vi "XML Results.vi"(2 "XML":string="﻿<?xml version=\"1.0\" encoding=\"UTF-8\" standalone=\"no\"?><worksheet xmlns=\"http://schemas.mathsoft.com/worksheet50\" xmlns:xsi=\"http://www.w3.org/2001/XMLSchema-instance\" xmlns:ve=\"http://schemas.openxmlformats.org/markup-compatibility/2006\" xmlns:r=\"http://schemas.openxmlformats.org/officeDocument/2006/relationships\" xmlns:ws=\"http://schemas.mathsoft.com/worksheet50\" xmlns:ml=\"http://schemas.mathsoft.com/math50\" xmlns:u=\"http://schemas.mathsoft.com/units10\" xmlns:p=\"http://schemas.mathsoft.com/provenance10\"><regions><region top=\"57.6\" width=\"368\" left=\"9.6\" height=\"30\" converted-from=\"Mathcad14\" region-id=\"0\"><text><FlowDocument FontFamily=\"Tahoma\" FontStyle=\"Normal\" FontWeight=\"Normal\" FontSize=\"14.6666666666667\" Foreground=\"#FF000000\" Background=\"#00FFFFFF\" PagePadding=\"5,0,5,0\" AllowDrop=\"True\" Typography.Variants=\"Normal\" xmlns=\"http://schemas.microsoft.com/winfx/2006/xaml/presentation\"><Paragraph TextAlignment=\"Left\"><Run FontFamily=\"Arial\" FontStyle=\"Normal\" FontWeight=\"Bold\" FontSize=\"26.6666666666667\" Typography.Variants=\"Normal\"><Run.TextDecorations><TextDecoration Location=\"Underline\" /></Run.TextDecorations>AguaClara Design Tool</Run></Paragraph></FlowDocument></text></region><region top=\"124.8\" width=\"75\" left=\"48\" height=\"17\" converted-from=\"Mathcad14\" region-id=\"1\"><math><ml:eval><ml:id xml:space=\"preserve\">Country</ml:id><ml:result /></ml:eval></math></region><region top=\"153.6\" width=\"84\" left=\"48\" height=\"17\" converted-from=\"Mathcad14\" region-id=\"2\"><math><ml:eval><ml:id xml:space=\"preserve\">Language</ml:id><ml:result /></ml:eval></math></region><region top=\"153.6\" width=\"152\" left=\"288\" height=\"37\" converted-from=\"Mathcad14\" region-id=\"3\"><math><ml:define><ml:id label=\"Variable\" xml:space=\"preserve\"><Span xmlns=\"http://schemas.microsoft.com/winfx/2006/xaml/presentation\" xmlns:pw=\"clr-namespace:Ptc.Wpf;assembly=Ptc.Core\">C<pw:Subscript>ChlorineDoseMax</pw:Subscript></Span></ml:id><ml:apply><ml:mult /><ml:real>2</ml:real><ml:apply><ml:div /><ml:id xml:space=\"preserve\">mg</ml:id><ml:id xml:space=\"preserve\">L</ml:id></ml:apply></ml:apply></ml:define></math><mc14-conversion-loss-annotations><annotation>DisplayOperator</annotation></mc14-conversion-loss-annotations></region><region top=\"201.6\" width=\"138\" left=\"288\" height=\"37\" converted-from=\"Mathcad14\" region-id=\"4\"><math><ml:define><ml:id label=\"Variable\" xml:space=\"preserve\"><Span xmlns=\"http://schemas.microsoft.com/winfx/2006/xaml/presentation\" xmlns:pw=\"clr-namespace:Ptc.Wpf;assembly=Ptc.Core\">C<pw:Subscript>ChlorineStock</pw:Subscript></Span></ml:id><ml:apply><ml:mult /><ml:real>50</ml:real><ml:apply><ml:div /><ml:id xml:space=\"preserve\">gm</ml:id><ml:id xml:space=\"preserve\">L</ml:id></ml:apply></ml:apply></ml:define></math><mc14-conversion-loss-annotations><annotation>DisplayOperator</annotation></mc14-conversion-loss-annotations></region><region top=\"240\" width=\"131\" left=\"288\" height=\"22\" converted-from=\"Mathcad14\" region-id=\"5\"><math><ml:define><ml:id label=\"Variable\" xml:space=\"preserve\"><Span xmlns=\"http://schemas.microsoft.com/winfx/2006/xaml/presentation\" xmlns:pw=\"clr-namespace:Ptc.Wpf;assembly=Ptc.Core\">Ti<pw:Subscript>ChlorineStock</pw:Subscript></Span></ml:id><ml:apply><ml:mult /><ml:real>30</ml:real><ml:id xml:space=\"preserve\">hr</ml:id></ml:apply></ml:define></math><mc14-conversion-loss-annotations><annotation>DisplayOperator</annotation></mc14-conversion-loss-annotations></region><region top=\"268.8\" width=\"242.68\" left=\"422.4\" height=\"32\" converted-from=\"Mathcad14\" region-id=\"6\"><text><FlowDocument FontFamily=\"Tahoma\" FontStyle=\"Normal\" FontWeight=\"Normal\" FontSize=\"14.6666666666667\" Foreground=\"#FF000000\" Background=\"#00FFFFFF\" PagePadding=\"5,0,5,0\" AllowDrop=\"True\" Typography.Variants=\"Normal\" xmlns=\"http://schemas.microsoft.com/winfx/2006/xaml/presentation\"><Paragraph TextAlignment=\"Left\"><Run FontFamily=\"Arial\" FontStyle=\"Normal\" FontWeight=\"Normal\" FontSize=\"13.3333333333333\" Typography.Variants=\"Normal\"><Run.TextDecorations><TextDecorationCollection /></Run.TextDecorations>Needs to be redefined as zero until we create a database for all countries.</Run></Paragraph></FlowDocument></text></region><region top=\"278.4\" width=\"70\" left=\"288\" height=\"17\" converted-from=\"Mathcad14\" region-id=\"7\"><math><ml:define><ml:id label=\"Variable\" xml:space=\"preserve\">Country</ml:id><ml:real>0</ml:real></ml:define></math></region><region top=\"297.6\" width=\"172\" left=\"9.6\" height=\"24\" converted-from=\"Mathcad14\" region-id=\"8\"><text><FlowDocument FontFamily=\"Tahoma\" FontStyle=\"Normal\" FontWeight=\"Normal\" FontSize=\"14.6666666666667\" Foreground=\"#FF000000\" Background=\"#00FFFFFF\" PagePadding=\"5,0,5,0\" AllowDrop=\"True\" Typography.Variants=\"Normal\" xmlns=\"http://schemas.microsoft.com/winfx/2006/xaml/presentation\"><Paragraph TextAlignment=\"Left\"><Run FontFamily=\"Arial\" FontStyle=\"Normal\" FontWeight=\"Normal\" FontSize=\"21.3333333333333\" Typography.Variants=\"Normal\"><Run.TextDecorations><TextDecorationCollection /></Run.TextDecorations>References</Run></Paragraph></FlowDocument></text></region><region top=\"326.4\" width=\"832\" left=\"0\" height=\"19.2\" region-id=\"9\"><text is-text-block=\"true\"><FlowDocument FontFamily=\"Mathcad UniMath\" xmlns=\"http://schemas.microsoft.com/winfx/2006/xaml/presentation\"><Paragraph xml:space=\"preserve\">---↓  ---</Paragraph></FlowDocument></text><mc14-conversion-loss-annotations><annotation>Area</annotation></mc14-conversion-loss-annotations></region><region top=\"378.24\" width=\"215.68\" left=\"28.8\" height=\"16\" converted-from=\"Mathcad14\" region-id=\"10\"><text><FlowDocument FontFamily=\"Tahoma\" FontStyle=\"Normal\" FontWeight=\"Normal\" FontSize=\"14.6666666666667\" Foreground=\"#FF000000\" Background=\"#00FFFFFF\" PagePadding=\"5,0,5,0\" AllowDrop=\"True\" Typography.Variants=\"Normal\" xmlns=\"http://schemas.microsoft.com/winfx/2006/xaml/presentation\"><Paragraph TextAlignment=\"Left\"><Run FontFamily=\"Arial\" FontStyle=\"Normal\" FontWeight=\"Normal\" FontSize=\"13.3333333333333\" Typography.Variants=\"Normal\"><Run.TextDecorations><TextDecorationCollection /></Run.TextDecorations>MathCAD dimension calculations:</Run></Paragraph></FlowDocument></text></region><region top=\"416.639984\" width=\"488\" left=\"48\" height=\"14\" converted-from=\"Mathcad14\" region-id=\"11\"><reference used-cache=\"false\" last-saved-date=\"12/31/9999 23:59:59\" href=\"./BasicClientInputs.mcdx\" /><mc14-conversion-loss-annotations><annotation>IncludeWorksheet</annotation></mc14-conversion-loss-annotations></region><region top=\"435.84\" width=\"461\" left=\"48\" height=\"14\" converted-from=\"Mathcad14\" region-id=\"12\"><reference used-cache=\"false\" last-saved-date=\"12/31/9999 23:59:59\" href=\"./ExpertInputs.mcdx\" /><mc14-conversion-loss-annotations><annotation>IncludeWorksheet</annotation></mc14-conversion-loss-annotations></region><region top=\"455.039978\" width=\"476\" left=\"48\" height=\"14\" converted-from=\"Mathcad14\" region-id=\"13\"><reference used-cache=\"false\" last-saved-date=\"12/31/9999 23:59:59\" href=\"./MathFunctions.mcdx\" /><mc14-conversion-loss-annotations><annotation>IncludeWorksheet</annotation></mc14-conversion-loss-annotations></region><region top=\"474.24\" width=\"466\" left=\"48\" height=\"14\" converted-from=\"Mathcad14\" region-id=\"14\"><reference used-cache=\"false\" last-saved-date=\"12/31/9999 23:59:59\" href=\"./PipeDatabase.mcdx\" /><mc14-conversion-loss-annotations><annotation>IncludeWorksheet</annotation></mc14-conversion-loss-annotations></region><region top=\"493.44\" width=\"480\" left=\"48\" height=\"14\" converted-from=\"Mathcad14\" region-id=\"15\"><reference used-cache=\"false\" last-saved-date=\"12/31/9999 23:59:59\" href=\"./FluidsFunctions.mcdx\" /><mc14-conversion-loss-annotations><annotation>IncludeWorksheet</annotation></mc14-conversion-loss-annotations></region><region top=\"512.64\" width=\"496\" left=\"48\" height=\"14\" converted-from=\"Mathcad14\" region-id=\"16\"><reference used-cache=\"false\" last-saved-date=\"12/31/9999 23:59:59\" href=\"./SedimentationTank.mcdx\" /><mc14-conversion-loss-annotations><annotation>IncludeWorksheet</annotation></mc14-conversion-loss-annotations></region><region top=\"531.839966\" width=\"453\" left=\"48\" height=\"14\" converted-from=\"Mathcad14\" region-id=\"17\"><reference used-cache=\"false\" last-saved-date=\"12/31/9999 23:59:59\" href=\"./Flocculator.mcdx\" /><mc14-conversion-loss-annotations><annotation>IncludeWorksheet</annotation></mc14-conversion-loss-annotations></region><region top=\"551.04\" width=\"428\" left=\"48\" height=\"14\" converted-from=\"Mathcad14\" region-id=\"18\"><reference used-cache=\"false\" last-saved-date=\"12/31/9999 23:59:59\" href=\"./LFOM.mcdx\" /><mc14-conversion-loss-annotations><annotation>IncludeWorksheet</annotation></mc14-conversion-loss-annotations></region><region top=\"570.24\" width=\"447\" left=\"48\" height=\"14\" converted-from=\"Mathcad14\" region-id=\"19\"><reference used-cache=\"false\" last-saved-date=\"12/31/9999 23:59:59\" href=\"./LinearCdc.mcdx\" /><mc14-conversion-loss-annotations><annotation>IncludeWorksheet</annotation></mc14-conversion-loss-annotations></region><region top=\"589.44\" width=\"497\" left=\"48\" height=\"14\" converted-from=\"Mathcad14\" region-id=\"20\"><reference used-cache=\"false\" last-saved-date=\"12/31/9999 23:59:59\" href=\"./ChemStorageTanks.mcdx\" /><mc14-conversion-loss-annotations><annotation>IncludeWorksheet</annotation></mc14-conversion-loss-annotations></region><region top=\"608.64\" width=\"467\" left=\"48\" height=\"14\" converted-from=\"Mathcad14\" region-id=\"21\"><reference used-cache=\"false\" last-saved-date=\"12/31/9999 23:59:59\" href=\"./EntranceTank.mcdx\" /><mc14-conversion-loss-annotations><annotation>IncludeWorksheet</annotation></mc14-conversion-loss-annotations></region><region top=\"627.839966\" width=\"520\" left=\"48\" height=\"14\" converted-from=\"Mathcad14\" region-id=\"22\"><reference used-cache=\"false\" last-saved-date=\"12/31/9999 23:59:59\" href=\"./StackedRapidSandFilter.mcdx\" /><mc14-conversion-loss-annotations><annotation>IncludeWorksheet</annotation></mc14-conversion-loss-annotations></region><region top=\"647.04\" width=\"466\" left=\"48\" height=\"14\" converted-from=\"Mathcad14\" region-id=\"23\"><reference used-cache=\"false\" last-saved-date=\"12/31/9999 23:59:59\" href=\"./DrainChannel.mcdx\" /><mc14-conversion-loss-annotations><annotation>IncludeWorksheet</annotation></mc14-conversion-loss-annotations></region><region top=\"666.24\" width=\"463\" left=\"48\" height=\"14\" converted-from=\"Mathcad14\" region-id=\"24\"><reference used-cache=\"false\" last-saved-date=\"12/31/9999 23:59:59\" href=\"./MaterialsList.mcdx\" /><mc14-conversion-loss-annotations><annotation>IncludeWorksheet</annotation></mc14-conversion-loss-annotations></region><region top=\"704.64\" width=\"187.68\" left=\"28.8\" height=\"16\" converted-from=\"Mathcad14\" region-id=\"25\"><text><FlowDocument FontFamily=\"Tahoma\" FontStyle=\"Normal\" FontWeight=\"Normal\" FontSize=\"14.6666666666667\" Foreground=\"#FF000000\" Background=\"#00FFFFFF\" PagePadding=\"5,0,5,0\" AllowDrop=\"True\" Typography.Variants=\"Normal\" xmlns=\"http://schemas.microsoft.com/winfx/2006/xaml/presentation\"><Paragraph TextAlignment=\"Left\"><Run FontFamily=\"Arial\" FontStyle=\"Normal\" FontWeight=\"Normal\" FontSize=\"13.3333333333333\" Typography.Variants=\"Normal\"><Run.TextDecorations><TextDecorationCollection /></Run.TextDecorations>AutoCAD drawing programs:</Run></Paragraph></FlowDocument></text></region><region top=\"743.04\" width=\"125\" left=\"57.6\" height=\"18\" converted-from=\"Mathcad14\" region-id=\"26\"><text><FlowDocument FontFamily=\"Tahoma\" FontStyle=\"Normal\" FontWeight=\"Normal\" FontSize=\"14.6666666666667\" Foreground=\"#FF000000\" Background=\"#00FFFFFF\" PagePadding=\"5,0,5,0\" AllowDrop=\"True\" Typography.Variants=\"Normal\" xmlns=\"http://schemas.microsoft.com/winfx/2006/xaml/presentation\"><Paragraph TextAlignment=\"Left\"><Run FontFamily=\"Arial\" FontStyle=\"Normal\" FontWeight=\"Normal\" FontSize=\"16\" Typography.Variants=\"Normal\"><Run.TextDecorations><TextDecoration Location=\"Underline\" /></Run.TextDecorations>Translators:</Run><Run FontFamily=\"Arial\" FontStyle=\"Normal\" FontWeight=\"Normal\" FontSize=\"13.3333333333333\" Typography.Variants=\"Normal\" xml:space=\"preserve\"><Run.TextDecorations><TextDecorationCollection /></Run.TextDecorations> </Run></Paragraph></FlowDocument></text></region><region top=\"771.839966\" width=\"534\" left=\"57.6\" height=\"32\" converted-from=\"Mathcad14\" region-id=\"27\"><text><FlowDocument FontFamily=\"Tahoma\" FontStyle=\"Normal\" FontWeight=\"Normal\" FontSize=\"14.6666666666667\" Foreground=\"#FF000000\" Background=\"#00FFFFFF\" PagePadding=\"5,0,5,0\" AllowDrop=\"True\" Typography.Variants=\"Normal\" xmlns=\"http://schemas.microsoft.com/winfx/2006/xaml/presentation\"><Paragraph TextAlignment=\"Left\"><Run FontFamily=\"Arial\" FontStyle=\"Normal\" FontWeight=\"Normal\" FontSize=\"13.3333333333333\" Typography.Variants=\"Normal\"><Run.TextDecorations><TextDecorationCollection /></Run.TextDecorations>These are the codes that take MathCAD outputs and create AutoCAD scripts that are used to draw the plant (formerly Basics)</Run></Paragraph></FlowDocument></text></region><region top=\"800.64\" width=\"586\" left=\"48\" height=\"14\" converted-from=\"Mathcad14\" region-id=\"28\"><reference used-cache=\"false\" last-saved-date=\"12/31/9999 23:59:59\" href=\".\\AutoCAD Scripts\\MtoATranslators.mcdx\" /><mc14-conversion-loss-annotations><annotation>IncludeWorksheet</annotation></mc14-conversion-loss-annotations></region><region top=\"848.64\" width=\"558\" left=\"57.6\" height=\"64\" converted-from=\"Mathcad14\" region-id=\"29\"><text><FlowDocument FontFamily=\"Tahoma\" FontStyle=\"Normal\" FontWeight=\"Normal\" FontSize=\"14.6666666666667\" Foreground=\"#FF000000\" Background=\"#00FFFFFF\" PagePadding=\"5,0,5,0\" AllowDrop=\"True\" Typography.Variants=\"Normal\" xmlns=\"http://schemas.microsoft.com/winfx/2006/xaml/presentation\"><Paragraph TextAlignment=\"Left\"><Run FontFamily=\"Arial\" FontStyle=\"Normal\" FontWeight=\"Normal\" FontSize=\"13.3333333333333\" Typography.Variants=\"Normal\"><Run.TextDecorations><TextDecorationCollection /></Run.TextDecorations>The wrapped MtoA translator contains the functions that the user will want to access. These functions will draw pieces with full functionality - specifying the location, dimension, and orientation of the object. Also, it contains layer control and subtraction capabilities for grouped objects.</Run></Paragraph></FlowDocument></text></region><region top=\"915.84\" width=\"636\" left=\"48\" height=\"14\" converted-from=\"Mathcad14\" region-id=\"30\"><reference used-cache=\"false\" last-saved-date=\"12/31/9999 23:59:59\" href=\".\\AutoCAD Scripts\\MtoATranslatorsWrapped.mcdx\" /><mc14-conversion-loss-annotations><annotation>IncludeWorksheet</annotation></mc14-conversion-loss-annotations></region><region top=\"992.64\" width=\"172\" left=\"19.2\" height=\"18\" converted-from=\"Mathcad14\" region-id=\"31\"><text><FlowDocument FontFamily=\"Tahoma\" FontStyle=\"Normal\" FontWeight=\"Normal\" FontSize=\"14.6666666666667\" Foreground=\"#FF000000\" Background=\"#00FFFFFF\" PagePadding=\"5,0,5,0\" AllowDrop=\"True\" Typography.Variants=\"Normal\" xmlns=\"http://schemas.microsoft.com/winfx/2006/xaml/presentation\"><Paragraph TextAlignment=\"Left\"><Run FontFamily=\"Arial\" FontStyle=\"Normal\" FontWeight=\"Normal\" FontSize=\"16\" Typography.Variants=\"Normal\"><Run.TextDecorations><TextDecoration Location=\"Underline\" /></Run.TextDecorations>Drawing functions:</Run><Run FontFamily=\"Arial\" FontStyle=\"Normal\" FontWeight=\"Normal\" FontSize=\"13.3333333333333\" Typography.Variants=\"Normal\" xml:space=\"preserve\"><Run.TextDecorations><TextDecorationCollection /></Run.TextDecorations> </Run></Paragraph></FlowDocument></text></region><region top=\"1011.84\" width=\"543\" left=\"48\" height=\"14\" converted-from=\"Mathcad14\" region-id=\"32\"><reference used-cache=\"false\" last-saved-date=\"12/31/9999 23:59:59\" href=\".\\AutoCAD Scripts\\ChannelF.mcdx\" /><mc14-conversion-loss-annotations><annotation>IncludeWorksheet</annotation></mc14-conversion-loss-annotations></region><region top=\"1031.04\" width=\"549\" left=\"48\" height=\"14\" converted-from=\"Mathcad14\" region-id=\"33\"><reference used-cache=\"false\" last-saved-date=\"12/31/9999 23:59:59\" href=\".\\AutoCAD Scripts\\PlumbingF.mcdx\" /><mc14-conversion-loss-annotations><annotation>IncludeWorksheet</annotation></mc14-conversion-loss-annotations></region><region top=\"1050.24\" width=\"526\" left=\"48\" height=\"14\" converted-from=\"Mathcad14\" region-id=\"34\"><reference used-cache=\"false\" last-saved-date=\"12/31/9999 23:59:59\" href=\".\\AutoCAD Scripts\\TankF.mcdx\" /><mc14-conversion-loss-annotations><annotation>IncludeWorksheet</annotation></mc14-conversion-loss-annotations></region><region top=\"1069.44006\" width=\"529\" left=\"48\" height=\"14\" converted-from=\"Mathcad14\" region-id=\"35\"><reference used-cache=\"false\" last-saved-date=\"12/31/9999 23:59:59\" href=\".\\AutoCAD Scripts\\StairsF.mcdx\" /><mc14-conversion-loss-annotations><annotation>IncludeWorksheet</annotation></mc14-conversion-loss-annotations></region><region top=\"1088.64\" width=\"572\" left=\"48\" height=\"14\" converted-from=\"Mathcad14\" region-id=\"36\"><reference used-cache=\"false\" last-saved-date=\"12/31/9999 23:59:59\" href=\".\\AutoCAD Scripts\\DrainChannelF.mcdx\" /><mc14-conversion-loss-annotations><annotation>IncludeWorksheet</annotation></mc14-conversion-loss-annotations></region><region top=\"1165.44006\" width=\"184\" left=\"19.2\" height=\"18\" converted-from=\"Mathcad14\" region-id=\"37\"><text><FlowDocument FontFamily=\"Tahoma\" FontStyle=\"Normal\" FontWeight=\"Normal\" FontSize=\"14.6666666666667\" Foreground=\"#FF000000\" Background=\"#00FFFFFF\" PagePadding=\"5,0,5,0\" AllowDrop=\"True\" Typography.Variants=\"Normal\" xmlns=\"http://schemas.microsoft.com/winfx/2006/xaml/presentation\"><Paragraph TextAlignment=\"Left\"><Run FontFamily=\"Arial\" FontStyle=\"Normal\" FontWeight=\"Normal\" FontSize=\"16\" Typography.Variants=\"Normal\"><Run.TextDecorations><TextDecoration Location=\"Underline\" /></Run.TextDecorations>AutoCAD Script Files:</Run><Run FontFamily=\"Arial\" FontStyle=\"Normal\" FontWeight=\"Normal\" FontSize=\"13.3333333333333\" Typography.Variants=\"Normal\" xml:space=\"preserve\"><Run.TextDecorations><TextDecorationCollection /></Run.TextDecorations> </Run></Paragraph></FlowDocument></text></region><region top=\"1184.64\" width=\"570\" left=\"48\" height=\"14\" converted-from=\"Mathcad14\" region-id=\"38\"><reference used-cache=\"false\" last-saved-date=\"12/31/9999 23:59:59\" href=\".\\AutoCAD Scripts\\FlocculatorAC.mcdx\" /><mc14-conversion-loss-annotations><annotation>IncludeWorksheet</annotation></mc14-conversion-loss-annotations></region><region top=\"1203.84009\" width=\"613\" left=\"48\" height=\"14\" converted-from=\"Mathcad14\" region-id=\"39\"><reference used-cache=\"false\" last-saved-date=\"12/31/9999 23:59:59\" href=\".\\AutoCAD Scripts\\SedimentationTankAC.mcdx\" /><mc14-conversion-loss-annotations><annotation>IncludeWorksheet</annotation></mc14-conversion-loss-annotations></region><region top=\"1223.04\" width=\"584\" left=\"48\" height=\"14\" converted-from=\"Mathcad14\" region-id=\"40\"><reference used-cache=\"false\" last-saved-date=\"12/31/9999 23:59:59\" href=\".\\AutoCAD Scripts\\EntranceTankAC.mcdx\" /><mc14-conversion-loss-annotations><annotation>IncludeWorksheet</annotation></mc14-conversion-loss-annotations></region><region top=\"1242.24\" width=\"631\" left=\"48\" height=\"14\" converted-from=\"Mathcad14\" region-id=\"41\"><reference used-cache=\"false\" last-saved-date=\"12/31/9999 23:59:59\" href=\".\\AutoCAD Scripts\\ChemStockTanksACvlk24.mcdx\" /><mc14-conversion-loss-annotations><annotation>IncludeWorksheet</annotation></mc14-conversion-loss-annotations></region><region top=\"1261.44006\" width=\"583\" left=\"48\" height=\"14\" converted-from=\"Mathcad14\" region-id=\"42\"><reference used-cache=\"false\" last-saved-date=\"12/31/9999 23:59:59\" href=\".\\AutoCAD Scripts\\DrainChannelAC.mcdx\" /><mc14-conversion-loss-annotations><annotation>IncludeWorksheet</annotation></mc14-conversion-loss-annotations></region><region top=\"1280.64\" width=\"637\" left=\"48\" height=\"14\" converted-from=\"Mathcad14\" region-id=\"43\"><reference used-cache=\"false\" last-saved-date=\"12/31/9999 23:59:59\" href=\".\\AutoCAD Scripts\\StackedRapidSandFilterAC.mcdx\" /><mc14-conversion-loss-annotations><annotation>IncludeWorksheet</annotation></mc14-conversion-loss-annotations></region><region top=\"1299.84009\" width=\"559\" left=\"48\" height=\"14\" converted-from=\"Mathcad14\" region-id=\"44\"><reference used-cache=\"false\" last-saved-date=\"12/31/9999 23:59:59\" href=\".\\AutoCAD Scripts\\CdcACvlk24.mcdx\" /><mc14-conversion-loss-annotations><annotation>IncludeWorksheet</annotation></mc14-conversion-loss-annotations></region><region top=\"1319.04\" width=\"625\" left=\"48\" height=\"14\" converted-from=\"Mathcad14\" region-id=\"45\"><reference used-cache=\"false\" last-saved-date=\"12/31/9999 23:59:59\" href=\".\\AutoCAD Scripts\\OperatorAccessACvlk24.mcdx\" /><mc14-conversion-loss-annotations><annotation>IncludeWorksheet</annotation></mc14-conversion-loss-annotations></region><region top=\"1338.24\" width=\"560\" left=\"48\" height=\"14\" converted-from=\"Mathcad14\" region-id=\"46\"><reference used-cache=\"false\" last-saved-date=\"12/31/9999 23:59:59\" href=\".\\AutoCAD Scripts\\MaterialsAC.mcdx\" /><mc14-conversion-loss-annotations><annotation>IncludeWorksheet</annotation></mc14-conversion-loss-annotations></region><region top=\"1424.64\" width=\"77.08\" left=\"19.2\" height=\"18\" converted-from=\"Mathcad14\" region-id=\"47\"><text><FlowDocument FontFamily=\"Tahoma\" FontStyle=\"Normal\" FontWeight=\"Normal\" FontSize=\"14.6666666666667\" Foreground=\"#FF000000\" Background=\"#00FFFFFF\" PagePadding=\"5,0,5,0\" AllowDrop=\"True\" Typography.Variants=\"Normal\" xmlns=\"http://schemas.microsoft.com/winfx/2006/xaml/presentation\"><Paragraph TextAlignment=\"Left\"><Run FontFamily=\"Arial\" FontStyle=\"Normal\" FontWeight=\"Normal\" FontSize=\"16\" Typography.Variants=\"Normal\"><Run.TextDecorations><TextDecoration Location=\"Underline\" /></Run.TextDecorations>Layouts:</Run></Paragraph></FlowDocument></text></region><region top=\"1472.64\" width=\"297.76\" left=\"57.6\" height=\"16\" converted-from=\"Mathcad14\" region-id=\"48\"><text><FlowDocument FontFamily=\"Tahoma\" FontStyle=\"Normal\" FontWeight=\"Normal\" FontSize=\"14.6666666666667\" Foreground=\"#FF000000\" Background=\"#00FFFFFF\" PagePadding=\"5,0,5,0\" AllowDrop=\"True\" Typography.Variants=\"Normal\" xmlns=\"http://schemas.microsoft.com/winfx/2006/xaml/presentation\"><Paragraph TextAlignment=\"Left\"><Run FontFamily=\"Arial\" FontStyle=\"Normal\" FontWeight=\"Normal\" FontSize=\"13.3333333333333\" Typography.Variants=\"Normal\"><Run.TextDecorations><TextDecorationCollection /></Run.TextDecorations>This rearranges the plant to optimize the layout</Run></Paragraph></FlowDocument></text></region><region top=\"1491.84009\" width=\"581\" left=\"57.6\" height=\"14\" converted-from=\"Mathcad14\" region-id=\"49\"><reference used-cache=\"false\" last-saved-date=\"12/31/9999 23:59:59\" href=\".\\AutoCAD Scripts\\PlantLayoutsAC.mcdx\" /><mc14-conversion-loss-annotations><annotation>IncludeWorksheet</annotation></mc14-conversion-loss-annotations></region><region top=\"1549.44006\" width=\"466\" left=\"38.4\" height=\"32\" converted-from=\"Mathcad14\" region-id=\"50\"><text><FlowDocument FontFamily=\"Tahoma\" FontStyle=\"Normal\" FontWeight=\"Normal\" FontSize=\"14.6666666666667\" Foreground=\"#FF000000\" Background=\"#00FFFFFF\" PagePadding=\"5,0,5,0\" AllowDrop=\"True\" Typography.Variants=\"Normal\" xmlns=\"http://schemas.microsoft.com/winfx/2006/xaml/presentation\"><Paragraph TextAlignment=\"Left\"><Run FontFamily=\"Arial\" FontStyle=\"Normal\" FontWeight=\"Normal\" FontSize=\"13.3333333333333\" Typography.Variants=\"Normal\"><Run.TextDecorations><TextDecorationCollection /></Run.TextDecorations>This file will execute at the very end to create multiple views of the entire plant in paperspace</Run></Paragraph></FlowDocument></text></region><region top=\"1587.84009\" width=\"554\" left=\"48\" height=\"14\" converted-from=\"Mathcad14\" region-id=\"51\"><reference used-cache=\"false\" last-saved-date=\"12/31/9999 23:59:59\" href=\".\\AutoCAD Scripts\\LayoutsAC.mcdx\" /><mc14-conversion-loss-annotations><annotation>IncludeWorksheet</annotation></mc14-conversion-loss-annotations></region><region top=\"1687.44006\" width=\"832\" left=\"0\" height=\"19.2\" region-id=\"52\"><text is-text-block=\"true\"><FlowDocument FontFamily=\"Mathcad UniMath\" xmlns=\"http://schemas.microsoft.com/winfx/2006/xaml/presentation\"><Paragraph xml:space=\"preserve\">---↑  ---</Paragraph></FlowDocument></text></region><region top=\"1726.08008\" width=\"567\" left=\"19.2\" height=\"36\" converted-from=\"Mathcad14\" region-id=\"53\"><text><FlowDocument FontFamily=\"Tahoma\" FontStyle=\"Normal\" FontWeight=\"Normal\" FontSize=\"14.6666666666667\" Foreground=\"#FF000000\" Background=\"#00FFFFFF\" PagePadding=\"5,0,5,0\" AllowDrop=\"True\" Typography.Variants=\"Normal\" xmlns=\"http://schemas.microsoft.com/winfx/2006/xaml/presentation\"><Paragraph TextAlignment=\"Left\"><Run FontFamily=\"Arial\" FontStyle=\"Italic\" FontWeight=\"Bold\" FontSize=\"16\" Typography.Variants=\"Normal\" xml:space=\"preserve\"><Run.TextDecorations><TextDecorationCollection /></Run.TextDecorations>All variables displayed must have the standard SI units. They may not have units attached by the user. </Run></Paragraph></FlowDocument></text></region><region top=\"1850.88013\" width=\"301\" left=\"9.6\" height=\"19\" converted-from=\"Mathcad14\" region-id=\"54\"><text><FlowDocument FontFamily=\"Tahoma\" FontStyle=\"Normal\" FontWeight=\"Normal\" FontSize=\"14.6666666666667\" Foreground=\"#FF000000\" Background=\"#00FFFFFF\" PagePadding=\"5,0,5,0\" AllowDrop=\"True\" Typography.Variants=\"Normal\" xmlns=\"http://schemas.microsoft.com/winfx/2006/xaml/presentation\"><Paragraph TextAlignment=\"Left\"><Run FontFamily=\"Arial\" FontStyle=\"Normal\" FontWeight=\"Bold\" FontSize=\"16\" Foreground=\"#FF008000\" Typography.Variants=\"Normal\"><Run.TextDecorations><TextDecorationCollection /></Run.TextDecorations>General</Run></Paragraph></FlowDocument></text></region><region top=\"1860.4801\" width=\"832\" left=\"0\" height=\"19.2\" region-id=\"55\"><text is-text-block=\"true\"><FlowDocument FontFamily=\"Mathcad UniMath\" xmlns=\"http://schemas.microsoft.com/winfx/2006/xaml/presentation\"><Paragraph xml:space=\"preserve\">---↓  ---</Paragraph></FlowDocument></text><mc14-conversion-loss-annotations><annotation>CollapsedArea</annotation></mc14-conversion-loss-annotations></region><region top=\"1950.72009\" width=\"67\" left=\"38.4\" height=\"22\" converted-from=\"Mathcad14\" region-id=\"56\"><math><ml:eval><ml:id xml:space=\"preserve\"><Span xmlns=\"http://schemas.microsoft.com/winfx/2006/xaml/presentation\" xmlns:pw=\"clr-namespace:Ptc.Wpf;assembly=Ptc.Core\">Q<pw:Subscript>Plant</pw:Subscript></Span></ml:id><ml:result /></ml:eval></math></region><region top=\"1950.72009\" width=\"170\" left=\"345.6\" height=\"22\" converted-from=\"Mathcad14\" region-id=\"57\"><math resultRef=\"-2\"><ml:eval><ml:id xml:space=\"preserve\"><Span xmlns=\"http://schemas.microsoft.com/winfx/2006/xaml/presentation\" xmlns:pw=\"clr-namespace:Ptc.Wpf;assembly=Ptc.Core\">Pi<pw:Subscript>VenaContractaOrifice</pw:Subscript></Span></ml:id><ml:result /></ml:eval></math></region><region top=\"1998.72009\" width=\"92\" left=\"48\" height=\"22\" converted-from=\"Mathcad14\" region-id=\"58\"><math><ml:eval><ml:id xml:space=\"preserve\"><Span xmlns=\"http://schemas.microsoft.com/winfx/2006/xaml/presentation\" xmlns:pw=\"clr-namespace:Ptc.Wpf;assembly=Ptc.Core\">T<pw:Subscript>PlantWall</pw:Subscript></Span></ml:id><ml:result /></ml:eval></math></region><region top=\"2037.12012\" width=\"90\" left=\"364.8\" height=\"22\" converted-from=\"Mathcad14\" region-id=\"59\"><math><ml:eval><ml:id xml:space=\"preserve\"><Span xmlns=\"http://schemas.microsoft.com/winfx/2006/xaml/presentation\" xmlns:pw=\"clr-namespace:Ptc.Wpf;assembly=Ptc.Core\">W<pw:Subscript>SedPlate</pw:Subscript></Span></ml:id><ml:result /></ml:eval></math></region><region top=\"2046.72009\" width=\"109\" left=\"48\" height=\"22\" converted-from=\"Mathcad14\" region-id=\"60\"><math><ml:eval><ml:id xml:space=\"preserve\"><Span xmlns=\"http://schemas.microsoft.com/winfx/2006/xaml/presentation\" xmlns:pw=\"clr-namespace:Ptc.Wpf;assembly=Ptc.Core\">T<pw:Subscript>ConcreteMin</pw:Subscript></Span></ml:id><ml:result /></ml:eval></math></region><region top=\"2085.12\" width=\"114\" left=\"364.8\" height=\"22\" converted-from=\"Mathcad14\" region-id=\"61\"><math><ml:eval><ml:id xml:space=\"preserve\"><Span xmlns=\"http://schemas.microsoft.com/winfx/2006/xaml/presentation\" xmlns:pw=\"clr-namespace:Ptc.Wpf;assembly=Ptc.Core\">L<pw:Subscript>SedPlateSheet</pw:Subscript></Span></ml:id><ml:result /></ml:eval></math></region><region top=\"2094.72021\" width=\"98\" left=\"48\" height=\"22\" converted-from=\"Mathcad14\" region-id=\"62\"><math><ml:eval><ml:id xml:space=\"preserve\"><Span xmlns=\"http://schemas.microsoft.com/winfx/2006/xaml/presentation\" xmlns:pw=\"clr-namespace:Ptc.Wpf;assembly=Ptc.Core\">C<pw:Subscript>CoagStock</pw:Subscript></Span></ml:id><ml:result /></ml:eval></math></region><region top=\"2133.12\" width=\"85\" left=\"364.8\" height=\"22\" converted-from=\"Mathcad14\" region-id=\"63\"><math><ml:eval><ml:id xml:space=\"preserve\"><Span xmlns=\"http://schemas.microsoft.com/winfx/2006/xaml/presentation\" xmlns:pw=\"clr-namespace:Ptc.Wpf;assembly=Ptc.Core\">T<pw:Subscript>SedPlate</pw:Subscript></Span></ml:id><ml:result /></ml:eval></math></region><region top=\"2161.92017\" width=\"101\" left=\"48\" height=\"22\" converted-from=\"Mathcad14\" region-id=\"64\"><math><ml:eval><ml:id xml:space=\"preserve\"><Span xmlns=\"http://schemas.microsoft.com/winfx/2006/xaml/presentation\" xmlns:pw=\"clr-namespace:Ptc.Wpf;assembly=Ptc.Core\">Ti<pw:Subscript>CoagStock</pw:Subscript></Span></ml:id><ml:result /></ml:eval></math></region><region top=\"2181.12\" width=\"86\" left=\"364.8\" height=\"22\" converted-from=\"Mathcad14\" region-id=\"65\"><math><ml:eval><ml:id xml:space=\"preserve\"><Span xmlns=\"http://schemas.microsoft.com/winfx/2006/xaml/presentation\" xmlns:pw=\"clr-namespace:Ptc.Wpf;assembly=Ptc.Core\">T<pw:Subscript>SedWeir</pw:Subscript></Span></ml:id><ml:result /></ml:eval></math></region><region top=\"2209.92017\" width=\"142\" left=\"48\" height=\"45\" converted-from=\"Mathcad14\" region-id=\"66\"><math resultRef=\"-3\"><ml:eval><ml:id xml:space=\"preserve\"><Span xmlns=\"http://schemas.microsoft.com/winfx/2006/xaml/presentation\" xmlns:pw=\"clr-namespace:Ptc.Wpf;assembly=Ptc.Core\">C<pw:Subscript>ChlorineStock</pw:Subscript></Span></ml:id><ml:result /></ml:eval></math></region><region top=\"2229.12\" width=\"85\" left=\"364.8\" height=\"22\" converted-from=\"Mathcad14\" region-id=\"67\"><math><ml:eval><ml:id xml:space=\"preserve\"><Span xmlns=\"http://schemas.microsoft.com/winfx/2006/xaml/presentation\" xmlns:pw=\"clr-namespace:Ptc.Wpf;assembly=Ptc.Core\">W<pw:Subscript>SedBay</pw:Subscript></Span></ml:id><ml:result /></ml:eval></math></region><region top=\"2277.12\" width=\"174\" left=\"48\" height=\"30\" converted-from=\"Mathcad14\" region-id=\"68\"><math resultRef=\"-4\"><ml:eval><ml:id xml:space=\"preserve\"><Span xmlns=\"http://schemas.microsoft.com/winfx/2006/xaml/presentation\" xmlns:pw=\"clr-namespace:Ptc.Wpf;assembly=Ptc.Core\">Ti<pw:Subscript>ChlorineStock</pw:Subscript></Span></ml:id><ml:result /></ml:eval></math></region><region top=\"2277.12\" width=\"140\" left=\"374.4\" height=\"22\" converted-from=\"Mathcad14\" region-id=\"69\"><math resultRef=\"-5\"><ml:eval><ml:id xml:space=\"preserve\"><Span xmlns=\"http://schemas.microsoft.com/winfx/2006/xaml/presentation\" xmlns:pw=\"clr-namespace:Ptc.Wpf;assembly=Ptc.Core\">HL<pw:Subscript>ChannelMax</pw:Subscript></Span></ml:id><ml:result /></ml:eval></math></region><region top=\"2277.12\" width=\"106\" left=\"576\" height=\"48\" converted-from=\"Mathcad14\" region-id=\"70\"><text><FlowDocument FontFamily=\"Tahoma\" FontStyle=\"Normal\" FontWeight=\"Normal\" FontSize=\"14.6666666666667\" Foreground=\"#FF000000\" Background=\"#00FFFFFF\" PagePadding=\"5,0,5,0\" AllowDrop=\"True\" Typography.Variants=\"Normal\" xmlns=\"http://schemas.microsoft.com/winfx/2006/xaml/presentation\"><Paragraph TextAlignment=\"Left\"><Run FontFamily=\"Arial\" FontStyle=\"Normal\" FontWeight=\"Normal\" FontSize=\"13.3333333333333\" Typography.Variants=\"Normal\"><Run.TextDecorations><TextDecorationCollection /></Run.TextDecorations>Eliminate FCM variable from design specs</Run></Paragraph></FlowDocument></text></region><region top=\"2325.12\" width=\"142\" left=\"48\" height=\"22\" converted-from=\"Mathcad14\" region-id=\"71\"><math resultRef=\"-6\"><ml:eval><ml:id xml:space=\"preserve\"><Span xmlns=\"http://schemas.microsoft.com/winfx/2006/xaml/presentation\" xmlns:pw=\"clr-namespace:Ptc.Wpf;assembly=Ptc.Core\">H<pw:Subscript>PlantFreeboard</pw:Subscript></Span></ml:id><ml:result /></ml:eval></math></region><region top=\"2325.12\" width=\"102\" left=\"364.8\" height=\"22\" converted-from=\"Mathcad14\" region-id=\"72\"><math><ml:eval><ml:id xml:space=\"preserve\"><Span xmlns=\"http://schemas.microsoft.com/winfx/2006/xaml/presentation\" xmlns:pw=\"clr-namespace:Ptc.Wpf;assembly=Ptc.Core\">EN<pw:Subscript>DrillSeries</pw:Subscript></Span></ml:id><ml:result /></ml:eval></math></region><region top=\"2386.32\" width=\"832\" left=\"0\" height=\"19.2\" region-id=\"73\"><text is-text-block=\"true\"><FlowDocument FontFamily=\"Mathcad UniMath\" xmlns=\"http://schemas.microsoft.com/winfx/2006/xaml/presentation\"><Paragraph xml:space=\"preserve\">---↑  ---</Paragraph></FlowDocument></text></region><region top=\"2495.76\" width=\"301\" left=\"9.6\" height=\"19\" converted-from=\"Mathcad14\" region-id=\"74\"><text><FlowDocument FontFamily=\"Tahoma\" FontStyle=\"Normal\" FontWeight=\"Normal\" FontSize=\"14.6666666666667\" Foreground=\"#FF000000\" Background=\"#00FFFFFF\" PagePadding=\"5,0,5,0\" AllowDrop=\"True\" Typography.Variants=\"Normal\" xmlns=\"http://schemas.microsoft.com/winfx/2006/xaml/presentation\"><Paragraph TextAlignment=\"Left\"><Run FontFamily=\"Arial\" FontStyle=\"Normal\" FontWeight=\"Bold\" FontSize=\"16\" Foreground=\"#FF008000\" Typography.Variants=\"Normal\"><Run.TextDecorations><TextDecorationCollection /></Run.TextDecorations>Entrance Tank</Run></Paragraph></FlowDocument></text></region><region top=\"2505.35986\" width=\"832\" left=\"0\" height=\"19.2\" region-id=\"75\"><text is-text-block=\"true\"><FlowDocument FontFamily=\"Mathcad UniMath\" xmlns=\"http://schemas.microsoft.com/winfx/2006/xaml/presentation\"><Paragraph xml:space=\"preserve\">---↓  ---</Paragraph></FlowDocument></text><mc14-conversion-loss-annotations><annotation>CollapsedArea</annotation></mc14-conversion-loss-annotations></region><region top=\"2586\" width=\"124\" left=\"48\" height=\"37\" converted-from=\"Mathcad14\" region-id=\"76\"><math resultRef=\"-7\"><ml:eval><ml:id xml:space=\"preserve\"><Span xmlns=\"http://schemas.microsoft.com/winfx/2006/xaml/presentation\" xmlns:pw=\"clr-namespace:Ptc.Wpf;assembly=Ptc.Core\">V<pw:Subscript>EtUp</pw:Subscript></Span></ml:id><ml:result /></ml:eval></math></region><region top=\"2595.6\" width=\"97\" left=\"364.8\" height=\"22\" converted-from=\"Mathcad14\" region-id=\"77\"><math><ml:eval><ml:id xml:space=\"preserve\"><Span xmlns=\"http://schemas.microsoft.com/winfx/2006/xaml/presentation\" xmlns:pw=\"clr-namespace:Ptc.Wpf;assembly=Ptc.Core\">W<pw:Subscript>EtCapture</pw:Subscript></Span></ml:id><ml:result /></ml:eval></math></region><region top=\"2624.4\" width=\"145\" left=\"547.2\" height=\"22\" converted-from=\"Mathcad14\" region-id=\"78\"><math><ml:eval><ml:id xml:space=\"preserve\"><Span xmlns=\"http://schemas.microsoft.com/winfx/2006/xaml/presentation\" xmlns:pw=\"clr-namespace:Ptc.Wpf;assembly=Ptc.Core\">H<pw:Subscript>EtOverflowChannel</pw:Subscript></Span></ml:id><ml:result /></ml:eval></math></region><region top=\"2634\" width=\"51\" left=\"48\" height=\"22\" converted-from=\"Mathcad14\" region-id=\"79\"><math><ml:eval><ml:id xml:space=\"preserve\"><Span xmlns=\"http://schemas.microsoft.com/winfx/2006/xaml/presentation\" xmlns:pw=\"clr-namespace:Ptc.Wpf;assembly=Ptc.Core\">H<pw:Subscript>Et</pw:Subscript></Span></ml:id><ml:result /></ml:eval></math></region><region top=\"2672.4\" width=\"93\" left=\"57.6\" height=\"22\" converted-from=\"Mathcad14\" region-id=\"80\"><math resultRef=\"-8\"><ml:eval><ml:id xml:space=\"preserve\"><Span xmlns=\"http://schemas.microsoft.com/winfx/2006/xaml/presentation\" xmlns:pw=\"clr-namespace:Ptc.Wpf;assembly=Ptc.Core\">H<pw:Subscript>EtTop</pw:Subscript></Span></ml:id><ml:result /></ml:eval></math></region><region top=\"2672.4\" width=\"378.76\" left=\"192\" height=\"16\" converted-from=\"Mathcad14\" region-id=\"81\"><text><FlowDocument FontFamily=\"Tahoma\" FontStyle=\"Normal\" FontWeight=\"Normal\" FontSize=\"14.6666666666667\" Foreground=\"#FF000000\" Background=\"#00FFFFFF\" PagePadding=\"5,0,5,0\" AllowDrop=\"True\" Typography.Variants=\"Normal\" xmlns=\"http://schemas.microsoft.com/winfx/2006/xaml/presentation\"><Paragraph TextAlignment=\"Left\"><Run FontFamily=\"Arial\" FontStyle=\"Normal\" FontWeight=\"Normal\" FontSize=\"13.3333333333333\" Typography.Variants=\"Normal\"><Run.TextDecorations><TextDecorationCollection /></Run.TextDecorations>height of the top part of the entrance tank above the hoppers</Run></Paragraph></FlowDocument></text></region><region top=\"2710.8\" width=\"55\" left=\"48\" height=\"22\" converted-from=\"Mathcad14\" region-id=\"82\"><math><ml:eval><ml:id xml:space=\"preserve\"><Span xmlns=\"http://schemas.microsoft.com/winfx/2006/xaml/presentation\" xmlns:pw=\"clr-namespace:Ptc.Wpf;assembly=Ptc.Core\">W<pw:Subscript>Et</pw:Subscript></Span></ml:id><ml:result /></ml:eval></math></region><region top=\"2749.2\" width=\"49\" left=\"48\" height=\"22\" converted-from=\"Mathcad14\" region-id=\"83\"><math><ml:eval><ml:id xml:space=\"preserve\"><Span xmlns=\"http://schemas.microsoft.com/winfx/2006/xaml/presentation\" xmlns:pw=\"clr-namespace:Ptc.Wpf;assembly=Ptc.Core\">L<pw:Subscript>Et</pw:Subscript></Span></ml:id><ml:result /></ml:eval></math></region><region top=\"2768.4\" width=\"122\" left=\"480\" height=\"22\" converted-from=\"Mathcad14\" region-id=\"84\"><math resultRef=\"-9\"><ml:eval><ml:id xml:space=\"preserve\"><Span xmlns=\"http://schemas.microsoft.com/winfx/2006/xaml/presentation\" xmlns:pw=\"clr-namespace:Ptc.Wpf;assembly=Ptc.Core\">ND<pw:Subscript>EtDrain</pw:Subscript></Span></ml:id><ml:result /></ml:eval></math></region><region top=\"2768.4\" width=\"94\" left=\"700.8\" height=\"22\" converted-from=\"Mathcad14\" region-id=\"85\"><math resultRef=\"-10\"><ml:eval><ml:id xml:space=\"preserve\"><Span xmlns=\"http://schemas.microsoft.com/winfx/2006/xaml/presentation\" xmlns:pw=\"clr-namespace:Ptc.Wpf;assembly=Ptc.Core\">HL<pw:Subscript>Lfom</pw:Subscript></Span></ml:id><ml:result /></ml:eval></math></region><region top=\"2778\" width=\"63\" left=\"48\" height=\"22\" converted-from=\"Mathcad14\" region-id=\"86\"><math><ml:eval><ml:id xml:space=\"preserve\"><Span xmlns=\"http://schemas.microsoft.com/winfx/2006/xaml/presentation\" xmlns:pw=\"clr-namespace:Ptc.Wpf;assembly=Ptc.Core\">ZW<pw:Subscript>Et</pw:Subscript></Span></ml:id><ml:result /></ml:eval></math></region><region top=\"2806.8\" width=\"72\" left=\"48\" height=\"22\" converted-from=\"Mathcad14\" region-id=\"87\"><math><ml:eval><ml:id xml:space=\"preserve\"><Span xmlns=\"http://schemas.microsoft.com/winfx/2006/xaml/presentation\" xmlns:pw=\"clr-namespace:Ptc.Wpf;assembly=Ptc.Core\">Z<pw:Subscript>EtTop</pw:Subscript></Span></ml:id><ml:result /></ml:eval></math></region><region top=\"2835.6\" width=\"50\" left=\"48\" height=\"22\" converted-from=\"Mathcad14\" region-id=\"88\"><math><ml:eval><ml:id xml:space=\"preserve\"><Span xmlns=\"http://schemas.microsoft.com/winfx/2006/xaml/presentation\" xmlns:pw=\"clr-namespace:Ptc.Wpf;assembly=Ptc.Core\">Z<pw:Subscript>Et</pw:Subscript></Span></ml:id><ml:result /></ml:eval></math></region><region top=\"2835.6\" width=\"154.48\" left=\"201.6\" height=\"16\" converted-from=\"Mathcad14\" region-id=\"89\"><text><FlowDocument FontFamily=\"Tahoma\" FontStyle=\"Normal\" FontWeight=\"Normal\" FontSize=\"14.6666666666667\" Foreground=\"#FF000000\" Background=\"#00FFFFFF\" PagePadding=\"5,0,5,0\" AllowDrop=\"True\" Typography.Variants=\"Normal\" xmlns=\"http://schemas.microsoft.com/winfx/2006/xaml/presentation\"><Paragraph TextAlignment=\"Left\"><Run FontFamily=\"Arial\" FontStyle=\"Normal\" FontWeight=\"Normal\" FontSize=\"13.3333333333333\" Typography.Variants=\"Normal\"><Run.TextDecorations><TextDecorationCollection /></Run.TextDecorations>elevation of top of slab.</Run></Paragraph></FlowDocument></text></region><region top=\"2864.4\" width=\"93\" left=\"480\" height=\"22\" converted-from=\"Mathcad14\" region-id=\"90\"><math><ml:eval><ml:id xml:space=\"preserve\"><Span xmlns=\"http://schemas.microsoft.com/winfx/2006/xaml/presentation\" xmlns:pw=\"clr-namespace:Ptc.Wpf;assembly=Ptc.Core\">ND<pw:Subscript>RMPipe</pw:Subscript></Span></ml:id><ml:result /></ml:eval></math></region><region top=\"2874\" width=\"91\" left=\"57.6\" height=\"22\" converted-from=\"Mathcad14\" region-id=\"91\"><math><ml:eval><ml:id xml:space=\"preserve\"><Span xmlns=\"http://schemas.microsoft.com/winfx/2006/xaml/presentation\" xmlns:pw=\"clr-namespace:Ptc.Wpf;assembly=Ptc.Core\">Z<pw:Subscript>EtHopper</pw:Subscript></Span></ml:id><ml:result /></ml:eval></math></region><region top=\"2912.4\" width=\"92\" left=\"480\" height=\"22\" converted-from=\"Mathcad14\" region-id=\"92\"><math><ml:eval><ml:id xml:space=\"preserve\"><Span xmlns=\"http://schemas.microsoft.com/winfx/2006/xaml/presentation\" xmlns:pw=\"clr-namespace:Ptc.Wpf;assembly=Ptc.Core\">H<pw:Subscript>EtHopper</pw:Subscript></Span></ml:id><ml:result /></ml:eval></math></region><region top=\"2922\" width=\"98\" left=\"57.6\" height=\"22\" converted-from=\"Mathcad14\" region-id=\"93\"><math><ml:eval><ml:id xml:space=\"preserve\"><Span xmlns=\"http://schemas.microsoft.com/winfx/2006/xaml/presentation\" xmlns:pw=\"clr-namespace:Ptc.Wpf;assembly=Ptc.Core\">N<pw:Subscript>EtHoppers</pw:Subscript></Span></ml:id><ml:result /></ml:eval></math></region><region top=\"2950.8\" width=\"128\" left=\"720\" height=\"22\" converted-from=\"Mathcad14\" region-id=\"94\"><math><ml:eval><ml:id xml:space=\"preserve\"><Span xmlns=\"http://schemas.microsoft.com/winfx/2006/xaml/presentation\" xmlns:pw=\"clr-namespace:Ptc.Wpf;assembly=Ptc.Core\">ND<pw:Subscript>EtFlowControl</pw:Subscript></Span></ml:id><ml:result /></ml:eval></math></region><region top=\"2960.4\" width=\"90\" left=\"480\" height=\"22\" converted-from=\"Mathcad14\" region-id=\"95\"><math><ml:eval><ml:id xml:space=\"preserve\"><Span xmlns=\"http://schemas.microsoft.com/winfx/2006/xaml/presentation\" xmlns:pw=\"clr-namespace:Ptc.Wpf;assembly=Ptc.Core\">L<pw:Subscript>EtHopper</pw:Subscript></Span></ml:id><ml:result /></ml:eval></math></region><region top=\"2979.6\" width=\"91\" left=\"57.6\" height=\"22\" converted-from=\"Mathcad14\" region-id=\"96\"><math><ml:eval><ml:id xml:space=\"preserve\"><Span xmlns=\"http://schemas.microsoft.com/winfx/2006/xaml/presentation\" xmlns:pw=\"clr-namespace:Ptc.Wpf;assembly=Ptc.Core\">AN<pw:Subscript>EtSlope</pw:Subscript></Span></ml:id><ml:result /></ml:eval></math></region><region top=\"3027.6\" width=\"72\" left=\"57.6\" height=\"22\" converted-from=\"Mathcad14\" region-id=\"97\"><math><ml:eval><ml:id xml:space=\"preserve\"><Span xmlns=\"http://schemas.microsoft.com/winfx/2006/xaml/presentation\" xmlns:pw=\"clr-namespace:Ptc.Wpf;assembly=Ptc.Core\">W<pw:Subscript>EtDC</pw:Subscript></Span></ml:id><ml:result /></ml:eval></math></region><region top=\"3027.6\" width=\"291.28\" left=\"192\" height=\"16\" converted-from=\"Mathcad14\" region-id=\"98\"><text><FlowDocument FontFamily=\"Tahoma\" FontStyle=\"Normal\" FontWeight=\"Normal\" FontSize=\"14.6666666666667\" Foreground=\"#FF000000\" Background=\"#00FFFFFF\" PagePadding=\"5,0,5,0\" AllowDrop=\"True\" Typography.Variants=\"Normal\" xmlns=\"http://schemas.microsoft.com/winfx/2006/xaml/presentation\"><Paragraph TextAlignment=\"Left\"><Run FontFamily=\"Arial\" FontStyle=\"Normal\" FontWeight=\"Normal\" FontSize=\"13.3333333333333\" Typography.Variants=\"Normal\"><Run.TextDecorations><TextDecorationCollection /></Run.TextDecorations>drain channel under entrance tank dimensions</Run></Paragraph></FlowDocument></text></region><region top=\"3056.4\" width=\"66\" left=\"57.6\" height=\"22\" converted-from=\"Mathcad14\" region-id=\"99\"><math><ml:eval><ml:id xml:space=\"preserve\"><Span xmlns=\"http://schemas.microsoft.com/winfx/2006/xaml/presentation\" xmlns:pw=\"clr-namespace:Ptc.Wpf;assembly=Ptc.Core\">L<pw:Subscript>EtDC</pw:Subscript></Span></ml:id><ml:result /></ml:eval></math></region><region top=\"3094.8\" width=\"327\" left=\"307.2\" height=\"32\" converted-from=\"Mathcad14\" region-id=\"100\"><text><FlowDocument FontFamily=\"Tahoma\" FontStyle=\"Normal\" FontWeight=\"Normal\" FontSize=\"14.6666666666667\" Foreground=\"#FF000000\" Background=\"#00FFFFFF\" PagePadding=\"5,0,5,0\" AllowDrop=\"True\" Typography.Variants=\"Normal\" xmlns=\"http://schemas.microsoft.com/winfx/2006/xaml/presentation\"><Paragraph TextAlignment=\"Left\"><Run FontFamily=\"Arial\" FontStyle=\"Normal\" FontWeight=\"Normal\" FontSize=\"13.3333333333333\" Typography.Variants=\"Normal\"><Run.TextDecorations><TextDecorationCollection /></Run.TextDecorations>Give heights of the channel at the beginning and end and change the design specs to explain that it's sloped.</Run></Paragraph></FlowDocument></text></region><region top=\"3104.4\" width=\"68\" left=\"57.6\" height=\"22\" converted-from=\"Mathcad14\" region-id=\"101\"><math><ml:eval><ml:id xml:space=\"preserve\"><Span xmlns=\"http://schemas.microsoft.com/winfx/2006/xaml/presentation\" xmlns:pw=\"clr-namespace:Ptc.Wpf;assembly=Ptc.Core\">H<pw:Subscript>EtDC</pw:Subscript></Span></ml:id><ml:result /></ml:eval></math></region><region top=\"3152.4\" width=\"129.4\" left=\"9.6\" height=\"16\" converted-from=\"Mathcad14\" region-id=\"102\"><text><FlowDocument FontFamily=\"Tahoma\" FontStyle=\"Normal\" FontWeight=\"Normal\" FontSize=\"14.6666666666667\" Foreground=\"#FF000000\" Background=\"#00FFFFFF\" PagePadding=\"5,0,5,0\" AllowDrop=\"True\" Typography.Variants=\"Normal\" xmlns=\"http://schemas.microsoft.com/winfx/2006/xaml/presentation\"><Paragraph TextAlignment=\"Left\"><Run FontFamily=\"Arial\" FontStyle=\"Normal\" FontWeight=\"Normal\" FontSize=\"13.3333333333333\" Typography.Variants=\"Normal\"><Run.TextDecorations><TextDecorationCollection /></Run.TextDecorations>Flow measurement</Run></Paragraph></FlowDocument></text></region><region top=\"3200.4\" width=\"108\" left=\"38.4\" height=\"22\" converted-from=\"Mathcad14\" region-id=\"103\"><math><ml:eval><ml:id xml:space=\"preserve\"><Span xmlns=\"http://schemas.microsoft.com/winfx/2006/xaml/presentation\" xmlns:pw=\"clr-namespace:Ptc.Wpf;assembly=Ptc.Core\">D<pw:Subscript>LfomOrifices</pw:Subscript></Span></ml:id><ml:result /></ml:eval></math></region><region top=\"3248.4\" width=\"121\" left=\"38.4\" height=\"22\" converted-from=\"Mathcad14\" region-id=\"104\"><math resultRef=\"-11\"><ml:eval><ml:id xml:space=\"preserve\"><Span xmlns=\"http://schemas.microsoft.com/winfx/2006/xaml/presentation\" xmlns:pw=\"clr-namespace:Ptc.Wpf;assembly=Ptc.Core\">S<pw:Subscript>LfomRows</pw:Subscript></Span></ml:id><ml:result /></ml:eval></math></region><region top=\"3421.2\" width=\"102\" left=\"336\" height=\"22\" converted-from=\"Mathcad14\" region-id=\"105\"><math><ml:eval><ml:id xml:space=\"preserve\"><Span xmlns=\"http://schemas.microsoft.com/winfx/2006/xaml/presentation\" xmlns:pw=\"clr-namespace:Ptc.Wpf;assembly=Ptc.Core\">H<pw:Subscript>LfomOrifice</pw:Subscript></Span></ml:id><ml:result /></ml:eval><resultFormat><table /></resultFormat></math></region><region top=\"3421.2\" width=\"95\" left=\"604.8\" height=\"22\" converted-from=\"Mathcad14\" region-id=\"106\"><math><ml:eval><ml:id xml:space=\"preserve\"><Span xmlns=\"http://schemas.microsoft.com/winfx/2006/xaml/presentation\" xmlns:pw=\"clr-namespace:Ptc.Wpf;assembly=Ptc.Core\">Q<pw:Subscript>LfomScale</pw:Subscript></Span></ml:id><ml:result /></ml:eval><resultFormat><table /></resultFormat></math></region><region top=\"3430.8\" width=\"109\" left=\"48\" height=\"22\" converted-from=\"Mathcad14\" region-id=\"107\"><math><ml:eval><ml:id xml:space=\"preserve\"><Span xmlns=\"http://schemas.microsoft.com/winfx/2006/xaml/presentation\" xmlns:pw=\"clr-namespace:Ptc.Wpf;assembly=Ptc.Core\">N<pw:Subscript>LfomOrifices</pw:Subscript></Span></ml:id><ml:result /></ml:eval><resultFormat><table /></resultFormat></math></region><region top=\"3594\" width=\"77\" left=\"28.8\" height=\"22\" converted-from=\"Mathcad14\" region-id=\"108\"><math><ml:eval><ml:id xml:space=\"preserve\"><Span xmlns=\"http://schemas.microsoft.com/winfx/2006/xaml/presentation\" xmlns:pw=\"clr-namespace:Ptc.Wpf;assembly=Ptc.Core\">ND<pw:Subscript>Lfom</pw:Subscript></Span></ml:id><ml:result /></ml:eval></math></region><region top=\"3622.8\" width=\"94\" left=\"403.2\" height=\"22\" converted-from=\"Mathcad14\" region-id=\"109\"><math resultRef=\"-12\"><ml:eval><ml:id xml:space=\"preserve\"><Span xmlns=\"http://schemas.microsoft.com/winfx/2006/xaml/presentation\" xmlns:pw=\"clr-namespace:Ptc.Wpf;assembly=Ptc.Core\">HL<pw:Subscript>Lfom</pw:Subscript></Span></ml:id><ml:result /></ml:eval></math></region><region top=\"3651.6\" width=\"75.92\" left=\"28.8\" height=\"16\" converted-from=\"Mathcad14\" region-id=\"110\"><text><FlowDocument FontFamily=\"Tahoma\" FontStyle=\"Normal\" FontWeight=\"Normal\" FontSize=\"14.6666666666667\" Foreground=\"#FF000000\" Background=\"#00FFFFFF\" PagePadding=\"5,0,5,0\" AllowDrop=\"True\" Typography.Variants=\"Normal\" xmlns=\"http://schemas.microsoft.com/winfx/2006/xaml/presentation\"><Paragraph TextAlignment=\"Left\"><Run FontFamily=\"Arial\" FontStyle=\"Normal\" FontWeight=\"Normal\" FontSize=\"13.3333333333333\" Typography.Variants=\"Normal\"><Run.TextDecorations><TextDecorationCollection /></Run.TextDecorations>Rapid Mix</Run></Paragraph></FlowDocument></text></region><region top=\"3709.2\" width=\"68\" left=\"38.4\" height=\"22\" converted-from=\"Mathcad14\" region-id=\"111\"><math><ml:eval><ml:id xml:space=\"preserve\"><Span xmlns=\"http://schemas.microsoft.com/winfx/2006/xaml/presentation\" xmlns:pw=\"clr-namespace:Ptc.Wpf;assembly=Ptc.Core\">ED<pw:Subscript>Tee</pw:Subscript></Span></ml:id><ml:result /></ml:eval></math></region><region top=\"3795.6\" width=\"162.4\" left=\"201.6\" height=\"16\" converted-from=\"Mathcad14\" region-id=\"112\"><text><FlowDocument FontFamily=\"Tahoma\" FontStyle=\"Normal\" FontWeight=\"Normal\" FontSize=\"14.6666666666667\" Foreground=\"#FF000000\" Background=\"#00FFFFFF\" PagePadding=\"5,0,5,0\" AllowDrop=\"True\" Typography.Variants=\"Normal\" xmlns=\"http://schemas.microsoft.com/winfx/2006/xaml/presentation\"><Paragraph TextAlignment=\"Left\"><Run FontFamily=\"Arial\" FontStyle=\"Normal\" FontWeight=\"Normal\" FontSize=\"13.3333333333333\" Typography.Variants=\"Normal\" xml:space=\"preserve\"><Run.TextDecorations><TextDecorationCollection /></Run.TextDecorations>elevation of the center of </Run></Paragraph></FlowDocument></text></region><region top=\"3805.2\" width=\"107\" left=\"9.6\" height=\"22\" converted-from=\"Mathcad14\" region-id=\"113\"><math><ml:eval><ml:id xml:space=\"preserve\"><Span xmlns=\"http://schemas.microsoft.com/winfx/2006/xaml/presentation\" xmlns:pw=\"clr-namespace:Ptc.Wpf;assembly=Ptc.Core\">Z<pw:Subscript>LfomOrifices</pw:Subscript></Span></ml:id><ml:result /></ml:eval></math></region><region top=\"3834\" width=\"69\" left=\"9.6\" height=\"22\" converted-from=\"Mathcad14\" region-id=\"114\"><math><ml:eval><ml:id xml:space=\"preserve\"><Span xmlns=\"http://schemas.microsoft.com/winfx/2006/xaml/presentation\" xmlns:pw=\"clr-namespace:Ptc.Wpf;assembly=Ptc.Core\">Z<pw:Subscript>EtExit</pw:Subscript></Span></ml:id><ml:result /></ml:eval></math></region><region top=\"3834\" width=\"527.52\" left=\"201.6\" height=\"32\" converted-from=\"Mathcad14\" region-id=\"115\"><text><FlowDocument FontFamily=\"Tahoma\" FontStyle=\"Normal\" FontWeight=\"Normal\" FontSize=\"14.6666666666667\" Foreground=\"#FF000000\" Background=\"#00FFFFFF\" PagePadding=\"5,0,5,0\" AllowDrop=\"True\" Typography.Variants=\"Normal\" xmlns=\"http://schemas.microsoft.com/winfx/2006/xaml/presentation\"><Paragraph TextAlignment=\"Left\"><Run FontFamily=\"Arial\" FontStyle=\"Normal\" FontWeight=\"Normal\" FontSize=\"13.3333333333333\" Typography.Variants=\"Normal\"><Run.TextDecorations><TextDecorationCollection /></Run.TextDecorations>elevation of center of pipe exiting the entrance tank and heading toward the flocculator</Run></Paragraph></FlowDocument></text></region><region top=\"3914.4\" width=\"832\" left=\"0\" height=\"19.2\" region-id=\"116\"><text is-text-block=\"true\"><FlowDocument FontFamily=\"Mathcad UniMath\" xmlns=\"http://schemas.microsoft.com/winfx/2006/xaml/presentation\"><Paragraph xml:space=\"preserve\">---↑  ---</Paragraph></FlowDocument></text></region><region top=\"4043.03979\" width=\"832\" left=\"0\" height=\"19.2\" region-id=\"117\"><text is-text-block=\"true\"><FlowDocument FontFamily=\"Mathcad UniMath\" xmlns=\"http://schemas.microsoft.com/winfx/2006/xaml/presentation\"><Paragraph xml:space=\"preserve\">---↓  ---</Paragraph></FlowDocument></text><mc14-conversion-loss-annotations><annotation>CollapsedArea</annotation></mc14-conversion-loss-annotations></region><region top=\"4114.07959\" width=\"72\" left=\"28.8\" height=\"22\" converted-from=\"Mathcad14\" region-id=\"118\"><math resultRef=\"-13\"><ml:eval><ml:id xml:space=\"preserve\"><Span xmlns=\"http://schemas.microsoft.com/winfx/2006/xaml/presentation\" xmlns:pw=\"clr-namespace:Ptc.Wpf;assembly=Ptc.Core\">W<pw:Subscript>DC</pw:Subscript></Span></ml:id><ml:result /></ml:eval></math></region><region top=\"4133.28\" width=\"398\" left=\"201.6\" height=\"48\" converted-from=\"Mathcad14\" region-id=\"119\"><text><FlowDocument FontFamily=\"Tahoma\" FontStyle=\"Normal\" FontWeight=\"Normal\" FontSize=\"14.6666666666667\" Foreground=\"#FF000000\" Background=\"#00FFFFFF\" PagePadding=\"5,0,5,0\" AllowDrop=\"True\" Typography.Variants=\"Normal\" xmlns=\"http://schemas.microsoft.com/winfx/2006/xaml/presentation\"><Paragraph TextAlignment=\"Left\"><Run FontFamily=\"Arial\" FontStyle=\"Normal\" FontWeight=\"Normal\" FontSize=\"13.3333333333333\" Typography.Variants=\"Normal\"><Run.TextDecorations><TextDecorationCollection /></Run.TextDecorations>Maybe give the vertical distances below the bottom of the sed tank of the beginning and end of the channel? Calculate them, display, and add to the design specs.</Run></Paragraph></FlowDocument></text></region><region top=\"4152.47949\" width=\"57\" left=\"28.8\" height=\"22\" converted-from=\"Mathcad14\" region-id=\"120\"><math><ml:eval><ml:id xml:space=\"preserve\"><Span xmlns=\"http://schemas.microsoft.com/winfx/2006/xaml/presentation\" xmlns:pw=\"clr-namespace:Ptc.Wpf;assembly=Ptc.Core\">H<pw:Subscript>DC</pw:Subscript></Span></ml:id><ml:result /></ml:eval></math></region><region top=\"4190.88\" width=\"55\" left=\"28.8\" height=\"22\" converted-from=\"Mathcad14\" region-id=\"121\"><math><ml:eval><ml:id xml:space=\"preserve\"><Span xmlns=\"http://schemas.microsoft.com/winfx/2006/xaml/presentation\" xmlns:pw=\"clr-namespace:Ptc.Wpf;assembly=Ptc.Core\">L<pw:Subscript>DC</pw:Subscript></Span></ml:id><ml:result /></ml:eval></math></region><region top=\"4252.07959\" width=\"832\" left=\"0\" height=\"19.2\" region-id=\"122\"><text is-text-block=\"true\"><FlowDocument FontFamily=\"Mathcad UniMath\" xmlns=\"http://schemas.microsoft.com/winfx/2006/xaml/presentation\"><Paragraph xml:space=\"preserve\">---↑  ---</Paragraph></FlowDocument></text></region><region top=\"4275.12\" width=\"310\" left=\"9.6\" height=\"19\" converted-from=\"Mathcad14\" region-id=\"123\"><text><FlowDocument FontFamily=\"Tahoma\" FontStyle=\"Normal\" FontWeight=\"Normal\" FontSize=\"14.6666666666667\" Foreground=\"#FF000000\" Background=\"#00FFFFFF\" PagePadding=\"5,0,5,0\" AllowDrop=\"True\" Typography.Variants=\"Normal\" xmlns=\"http://schemas.microsoft.com/winfx/2006/xaml/presentation\"><Paragraph TextAlignment=\"Left\"><Run FontFamily=\"Arial\" FontStyle=\"Normal\" FontWeight=\"Bold\" FontSize=\"16\" Foreground=\"#FF008000\" Typography.Variants=\"Normal\"><Run.TextDecorations><TextDecorationCollection /></Run.TextDecorations>Plant Drain Channel</Run></Paragraph></FlowDocument></text></region><region top=\"4371.12\" width=\"832\" left=\"0\" height=\"19.2\" region-id=\"124\"><text is-text-block=\"true\"><FlowDocument FontFamily=\"Mathcad UniMath\" xmlns=\"http://schemas.microsoft.com/winfx/2006/xaml/presentation\"><Paragraph xml:space=\"preserve\">---↓  ---</Paragraph></FlowDocument></text><mc14-conversion-loss-annotations><annotation>CollapsedArea</annotation></mc14-conversion-loss-annotations></region><region top=\"4432.55957\" width=\"95\" left=\"28.8\" height=\"22\" converted-from=\"Mathcad14\" region-id=\"125\"><math><ml:eval><ml:id xml:space=\"preserve\"><Span xmlns=\"http://schemas.microsoft.com/winfx/2006/xaml/presentation\" xmlns:pw=\"clr-namespace:Ptc.Wpf;assembly=Ptc.Core\">Z<pw:Subscript>CoagTank</pw:Subscript></Span></ml:id><ml:result /></ml:eval></math></region><region top=\"4480.55957\" width=\"127\" left=\"28.8\" height=\"22\" converted-from=\"Mathcad14\" region-id=\"126\"><math><ml:eval><ml:id xml:space=\"preserve\"><Span xmlns=\"http://schemas.microsoft.com/winfx/2006/xaml/presentation\" xmlns:pw=\"clr-namespace:Ptc.Wpf;assembly=Ptc.Core\">Z<pw:Subscript>CoagTankOutlet</pw:Subscript></Span></ml:id><ml:result /></ml:eval></math></region><region top=\"4528.55957\" width=\"141\" left=\"28.8\" height=\"22\" converted-from=\"Mathcad14\" region-id=\"127\"><math resultRef=\"-14\"><ml:eval><ml:id xml:space=\"preserve\"><Span xmlns=\"http://schemas.microsoft.com/winfx/2006/xaml/presentation\" xmlns:pw=\"clr-namespace:Ptc.Wpf;assembly=Ptc.Core\">L<pw:Subscript>CdcFloatArm</pw:Subscript></Span></ml:id><ml:result /></ml:eval></math></region><region top=\"4547.76\" width=\"84\" left=\"316.8\" height=\"22\" converted-from=\"Mathcad14\" region-id=\"128\"><math><ml:eval><ml:id xml:space=\"preserve\"><Span xmlns=\"http://schemas.microsoft.com/winfx/2006/xaml/presentation\" xmlns:pw=\"clr-namespace:Ptc.Wpf;assembly=Ptc.Core\">Q<pw:Subscript>CdcMax</pw:Subscript></Span></ml:id><ml:result /></ml:eval></math></region><region top=\"4576.55957\" width=\"142\" left=\"28.8\" height=\"22\" converted-from=\"Mathcad14\" region-id=\"129\"><math resultRef=\"-15\"><ml:eval><ml:id xml:space=\"preserve\"><Span xmlns=\"http://schemas.microsoft.com/winfx/2006/xaml/presentation\" xmlns:pw=\"clr-namespace:Ptc.Wpf;assembly=Ptc.Core\">L<pw:Subscript>CdcScaleArm</pw:Subscript></Span></ml:id><ml:result /></ml:eval></math></region><region top=\"4595.76\" width=\"154\" left=\"614.4\" height=\"45\" converted-from=\"Mathcad14\" region-id=\"130\"><math resultRef=\"-16\"><ml:eval><ml:id xml:space=\"preserve\"><Span xmlns=\"http://schemas.microsoft.com/winfx/2006/xaml/presentation\" xmlns:pw=\"clr-namespace:Ptc.Wpf;assembly=Ptc.Core\">C<pw:Subscript>CoagDoseMax</pw:Subscript></Span></ml:id><ml:result /></ml:eval></math></region><region top=\"4624.55957\" width=\"122\" left=\"28.8\" height=\"22\" converted-from=\"Mathcad14\" region-id=\"131\"><math resultRef=\"-17\"><ml:eval><ml:id xml:space=\"preserve\"><Span xmlns=\"http://schemas.microsoft.com/winfx/2006/xaml/presentation\" xmlns:pw=\"clr-namespace:Ptc.Wpf;assembly=Ptc.Core\">B<pw:Subscript>StockOutlet</pw:Subscript></Span></ml:id><ml:result /></ml:eval></math></region><region top=\"4701.36\" width=\"115\" left=\"316.8\" height=\"22\" converted-from=\"Mathcad14\" region-id=\"132\"><math><ml:eval><ml:id xml:space=\"preserve\"><Span xmlns=\"http://schemas.microsoft.com/winfx/2006/xaml/presentation\" xmlns:pw=\"clr-namespace:Ptc.Wpf;assembly=Ptc.Core\">L<pw:Subscript>CoagCdcTube</pw:Subscript></Span></ml:id><ml:result /></ml:eval></math></region><region top=\"4720.55957\" width=\"164\" left=\"28.8\" height=\"30\" converted-from=\"Mathcad14\" region-id=\"133\"><math resultRef=\"-18\"><ml:eval><ml:id xml:space=\"preserve\"><Span xmlns=\"http://schemas.microsoft.com/winfx/2006/xaml/presentation\" xmlns:pw=\"clr-namespace:Ptc.Wpf;assembly=Ptc.Core\">D<pw:Subscript>CdcTube</pw:Subscript></Span></ml:id><ml:result /></ml:eval></math></region><region top=\"4758.96\" width=\"124\" left=\"28.8\" height=\"22\" converted-from=\"Mathcad14\" region-id=\"134\"><math><ml:eval><ml:id xml:space=\"preserve\"><Span xmlns=\"http://schemas.microsoft.com/winfx/2006/xaml/presentation\" xmlns:pw=\"clr-namespace:Ptc.Wpf;assembly=Ptc.Core\">N<pw:Subscript>CoagCdcTubes</pw:Subscript></Span></ml:id><ml:result /></ml:eval></math></region><region top=\"4797.36\" width=\"88\" left=\"374.4\" height=\"22\" converted-from=\"Mathcad14\" region-id=\"135\"><math resultRef=\"-19\"><ml:eval><ml:id xml:space=\"preserve\"><Span xmlns=\"http://schemas.microsoft.com/winfx/2006/xaml/presentation\" xmlns:pw=\"clr-namespace:Ptc.Wpf;assembly=Ptc.Core\">HL<pw:Subscript>Cdc</pw:Subscript></Span></ml:id><ml:result /></ml:eval></math></region><region top=\"4806.96\" width=\"141\" left=\"28.8\" height=\"22\" converted-from=\"Mathcad14\" region-id=\"136\"><math resultRef=\"-20\"><ml:eval><ml:id xml:space=\"preserve\"><Span xmlns=\"http://schemas.microsoft.com/winfx/2006/xaml/presentation\" xmlns:pw=\"clr-namespace:Ptc.Wpf;assembly=Ptc.Core\">L<pw:Subscript>CdcFloatArm</pw:Subscript></Span></ml:id><ml:result /></ml:eval></math></region><region top=\"4845.36\" width=\"142\" left=\"28.8\" height=\"22\" converted-from=\"Mathcad14\" region-id=\"137\"><math resultRef=\"-21\"><ml:eval><ml:id xml:space=\"preserve\"><Span xmlns=\"http://schemas.microsoft.com/winfx/2006/xaml/presentation\" xmlns:pw=\"clr-namespace:Ptc.Wpf;assembly=Ptc.Core\">L<pw:Subscript>CdcScaleArm</pw:Subscript></Span></ml:id><ml:result /></ml:eval></math></region><region top=\"4973.76\" width=\"832\" left=\"0\" height=\"19.2\" region-id=\"138\"><text is-text-block=\"true\"><FlowDocument FontFamily=\"Mathcad UniMath\" xmlns=\"http://schemas.microsoft.com/winfx/2006/xaml/presentation\"><Paragraph xml:space=\"preserve\">---↑  ---</Paragraph></FlowDocument></text></region><region top=\"4996.8\" width=\"310\" left=\"9.6\" height=\"19\" converted-from=\"Mathcad14\" region-id=\"139\"><text><FlowDocument FontFamily=\"Tahoma\" FontStyle=\"Normal\" FontWeight=\"Normal\" FontSize=\"14.6666666666667\" Foreground=\"#FF000000\" Background=\"#00FFFFFF\" PagePadding=\"5,0,5,0\" AllowDrop=\"True\" Typography.Variants=\"Normal\" xmlns=\"http://schemas.microsoft.com/winfx/2006/xaml/presentation\"><Paragraph Margin=\"0,0,0,0\" TextAlignment=\"Left\"><Run FontFamily=\"Arial\" FontStyle=\"Normal\" FontWeight=\"Bold\" FontSize=\"16\" Foreground=\"#FF008000\" Typography.Variants=\"Normal\"><Run.TextDecorations><TextDecorationCollection /></Run.TextDecorations>Coag Dose Controller</Run></Paragraph></FlowDocument></text></region><region top=\"5092.8\" width=\"103.36\" left=\"9.6\" height=\"19\" converted-from=\"Mathcad14\" region-id=\"140\"><text><FlowDocument FontFamily=\"Tahoma\" FontStyle=\"Normal\" FontWeight=\"Normal\" FontSize=\"14.6666666666667\" Foreground=\"#FF000000\" Background=\"#00FFFFFF\" PagePadding=\"5,0,5,0\" AllowDrop=\"True\" Typography.Variants=\"Normal\" xmlns=\"http://schemas.microsoft.com/winfx/2006/xaml/presentation\"><Paragraph TextAlignment=\"Left\"><Run FontFamily=\"Arial\" FontStyle=\"Normal\" FontWeight=\"Bold\" FontSize=\"16\" Foreground=\"#FF008000\" Typography.Variants=\"Normal\"><Run.TextDecorations><TextDecorationCollection /></Run.TextDecorations>Flocculator</Run></Paragraph></FlowDocument></text></region><region top=\"5102.4\" width=\"832\" left=\"0\" height=\"19.2\" region-id=\"141\"><text is-text-block=\"true\"><FlowDocument FontFamily=\"Mathcad UniMath\" xmlns=\"http://schemas.microsoft.com/winfx/2006/xaml/presentation\"><Paragraph xml:space=\"preserve\">---↓  ---</Paragraph></FlowDocument></text><mc14-conversion-loss-annotations><annotation>CollapsedArea</annotation></mc14-conversion-loss-annotations></region><region top=\"5163.84\" width=\"240.52\" left=\"681.6\" height=\"16\" converted-from=\"Mathcad14\" region-id=\"142\"><text><FlowDocument FontFamily=\"Tahoma\" FontStyle=\"Normal\" FontWeight=\"Normal\" FontSize=\"14.6666666666667\" Foreground=\"#FF000000\" Background=\"#00FFFFFF\" PagePadding=\"5,0,5,0\" AllowDrop=\"True\" Typography.Variants=\"Normal\" xmlns=\"http://schemas.microsoft.com/winfx/2006/xaml/presentation\"><Paragraph TextAlignment=\"Left\"><Run FontFamily=\"Arial\" FontStyle=\"Normal\" FontWeight=\"Normal\" FontSize=\"13.3333333333333\" Typography.Variants=\"Normal\"><Run.TextDecorations><TextDecorationCollection /></Run.TextDecorations>Look at Flocculator Positioning arrays</Run></Paragraph></FlowDocument></text></region><region top=\"5173.44\" width=\"63\" left=\"19.2\" height=\"22\" converted-from=\"Mathcad14\" region-id=\"143\"><math><ml:eval><ml:id xml:space=\"preserve\"><Span xmlns=\"http://schemas.microsoft.com/winfx/2006/xaml/presentation\" xmlns:pw=\"clr-namespace:Ptc.Wpf;assembly=Ptc.Core\">H<pw:Subscript>Floc</pw:Subscript></Span></ml:id><ml:result /></ml:eval></math></region><region top=\"5173.44\" width=\"90\" left=\"230.4\" height=\"22\" converted-from=\"Mathcad14\" region-id=\"144\"><math><ml:eval><ml:id xml:space=\"preserve\"><Span xmlns=\"http://schemas.microsoft.com/winfx/2006/xaml/presentation\" xmlns:pw=\"clr-namespace:Ptc.Wpf;assembly=Ptc.Core\">Z<pw:Subscript>FlocTank</pw:Subscript></Span></ml:id><ml:result /></ml:eval></math></region><region top=\"5202.23975\" width=\"100\" left=\"432\" height=\"22\" converted-from=\"Mathcad14\" region-id=\"145\"><math><ml:eval><ml:id xml:space=\"preserve\"><Span xmlns=\"http://schemas.microsoft.com/winfx/2006/xaml/presentation\" xmlns:pw=\"clr-namespace:Ptc.Wpf;assembly=Ptc.Core\">N<pw:Subscript>FlocValves</pw:Subscript></Span></ml:id><ml:result /></ml:eval></math></region><region top=\"5221.44\" width=\"112\" left=\"19.2\" height=\"22\" converted-from=\"Mathcad14\" region-id=\"146\"><math><ml:eval><ml:id xml:space=\"preserve\"><Span xmlns=\"http://schemas.microsoft.com/winfx/2006/xaml/presentation\" xmlns:pw=\"clr-namespace:Ptc.Wpf;assembly=Ptc.Core\">W<pw:Subscript>FlocChannel</pw:Subscript></Span></ml:id><ml:result /></ml:eval></math></region><region top=\"5221.44\" width=\"290.2\" left=\"748.8\" height=\"16\" converted-from=\"Mathcad14\" region-id=\"147\"><text><FlowDocument FontFamily=\"Tahoma\" FontStyle=\"Normal\" FontWeight=\"Normal\" FontSize=\"14.6666666666667\" Foreground=\"#FF000000\" Background=\"#00FFFFFF\" PagePadding=\"5,0,5,0\" AllowDrop=\"True\" Typography.Variants=\"Normal\" xmlns=\"http://schemas.microsoft.com/winfx/2006/xaml/presentation\"><Paragraph TextAlignment=\"Left\"><Run FontFamily=\"Arial\" FontStyle=\"Normal\" FontWeight=\"Normal\" FontSize=\"13.3333333333333\" Typography.Variants=\"Normal\"><Run.TextDecorations><TextDecorationCollection /></Run.TextDecorations>Fill last channel with bafffles from last channel</Run></Paragraph></FlowDocument></text></region><region top=\"5231.04\" width=\"65\" left=\"240\" height=\"22\" converted-from=\"Mathcad14\" region-id=\"148\"><math><ml:eval><ml:id xml:space=\"preserve\"><Span xmlns=\"http://schemas.microsoft.com/winfx/2006/xaml/presentation\" xmlns:pw=\"clr-namespace:Ptc.Wpf;assembly=Ptc.Core\">Ti<pw:Subscript>Floc</pw:Subscript></Span></ml:id><ml:result /></ml:eval></math></region><region top=\"5240.63965\" width=\"93\" left=\"441.6\" height=\"22\" converted-from=\"Mathcad14\" region-id=\"149\"><math><ml:eval><ml:id xml:space=\"preserve\"><Span xmlns=\"http://schemas.microsoft.com/winfx/2006/xaml/presentation\" xmlns:pw=\"clr-namespace:Ptc.Wpf;assembly=Ptc.Core\">H<pw:Subscript>FlocSlope</pw:Subscript></Span></ml:id><ml:result /></ml:eval></math></region><region top=\"5240.63965\" width=\"391.96\" left=\"748.8\" height=\"16\" converted-from=\"Mathcad14\" region-id=\"150\"><text><FlowDocument FontFamily=\"Tahoma\" FontStyle=\"Normal\" FontWeight=\"Normal\" FontSize=\"14.6666666666667\" Foreground=\"#FF000000\" Background=\"#00FFFFFF\" PagePadding=\"5,0,5,0\" AllowDrop=\"True\" Typography.Variants=\"Normal\" xmlns=\"http://schemas.microsoft.com/winfx/2006/xaml/presentation\"><Paragraph TextAlignment=\"Left\"><Run FontFamily=\"Arial\" FontStyle=\"Normal\" FontWeight=\"Normal\" FontSize=\"13.3333333333333\" Typography.Variants=\"Normal\"><Run.TextDecorations><TextDecorationCollection /></Run.TextDecorations>Fix port width to be based on energy dissipation in that channel</Run></Paragraph></FlowDocument></text></region><region top=\"5259.84\" width=\"395.14\" left=\"748.8\" height=\"16\" converted-from=\"Mathcad14\" region-id=\"151\"><text><FlowDocument FontFamily=\"Tahoma\" FontStyle=\"Normal\" FontWeight=\"Normal\" FontSize=\"14.6666666666667\" Foreground=\"#FF000000\" Background=\"#00FFFFFF\" PagePadding=\"5,0,5,0\" AllowDrop=\"True\" Typography.Variants=\"Normal\" xmlns=\"http://schemas.microsoft.com/winfx/2006/xaml/presentation\"><Paragraph TextAlignment=\"Left\"><Run FontFamily=\"Arial\" FontStyle=\"Normal\" FontWeight=\"Normal\" FontSize=\"13.3333333333333\" Typography.Variants=\"Normal\"><Run.TextDecorations><TextDecorationCollection /></Run.TextDecorations>Adjust spacing after the number of baffles per channel is known.</Run></Paragraph></FlowDocument></text></region><region top=\"5269.44\" width=\"107\" left=\"19.2\" height=\"53\" converted-from=\"Mathcad14\" region-id=\"152\"><math resultRef=\"-22\"><ml:eval><ml:id xml:space=\"preserve\"><Span xmlns=\"http://schemas.microsoft.com/winfx/2006/xaml/presentation\" xmlns:pw=\"clr-namespace:Ptc.Wpf;assembly=Ptc.Core\">ED<pw:Subscript>Floc</pw:Subscript></Span></ml:id><ml:result /></ml:eval></math></region><region top=\"5279.04\" width=\"62\" left=\"240\" height=\"22\" converted-from=\"Mathcad14\" region-id=\"153\"><math><ml:eval><ml:id xml:space=\"preserve\"><Span xmlns=\"http://schemas.microsoft.com/winfx/2006/xaml/presentation\" xmlns:pw=\"clr-namespace:Ptc.Wpf;assembly=Ptc.Core\">V<pw:Subscript>Floc</pw:Subscript></Span></ml:id><ml:result /></ml:eval></math></region><region top=\"5279.04\" width=\"442.88\" left=\"748.8\" height=\"16\" converted-from=\"Mathcad14\" region-id=\"154\"><text><FlowDocument FontFamily=\"Tahoma\" FontStyle=\"Normal\" FontWeight=\"Normal\" FontSize=\"14.6666666666667\" Foreground=\"#FF000000\" Background=\"#00FFFFFF\" PagePadding=\"5,0,5,0\" AllowDrop=\"True\" Typography.Variants=\"Normal\" xmlns=\"http://schemas.microsoft.com/winfx/2006/xaml/presentation\"><Paragraph TextAlignment=\"Left\"><Run FontFamily=\"Arial\" FontStyle=\"Normal\" FontWeight=\"Normal\" FontSize=\"13.3333333333333\" Typography.Variants=\"Normal\" xml:space=\"preserve\"><Run.TextDecorations><TextDecorationCollection /></Run.TextDecorations>Check the residence time of the flocculator should be at least 20minutes </Run></Paragraph></FlowDocument></text></region><region top=\"5317.44\" width=\"98\" left=\"19.2\" height=\"22\" converted-from=\"Mathcad14\" region-id=\"155\"><math><ml:eval><ml:id xml:space=\"preserve\"><Span xmlns=\"http://schemas.microsoft.com/winfx/2006/xaml/presentation\" xmlns:pw=\"clr-namespace:Ptc.Wpf;assembly=Ptc.Core\">HW<pw:Subscript>FlocEnd</pw:Subscript></Span></ml:id><ml:result /></ml:eval></math></region><region top=\"5336.63965\" width=\"103\" left=\"259.2\" height=\"22\" converted-from=\"Mathcad14\" region-id=\"156\"><math><ml:eval><ml:id xml:space=\"preserve\"><Span xmlns=\"http://schemas.microsoft.com/winfx/2006/xaml/presentation\" xmlns:pw=\"clr-namespace:Ptc.Wpf;assembly=Ptc.Core\">ND<pw:Subscript>FlocValve</pw:Subscript></Span></ml:id><ml:result /></ml:eval></math></region><region top=\"5355.84\" width=\"113\" left=\"28.8\" height=\"30\" converted-from=\"Mathcad14\" region-id=\"157\"><math resultRef=\"-23\"><ml:eval><ml:id xml:space=\"preserve\"><Span xmlns=\"http://schemas.microsoft.com/winfx/2006/xaml/presentation\" xmlns:pw=\"clr-namespace:Ptc.Wpf;assembly=Ptc.Core\">CP<pw:Subscript>Floc</pw:Subscript></Span></ml:id><ml:result /></ml:eval></math></region><region top=\"5384.63965\" width=\"144\" left=\"259.2\" height=\"30\" converted-from=\"Mathcad14\" region-id=\"158\"><math resultRef=\"-24\"><ml:eval><ml:id xml:space=\"preserve\"><Span xmlns=\"http://schemas.microsoft.com/winfx/2006/xaml/presentation\" xmlns:pw=\"clr-namespace:Ptc.Wpf;assembly=Ptc.Core\">Ti<pw:Subscript>FlocDrain</pw:Subscript></Span></ml:id><ml:result /></ml:eval></math></region><region top=\"5403.84\" width=\"98\" left=\"28.8\" height=\"22\" converted-from=\"Mathcad14\" region-id=\"159\"><math><ml:eval><ml:id xml:space=\"preserve\"><Span xmlns=\"http://schemas.microsoft.com/winfx/2006/xaml/presentation\" xmlns:pw=\"clr-namespace:Ptc.Wpf;assembly=Ptc.Core\">CP<pw:Subscript>FlocTotal</pw:Subscript></Span></ml:id><ml:result /></ml:eval></math></region><region top=\"5461.44\" width=\"114\" left=\"19.2\" height=\"22\" converted-from=\"Mathcad14\" region-id=\"160\"><math><ml:eval><ml:id xml:space=\"preserve\"><Span xmlns=\"http://schemas.microsoft.com/winfx/2006/xaml/presentation\" xmlns:pw=\"clr-namespace:Ptc.Wpf;assembly=Ptc.Core\">N<pw:Subscript>FlocChannels</pw:Subscript></Span></ml:id><ml:result /></ml:eval></math></region><region top=\"5461.44\" width=\"62\" left=\"268.8\" height=\"22\" converted-from=\"Mathcad14\" region-id=\"161\"><math><ml:eval><ml:id xml:space=\"preserve\"><Span xmlns=\"http://schemas.microsoft.com/winfx/2006/xaml/presentation\" xmlns:pw=\"clr-namespace:Ptc.Wpf;assembly=Ptc.Core\">G<pw:Subscript>Floc</pw:Subscript></Span></ml:id><ml:result /></ml:eval></math></region><region top=\"5499.84\" width=\"89\" left=\"19.2\" height=\"22\" converted-from=\"Mathcad14\" region-id=\"162\"><math><ml:eval><ml:id xml:space=\"preserve\"><Span xmlns=\"http://schemas.microsoft.com/winfx/2006/xaml/presentation\" xmlns:pw=\"clr-namespace:Ptc.Wpf;assembly=Ptc.Core\">L<pw:Subscript>FlocTank</pw:Subscript></Span></ml:id><ml:result /></ml:eval></math></region><region top=\"5547.84\" width=\"70\" left=\"19.2\" height=\"22\" converted-from=\"Mathcad14\" region-id=\"163\"><math><ml:eval><ml:id xml:space=\"preserve\"><Span xmlns=\"http://schemas.microsoft.com/winfx/2006/xaml/presentation\" xmlns:pw=\"clr-namespace:Ptc.Wpf;assembly=Ptc.Core\">HL<pw:Subscript>Floc</pw:Subscript></Span></ml:id><ml:result /></ml:eval></math></region><region top=\"5547.84\" width=\"139\" left=\"268.8\" height=\"22\" converted-from=\"Mathcad14\" region-id=\"164\"><math><ml:eval><ml:id xml:space=\"preserve\"><Span xmlns=\"http://schemas.microsoft.com/winfx/2006/xaml/presentation\" xmlns:pw=\"clr-namespace:Ptc.Wpf;assembly=Ptc.Core\">ED<pw:Subscript>FlocChannelFirst</pw:Subscript></Span></ml:id><ml:result /></ml:eval></math></region><region top=\"5605.44\" width=\"101\" left=\"19.2\" height=\"22\" converted-from=\"Mathcad14\" region-id=\"165\"><math><ml:eval><ml:id xml:space=\"preserve\"><Span xmlns=\"http://schemas.microsoft.com/winfx/2006/xaml/presentation\" xmlns:pw=\"clr-namespace:Ptc.Wpf;assembly=Ptc.Core\">HW<pw:Subscript>FlocStart</pw:Subscript></Span></ml:id><ml:result /></ml:eval></math></region><region top=\"5720.63965\" width=\"92\" left=\"28.8\" height=\"22\" converted-from=\"Mathcad14\" region-id=\"166\"><math><ml:eval><ml:id xml:space=\"preserve\"><Span xmlns=\"http://schemas.microsoft.com/winfx/2006/xaml/presentation\" xmlns:pw=\"clr-namespace:Ptc.Wpf;assembly=Ptc.Core\">S<pw:Subscript>FlocBaffle</pw:Subscript></Span></ml:id><ml:result /></ml:eval></math></region><region top=\"5720.63965\" width=\"93\" left=\"240\" height=\"22\" converted-from=\"Mathcad14\" region-id=\"167\"><math><ml:eval><ml:id xml:space=\"preserve\"><Span xmlns=\"http://schemas.microsoft.com/winfx/2006/xaml/presentation\" xmlns:pw=\"clr-namespace:Ptc.Wpf;assembly=Ptc.Core\">B<pw:Subscript>FlocBaffle</pw:Subscript></Span></ml:id><ml:result /></ml:eval></math></region><region top=\"5720.63965\" width=\"145\" left=\"470.4\" height=\"22\" converted-from=\"Mathcad14\" region-id=\"168\"><math><ml:eval><ml:id xml:space=\"preserve\"><Span xmlns=\"http://schemas.microsoft.com/winfx/2006/xaml/presentation\" xmlns:pw=\"clr-namespace:Ptc.Wpf;assembly=Ptc.Core\">N<pw:Subscript>FlocChannelBaffles</pw:Subscript></Span></ml:id><ml:result /></ml:eval></math></region><region top=\"5720.63965\" width=\"89\" left=\"720\" height=\"22\" converted-from=\"Mathcad14\" region-id=\"169\"><math><ml:eval><ml:id xml:space=\"preserve\"><Span xmlns=\"http://schemas.microsoft.com/winfx/2006/xaml/presentation\" xmlns:pw=\"clr-namespace:Ptc.Wpf;assembly=Ptc.Core\">W<pw:Subscript>FlocPort</pw:Subscript></Span></ml:id><ml:result /></ml:eval></math></region><region top=\"5797.44\" width=\"116\" left=\"28.8\" height=\"22\" converted-from=\"Mathcad14\" region-id=\"170\"><math><ml:eval><ml:id xml:space=\"preserve\"><Span xmlns=\"http://schemas.microsoft.com/winfx/2006/xaml/presentation\" xmlns:pw=\"clr-namespace:Ptc.Wpf;assembly=Ptc.Core\">S<pw:Subscript>FlocBaffleFirst</pw:Subscript></Span></ml:id><ml:result /></ml:eval></math></region><region top=\"5912.63965\" width=\"120\" left=\"28.8\" height=\"22\" converted-from=\"Mathcad14\" region-id=\"171\"><math><ml:eval><ml:id xml:space=\"preserve\"><Span xmlns=\"http://schemas.microsoft.com/winfx/2006/xaml/presentation\" xmlns:pw=\"clr-namespace:Ptc.Wpf;assembly=Ptc.Core\">HL<pw:Subscript>FlocChannels</pw:Subscript></Span></ml:id><ml:result /></ml:eval></math></region><region top=\"5912.63965\" width=\"126\" left=\"268.8\" height=\"22\" converted-from=\"Mathcad14\" region-id=\"172\"><math><ml:eval><ml:id xml:space=\"preserve\"><Span xmlns=\"http://schemas.microsoft.com/winfx/2006/xaml/presentation\" xmlns:pw=\"clr-namespace:Ptc.Wpf;assembly=Ptc.Core\">L<pw:Subscript>FlocBaffleLower</pw:Subscript></Span></ml:id><ml:result /></ml:eval></math></region><region top=\"5912.63965\" width=\"126\" left=\"508.8\" height=\"22\" converted-from=\"Mathcad14\" region-id=\"173\"><math><ml:eval><ml:id xml:space=\"preserve\"><Span xmlns=\"http://schemas.microsoft.com/winfx/2006/xaml/presentation\" xmlns:pw=\"clr-namespace:Ptc.Wpf;assembly=Ptc.Core\">L<pw:Subscript>FlocBaffleUpper</pw:Subscript></Span></ml:id><ml:result /></ml:eval></math></region><region top=\"5912.63965\" width=\"85\" left=\"748.8\" height=\"22\" converted-from=\"Mathcad14\" region-id=\"174\"><math><ml:eval><ml:id xml:space=\"preserve\"><Span xmlns=\"http://schemas.microsoft.com/winfx/2006/xaml/presentation\" xmlns:pw=\"clr-namespace:Ptc.Wpf;assembly=Ptc.Core\">H<pw:Subscript>FlocPort</pw:Subscript></Span></ml:id><ml:result /></ml:eval></math></region><region top=\"6027.84\" width=\"65\" left=\"28.8\" height=\"22\" converted-from=\"Mathcad14\" region-id=\"175\"><math><ml:eval><ml:id xml:space=\"preserve\"><Span xmlns=\"http://schemas.microsoft.com/winfx/2006/xaml/presentation\" xmlns:pw=\"clr-namespace:Ptc.Wpf;assembly=Ptc.Core\">Ti<pw:Subscript>Floc</pw:Subscript></Span></ml:id><ml:result /></ml:eval></math></region><region top=\"6027.84\" width=\"206.4\" left=\"172.8\" height=\"16\" converted-from=\"Mathcad14\" region-id=\"176\"><text><FlowDocument FontFamily=\"Tahoma\" FontStyle=\"Normal\" FontWeight=\"Normal\" FontSize=\"14.6666666666667\" Foreground=\"#FF000000\" Background=\"#00FFFFFF\" PagePadding=\"5,0,5,0\" AllowDrop=\"True\" Typography.Variants=\"Normal\" xmlns=\"http://schemas.microsoft.com/winfx/2006/xaml/presentation\"><Paragraph TextAlignment=\"Left\"><Run FontFamily=\"Arial\" FontStyle=\"Normal\" FontWeight=\"Normal\" FontSize=\"13.3333333333333\" Typography.Variants=\"Normal\"><Run.TextDecorations><TextDecorationCollection /></Run.TextDecorations>residence time of the flocculator</Run></Paragraph></FlowDocument></text></region><region top=\"6056.63965\" width=\"101\" left=\"28.8\" height=\"22\" converted-from=\"Mathcad14\" region-id=\"177\"><math><ml:eval><ml:id xml:space=\"preserve\"><Span xmlns=\"http://schemas.microsoft.com/winfx/2006/xaml/presentation\" xmlns:pw=\"clr-namespace:Ptc.Wpf;assembly=Ptc.Core\">N<pw:Subscript>FlocBaffles</pw:Subscript></Span></ml:id><ml:result /></ml:eval></math></region><region top=\"6056.63965\" width=\"109\" left=\"470.4\" height=\"22\" converted-from=\"Mathcad14\" region-id=\"178\"><math><ml:eval><ml:id xml:space=\"preserve\"><Span xmlns=\"http://schemas.microsoft.com/winfx/2006/xaml/presentation\" xmlns:pw=\"clr-namespace:Ptc.Wpf;assembly=Ptc.Core\">ND<pw:Subscript>FlocValve</pw:Subscript></Span></ml:id><ml:unitOverride><ml:id label=\"Unit\" xml:space=\"preserve\">in</ml:id></ml:unitOverride><ml:result /></ml:eval></math></region><region top=\"6104.63965\" width=\"102\" left=\"28.8\" height=\"22\" converted-from=\"Mathcad14\" region-id=\"179\"><math><ml:eval><ml:id xml:space=\"preserve\"><Span xmlns=\"http://schemas.microsoft.com/winfx/2006/xaml/presentation\" xmlns:pw=\"clr-namespace:Ptc.Wpf;assembly=Ptc.Core\">EN<pw:Subscript>FlocBaffle</pw:Subscript></Span></ml:id><ml:result /></ml:eval></math></region><region top=\"6165.84\" width=\"832\" left=\"0\" height=\"19.2\" region-id=\"180\"><text is-text-block=\"true\"><FlowDocument FontFamily=\"Mathcad UniMath\" xmlns=\"http://schemas.microsoft.com/winfx/2006/xaml/presentation\"><Paragraph xml:space=\"preserve\">---↑  ---</Paragraph></FlowDocument></text></region><region top=\"6265.68\" width=\"301\" left=\"19.2\" height=\"19\" converted-from=\"Mathcad14\" region-id=\"181\"><text><FlowDocument FontFamily=\"Tahoma\" FontStyle=\"Normal\" FontWeight=\"Normal\" FontSize=\"14.6666666666667\" Foreground=\"#FF000000\" Background=\"#00FFFFFF\" PagePadding=\"5,0,5,0\" AllowDrop=\"True\" Typography.Variants=\"Normal\" xmlns=\"http://schemas.microsoft.com/winfx/2006/xaml/presentation\"><Paragraph TextAlignment=\"Left\"><Run FontFamily=\"Arial\" FontStyle=\"Normal\" FontWeight=\"Bold\" FontSize=\"16\" Foreground=\"#FF008000\" Typography.Variants=\"Normal\"><Run.TextDecorations><TextDecorationCollection /></Run.TextDecorations>Sed Tanks</Run></Paragraph></FlowDocument></text></region><region top=\"6275.28027\" width=\"832\" left=\"0\" height=\"19.2\" region-id=\"182\"><text is-text-block=\"true\"><FlowDocument FontFamily=\"Mathcad UniMath\" xmlns=\"http://schemas.microsoft.com/winfx/2006/xaml/presentation\"><Paragraph xml:space=\"preserve\">---↓  ---</Paragraph></FlowDocument></text><mc14-conversion-loss-annotations><annotation>CollapsedArea</annotation></mc14-conversion-loss-annotations></region><region top=\"6346.32\" width=\"94\" left=\"38.4\" height=\"22\" converted-from=\"Mathcad14\" region-id=\"183\"><math><ml:eval><ml:id xml:space=\"preserve\"><Span xmlns=\"http://schemas.microsoft.com/winfx/2006/xaml/presentation\" xmlns:pw=\"clr-namespace:Ptc.Wpf;assembly=Ptc.Core\">N<pw:Subscript>SedTanks</pw:Subscript></Span></ml:id><ml:result /></ml:eval></math></region><region top=\"6394.32\" width=\"59\" left=\"38.4\" height=\"22\" converted-from=\"Mathcad14\" region-id=\"184\"><math><ml:eval><ml:id xml:space=\"preserve\"><Span xmlns=\"http://schemas.microsoft.com/winfx/2006/xaml/presentation\" xmlns:pw=\"clr-namespace:Ptc.Wpf;assembly=Ptc.Core\">L<pw:Subscript>Sed</pw:Subscript></Span></ml:id><ml:result /></ml:eval></math></region><region top=\"6432.71973\" width=\"88\" left=\"38.4\" height=\"22\" converted-from=\"Mathcad14\" region-id=\"185\"><math><ml:eval><ml:id xml:space=\"preserve\"><Span xmlns=\"http://schemas.microsoft.com/winfx/2006/xaml/presentation\" xmlns:pw=\"clr-namespace:Ptc.Wpf;assembly=Ptc.Core\">N<pw:Subscript>SedBays</pw:Subscript></Span></ml:id><ml:result /></ml:eval></math></region><region top=\"6442.32\" width=\"319.36\" left=\"182.4\" height=\"16\" converted-from=\"Mathcad14\" region-id=\"186\"><text><FlowDocument FontFamily=\"Tahoma\" FontStyle=\"Normal\" FontWeight=\"Normal\" FontSize=\"14.6666666666667\" Foreground=\"#FF000000\" Background=\"#00FFFFFF\" PagePadding=\"5,0,5,0\" AllowDrop=\"True\" Typography.Variants=\"Normal\" xmlns=\"http://schemas.microsoft.com/winfx/2006/xaml/presentation\"><Paragraph TextAlignment=\"Left\"><Run FontFamily=\"Arial\" FontStyle=\"Normal\" FontWeight=\"Normal\" FontSize=\"13.3333333333333\" Typography.Variants=\"Normal\"><Run.TextDecorations><TextDecorationCollection /></Run.TextDecorations>Number of bays of inlet manifolds in each sed tank</Run></Paragraph></FlowDocument></text></region><region top=\"6499.92\" width=\"81\" left=\"38.4\" height=\"22\" converted-from=\"Mathcad14\" region-id=\"187\"><math><ml:eval><ml:id xml:space=\"preserve\"><Span xmlns=\"http://schemas.microsoft.com/winfx/2006/xaml/presentation\" xmlns:pw=\"clr-namespace:Ptc.Wpf;assembly=Ptc.Core\">Q<pw:Subscript>SedBay</pw:Subscript></Span></ml:id><ml:result /></ml:eval></math></region><region top=\"6547.92\" width=\"156\" left=\"38.4\" height=\"37\" converted-from=\"Mathcad14\" region-id=\"188\"><math resultRef=\"-25\"><ml:eval><ml:id xml:space=\"preserve\"><Span xmlns=\"http://schemas.microsoft.com/winfx/2006/xaml/presentation\" xmlns:pw=\"clr-namespace:Ptc.Wpf;assembly=Ptc.Core\">V<pw:Subscript>SedUpBod</pw:Subscript></Span></ml:id><ml:result /></ml:eval></math></region><region top=\"6557.52051\" width=\"124.84\" left=\"268.8\" height=\"16\" converted-from=\"Mathcad14\" region-id=\"189\"><text><FlowDocument FontFamily=\"Tahoma\" FontStyle=\"Normal\" FontWeight=\"Normal\" FontSize=\"14.6666666666667\" Foreground=\"#FF000000\" Background=\"#00FFFFFF\" PagePadding=\"5,0,5,0\" AllowDrop=\"True\" Typography.Variants=\"Normal\" xmlns=\"http://schemas.microsoft.com/winfx/2006/xaml/presentation\"><Paragraph TextAlignment=\"Left\"><Run FontFamily=\"Arial\" FontStyle=\"Normal\" FontWeight=\"Normal\" FontSize=\"13.3333333333333\" Typography.Variants=\"Normal\"><Run.TextDecorations><TextDecorationCollection /></Run.TextDecorations>design constraints</Run></Paragraph></FlowDocument></text></region><region top=\"6605.52051\" width=\"157\" left=\"38.4\" height=\"37\" converted-from=\"Mathcad14\" region-id=\"190\"><math resultRef=\"-26\"><ml:eval><ml:id xml:space=\"preserve\"><Span xmlns=\"http://schemas.microsoft.com/winfx/2006/xaml/presentation\" xmlns:pw=\"clr-namespace:Ptc.Wpf;assembly=Ptc.Core\">V<pw:Subscript>SedCBod</pw:Subscript></Span></ml:id><ml:result /></ml:eval></math></region><region top=\"6663.12\" width=\"75\" left=\"38.4\" height=\"22\" converted-from=\"Mathcad14\" region-id=\"191\"><math><ml:eval><ml:id xml:space=\"preserve\"><Span xmlns=\"http://schemas.microsoft.com/winfx/2006/xaml/presentation\" xmlns:pw=\"clr-namespace:Ptc.Wpf;assembly=Ptc.Core\">V<pw:Subscript>SedUp</pw:Subscript></Span></ml:id><ml:result /></ml:eval></math></region><region top=\"6663.12\" width=\"194.3\" left=\"230.4\" height=\"16\" converted-from=\"Mathcad14\" region-id=\"192\"><text><FlowDocument FontFamily=\"Tahoma\" FontStyle=\"Normal\" FontWeight=\"Normal\" FontSize=\"14.6666666666667\" Foreground=\"#FF000000\" Background=\"#00FFFFFF\" PagePadding=\"5,0,5,0\" AllowDrop=\"True\" Typography.Variants=\"Normal\" xmlns=\"http://schemas.microsoft.com/winfx/2006/xaml/presentation\"><Paragraph TextAlignment=\"Left\"><Run FontFamily=\"Arial\" FontStyle=\"Normal\" FontWeight=\"Normal\" FontSize=\"13.3333333333333\" Typography.Variants=\"Normal\"><Run.TextDecorations><TextDecorationCollection /></Run.TextDecorations>Actual values from this design</Run></Paragraph></FlowDocument></text></region><region top=\"6720.72\" width=\"67\" left=\"38.4\" height=\"22\" converted-from=\"Mathcad14\" region-id=\"193\"><math><ml:eval><ml:id xml:space=\"preserve\"><Span xmlns=\"http://schemas.microsoft.com/winfx/2006/xaml/presentation\" xmlns:pw=\"clr-namespace:Ptc.Wpf;assembly=Ptc.Core\">V<pw:Subscript>SedC</pw:Subscript></Span></ml:id><ml:result /></ml:eval></math></region><region top=\"6778.32031\" width=\"123\" left=\"38.4\" height=\"22\" converted-from=\"Mathcad14\" region-id=\"194\"><math><ml:eval><ml:id xml:space=\"preserve\"><Span xmlns=\"http://schemas.microsoft.com/winfx/2006/xaml/presentation\" xmlns:pw=\"clr-namespace:Ptc.Wpf;assembly=Ptc.Core\">W<pw:Subscript>SedSideSlopes</pw:Subscript></Span></ml:id><ml:result /></ml:eval></math></region><region top=\"6826.32031\" width=\"121\" left=\"38.4\" height=\"22\" converted-from=\"Mathcad14\" region-id=\"195\"><math resultRef=\"-27\"><ml:eval><ml:id xml:space=\"preserve\"><Span xmlns=\"http://schemas.microsoft.com/winfx/2006/xaml/presentation\" xmlns:pw=\"clr-namespace:Ptc.Wpf;assembly=Ptc.Core\">AN<pw:Subscript>SedSlope</pw:Subscript></Span></ml:id><ml:result /></ml:eval></math></region><region top=\"6883.92041\" width=\"63\" left=\"38.4\" height=\"22\" converted-from=\"Mathcad14\" region-id=\"196\"><math><ml:eval><ml:id xml:space=\"preserve\"><Span xmlns=\"http://schemas.microsoft.com/winfx/2006/xaml/presentation\" xmlns:pw=\"clr-namespace:Ptc.Wpf;assembly=Ptc.Core\">Ti<pw:Subscript>Sed</pw:Subscript></Span></ml:id><ml:result /></ml:eval></math></region><region top=\"6941.52051\" width=\"275.44\" left=\"19.2\" height=\"19\" converted-from=\"Mathcad14\" region-id=\"197\"><text><FlowDocument FontFamily=\"Tahoma\" FontStyle=\"Normal\" FontWeight=\"Normal\" FontSize=\"14.6666666666667\" Foreground=\"#FF000000\" Background=\"#00FFFFFF\" PagePadding=\"5,0,5,0\" AllowDrop=\"True\" Typography.Variants=\"Normal\" xmlns=\"http://schemas.microsoft.com/winfx/2006/xaml/presentation\"><Paragraph TextAlignment=\"Left\"><Run FontFamily=\"Arial\" FontStyle=\"Normal\" FontWeight=\"Bold\" FontSize=\"16\" Foreground=\"#FF008000\" Typography.Variants=\"Normal\"><Run.TextDecorations><TextDecorationCollection /></Run.TextDecorations>Sedimentation Tank Sludge Drain:</Run></Paragraph></FlowDocument></text></region><region top=\"6960.72\" width=\"139\" left=\"28.8\" height=\"22\" converted-from=\"Mathcad14\" region-id=\"198\"><math><ml:eval><ml:id xml:space=\"preserve\"><Span xmlns=\"http://schemas.microsoft.com/winfx/2006/xaml/presentation\" xmlns:pw=\"clr-namespace:Ptc.Wpf;assembly=Ptc.Core\">N<pw:Subscript>SedSludgeOrifices</pw:Subscript></Span></ml:id><ml:result /></ml:eval></math></region><region top=\"6970.32031\" width=\"59.44\" left=\"230.4\" height=\"16\" converted-from=\"Mathcad14\" region-id=\"199\"><text><FlowDocument FontFamily=\"Tahoma\" FontStyle=\"Normal\" FontWeight=\"Normal\" FontSize=\"14.6666666666667\" Foreground=\"#FF000000\" Background=\"#00FFFFFF\" PagePadding=\"5,0,5,0\" AllowDrop=\"True\" Typography.Variants=\"Normal\" xmlns=\"http://schemas.microsoft.com/winfx/2006/xaml/presentation\"><Paragraph TextAlignment=\"Left\"><Run FontFamily=\"Arial\" FontStyle=\"Normal\" FontWeight=\"Normal\" FontSize=\"13.3333333333333\" Typography.Variants=\"Normal\"><Run.TextDecorations><TextDecorationCollection /></Run.TextDecorations>per cell</Run></Paragraph></FlowDocument></text></region><region top=\"6970.32031\" width=\"158\" left=\"643.2\" height=\"30\" converted-from=\"Mathcad14\" region-id=\"200\"><math resultRef=\"-28\"><ml:eval><ml:id xml:space=\"preserve\"><Span xmlns=\"http://schemas.microsoft.com/winfx/2006/xaml/presentation\" xmlns:pw=\"clr-namespace:Ptc.Wpf;assembly=Ptc.Core\">Ti<pw:Subscript>SludgeDrain</pw:Subscript></Span></ml:id><ml:result /></ml:eval></math></region><region top=\"6970.32031\" width=\"109.56\" left=\"864\" height=\"16\" converted-from=\"Mathcad14\" region-id=\"201\"><text><FlowDocument FontFamily=\"Tahoma\" FontStyle=\"Normal\" FontWeight=\"Normal\" FontSize=\"14.6666666666667\" Foreground=\"#FF000000\" Background=\"#00FFFFFF\" PagePadding=\"5,0,5,0\" AllowDrop=\"True\" Typography.Variants=\"Normal\" xmlns=\"http://schemas.microsoft.com/winfx/2006/xaml/presentation\"><Paragraph TextAlignment=\"Left\"><Run FontFamily=\"Arial\" FontStyle=\"Normal\" FontWeight=\"Normal\" FontSize=\"13.3333333333333\" Typography.Variants=\"Normal\"><Run.TextDecorations><TextDecorationCollection /></Run.TextDecorations>Tank Drain time</Run></Paragraph></FlowDocument></text></region><region top=\"6999.12\" width=\"101\" left=\"28.8\" height=\"22\" converted-from=\"Mathcad14\" region-id=\"202\"><math><ml:eval><ml:id xml:space=\"preserve\"><Span xmlns=\"http://schemas.microsoft.com/winfx/2006/xaml/presentation\" xmlns:pw=\"clr-namespace:Ptc.Wpf;assembly=Ptc.Core\">W<pw:Subscript>SedSludge</pw:Subscript></Span></ml:id><ml:result /></ml:eval></math></region><region top=\"6999.12\" width=\"181.1\" left=\"230.4\" height=\"16\" converted-from=\"Mathcad14\" region-id=\"203\"><text><FlowDocument FontFamily=\"Tahoma\" FontStyle=\"Normal\" FontWeight=\"Normal\" FontSize=\"14.6666666666667\" Foreground=\"#FF000000\" Background=\"#00FFFFFF\" PagePadding=\"5,0,5,0\" AllowDrop=\"True\" Typography.Variants=\"Normal\" xmlns=\"http://schemas.microsoft.com/winfx/2006/xaml/presentation\"><Paragraph TextAlignment=\"Left\"><Run FontFamily=\"Arial\" FontStyle=\"Normal\" FontWeight=\"Normal\" FontSize=\"13.3333333333333\" Typography.Variants=\"Normal\"><Run.TextDecorations><TextDecorationCollection /></Run.TextDecorations>Width of the sludge channel</Run></Paragraph></FlowDocument></text></region><region top=\"7018.32031\" width=\"184.32\" left=\"230.4\" height=\"16\" converted-from=\"Mathcad14\" region-id=\"204\"><text><FlowDocument FontFamily=\"Tahoma\" FontStyle=\"Normal\" FontWeight=\"Normal\" FontSize=\"14.6666666666667\" Foreground=\"#FF000000\" Background=\"#00FFFFFF\" PagePadding=\"5,0,5,0\" AllowDrop=\"True\" Typography.Variants=\"Normal\" xmlns=\"http://schemas.microsoft.com/winfx/2006/xaml/presentation\"><Paragraph TextAlignment=\"Left\"><Run FontFamily=\"Arial\" FontStyle=\"Normal\" FontWeight=\"Normal\" FontSize=\"13.3333333333333\" Typography.Variants=\"Normal\"><Run.TextDecorations><TextDecorationCollection /></Run.TextDecorations>Depth of the sludge channel</Run></Paragraph></FlowDocument></text></region><region top=\"7027.92041\" width=\"97\" left=\"28.8\" height=\"22\" converted-from=\"Mathcad14\" region-id=\"205\"><math><ml:eval><ml:id xml:space=\"preserve\"><Span xmlns=\"http://schemas.microsoft.com/winfx/2006/xaml/presentation\" xmlns:pw=\"clr-namespace:Ptc.Wpf;assembly=Ptc.Core\">H<pw:Subscript>SedSludge</pw:Subscript></Span></ml:id><ml:result /></ml:eval></math></region><region top=\"7027.92041\" width=\"298.78\" left=\"864\" height=\"16\" converted-from=\"Mathcad14\" region-id=\"206\"><text><FlowDocument FontFamily=\"Tahoma\" FontStyle=\"Normal\" FontWeight=\"Normal\" FontSize=\"14.6666666666667\" Foreground=\"#FF000000\" Background=\"#00FFFFFF\" PagePadding=\"5,0,5,0\" AllowDrop=\"True\" Typography.Variants=\"Normal\" xmlns=\"http://schemas.microsoft.com/winfx/2006/xaml/presentation\"><Paragraph TextAlignment=\"Left\"><Run FontFamily=\"Arial\" FontStyle=\"Normal\" FontWeight=\"Normal\" FontSize=\"13.3333333333333\" Typography.Variants=\"Normal\"><Run.TextDecorations><TextDecorationCollection /></Run.TextDecorations>Distance center to center between drain orifices</Run></Paragraph></FlowDocument></text></region><region top=\"7037.52051\" width=\"137\" left=\"643.2\" height=\"22\" converted-from=\"Mathcad14\" region-id=\"207\"><math><ml:eval><ml:id xml:space=\"preserve\"><Span xmlns=\"http://schemas.microsoft.com/winfx/2006/xaml/presentation\" xmlns:pw=\"clr-namespace:Ptc.Wpf;assembly=Ptc.Core\">B<pw:Subscript>SedSludgeOrifices</pw:Subscript></Span></ml:id><ml:result /></ml:eval></math></region><region top=\"7085.52051\" width=\"126\" left=\"643.2\" height=\"22\" converted-from=\"Mathcad14\" region-id=\"208\"><math><ml:eval><ml:id xml:space=\"preserve\"><Span xmlns=\"http://schemas.microsoft.com/winfx/2006/xaml/presentation\" xmlns:pw=\"clr-namespace:Ptc.Wpf;assembly=Ptc.Core\">W<pw:Subscript>SedDrainCover</pw:Subscript></Span></ml:id><ml:result /></ml:eval></math></region><region top=\"7104.72\" width=\"132\" left=\"28.8\" height=\"22\" converted-from=\"Mathcad14\" region-id=\"209\"><math><ml:eval><ml:id xml:space=\"preserve\"><Span xmlns=\"http://schemas.microsoft.com/winfx/2006/xaml/presentation\" xmlns:pw=\"clr-namespace:Ptc.Wpf;assembly=Ptc.Core\">D<pw:Subscript>SedSludgeOrifice</pw:Subscript></Span></ml:id><ml:result /></ml:eval></math></region><region top=\"7114.32031\" width=\"167.02\" left=\"288\" height=\"16\" converted-from=\"Mathcad14\" region-id=\"210\"><text><FlowDocument FontFamily=\"Tahoma\" FontStyle=\"Normal\" FontWeight=\"Normal\" FontSize=\"14.6666666666667\" Foreground=\"#FF000000\" Background=\"#00FFFFFF\" PagePadding=\"5,0,5,0\" AllowDrop=\"True\" Typography.Variants=\"Normal\" xmlns=\"http://schemas.microsoft.com/winfx/2006/xaml/presentation\"><Paragraph TextAlignment=\"Left\"><Run FontFamily=\"Arial\" FontStyle=\"Normal\" FontWeight=\"Normal\" FontSize=\"13.3333333333333\" Typography.Variants=\"Normal\"><Run.TextDecorations><TextDecorationCollection /></Run.TextDecorations>Diameter of drain orifices</Run></Paragraph></FlowDocument></text></region><region top=\"7152.72\" width=\"139\" left=\"28.8\" height=\"22\" converted-from=\"Mathcad14\" region-id=\"211\"><math><ml:eval><ml:id xml:space=\"preserve\"><Span xmlns=\"http://schemas.microsoft.com/winfx/2006/xaml/presentation\" xmlns:pw=\"clr-namespace:Ptc.Wpf;assembly=Ptc.Core\">N<pw:Subscript>SedSludgeOrifices</pw:Subscript></Span></ml:id><ml:result /></ml:eval></math></region><region top=\"7191.12\" width=\"130\" left=\"28.8\" height=\"22\" converted-from=\"Mathcad14\" region-id=\"212\"><math><ml:eval><ml:id xml:space=\"preserve\"><Span xmlns=\"http://schemas.microsoft.com/winfx/2006/xaml/presentation\" xmlns:pw=\"clr-namespace:Ptc.Wpf;assembly=Ptc.Core\">ND<pw:Subscript>SedSludgePipe</pw:Subscript></Span></ml:id><ml:result /></ml:eval></math></region><region top=\"7258.32031\" width=\"398\" left=\"9.6\" height=\"19\" converted-from=\"Mathcad14\" region-id=\"213\"><text><FlowDocument FontFamily=\"Tahoma\" FontStyle=\"Normal\" FontWeight=\"Normal\" FontSize=\"14.6666666666667\" Foreground=\"#FF000000\" Background=\"#00FFFFFF\" PagePadding=\"5,0,5,0\" AllowDrop=\"True\" Typography.Variants=\"Normal\" xmlns=\"http://schemas.microsoft.com/winfx/2006/xaml/presentation\"><Paragraph TextAlignment=\"Left\"><Run FontFamily=\"Arial\" FontStyle=\"Normal\" FontWeight=\"Bold\" FontSize=\"16\" Foreground=\"#FF008000\" Typography.Variants=\"Normal\"><Run.TextDecorations><TextDecorationCollection /></Run.TextDecorations>Sedimentation Tank Dimensions:</Run></Paragraph></FlowDocument></text></region><region top=\"7287.12\" width=\"96\" left=\"28.8\" height=\"22\" converted-from=\"Mathcad14\" region-id=\"214\"><math><ml:eval><ml:id xml:space=\"preserve\"><Span xmlns=\"http://schemas.microsoft.com/winfx/2006/xaml/presentation\" xmlns:pw=\"clr-namespace:Ptc.Wpf;assembly=Ptc.Core\">Z<pw:Subscript>SedSludge</pw:Subscript></Span></ml:id><ml:result /></ml:eval></math></region><region top=\"7287.12\" width=\"273.5\" left=\"230.4\" height=\"16\" converted-from=\"Mathcad14\" region-id=\"215\"><text><FlowDocument FontFamily=\"Tahoma\" FontStyle=\"Normal\" FontWeight=\"Normal\" FontSize=\"14.6666666666667\" Foreground=\"#FF000000\" Background=\"#00FFFFFF\" PagePadding=\"5,0,5,0\" AllowDrop=\"True\" Typography.Variants=\"Normal\" xmlns=\"http://schemas.microsoft.com/winfx/2006/xaml/presentation\"><Paragraph TextAlignment=\"Left\"><Run FontFamily=\"Arial\" FontStyle=\"Normal\" FontWeight=\"Normal\" FontSize=\"13.3333333333333\" Typography.Variants=\"Normal\"><Run.TextDecorations><TextDecorationCollection /></Run.TextDecorations>Height from 0 of the top of the sludge drain</Run></Paragraph></FlowDocument></text></region><region top=\"7344.72\" width=\"118\" left=\"28.8\" height=\"22\" converted-from=\"Mathcad14\" region-id=\"216\"><math><ml:eval><ml:id xml:space=\"preserve\"><Span xmlns=\"http://schemas.microsoft.com/winfx/2006/xaml/presentation\" xmlns:pw=\"clr-namespace:Ptc.Wpf;assembly=Ptc.Core\">Z<pw:Subscript>SedSideSlopes</pw:Subscript></Span></ml:id><ml:result /></ml:eval></math></region><region top=\"7392.72\" width=\"140.64\" left=\"230.4\" height=\"16\" converted-from=\"Mathcad14\" region-id=\"217\"><text><FlowDocument FontFamily=\"Tahoma\" FontStyle=\"Normal\" FontWeight=\"Normal\" FontSize=\"14.6666666666667\" Foreground=\"#FF000000\" Background=\"#00FFFFFF\" PagePadding=\"5,0,5,0\" AllowDrop=\"True\" Typography.Variants=\"Normal\" xmlns=\"http://schemas.microsoft.com/winfx/2006/xaml/presentation\"><Paragraph TextAlignment=\"Left\"><Run FontFamily=\"Arial\" FontStyle=\"Normal\" FontWeight=\"Normal\" FontSize=\"13.3333333333333\" Typography.Variants=\"Normal\"><Run.TextDecorations><TextDecorationCollection /></Run.TextDecorations>Total tank wall height</Run></Paragraph></FlowDocument></text></region><region top=\"7402.32031\" width=\"65\" left=\"28.8\" height=\"22\" converted-from=\"Mathcad14\" region-id=\"218\"><math><ml:eval><ml:id xml:space=\"preserve\"><Span xmlns=\"http://schemas.microsoft.com/winfx/2006/xaml/presentation\" xmlns:pw=\"clr-namespace:Ptc.Wpf;assembly=Ptc.Core\">W<pw:Subscript>Sed</pw:Subscript></Span></ml:id><ml:result /></ml:eval></math></region><region top=\"7431.12\" width=\"59\" left=\"28.8\" height=\"22\" converted-from=\"Mathcad14\" region-id=\"219\"><math><ml:eval><ml:id xml:space=\"preserve\"><Span xmlns=\"http://schemas.microsoft.com/winfx/2006/xaml/presentation\" xmlns:pw=\"clr-namespace:Ptc.Wpf;assembly=Ptc.Core\">L<pw:Subscript>Sed</pw:Subscript></Span></ml:id><ml:result /></ml:eval></math></region><region top=\"7431.12\" width=\"113.44\" left=\"230.4\" height=\"16\" converted-from=\"Mathcad14\" region-id=\"220\"><text><FlowDocument FontFamily=\"Tahoma\" FontStyle=\"Normal\" FontWeight=\"Normal\" FontSize=\"14.6666666666667\" Foreground=\"#FF000000\" Background=\"#00FFFFFF\" PagePadding=\"5,0,5,0\" AllowDrop=\"True\" Typography.Variants=\"Normal\" xmlns=\"http://schemas.microsoft.com/winfx/2006/xaml/presentation\"><Paragraph TextAlignment=\"Left\"><Run FontFamily=\"Arial\" FontStyle=\"Normal\" FontWeight=\"Normal\" FontSize=\"13.3333333333333\" Typography.Variants=\"Normal\"><Run.TextDecorations><TextDecorationCollection /></Run.TextDecorations>Total tank length</Run></Paragraph></FlowDocument></text></region><region top=\"7469.52051\" width=\"61\" left=\"28.8\" height=\"22\" converted-from=\"Mathcad14\" region-id=\"221\"><math><ml:eval><ml:id xml:space=\"preserve\"><Span xmlns=\"http://schemas.microsoft.com/winfx/2006/xaml/presentation\" xmlns:pw=\"clr-namespace:Ptc.Wpf;assembly=Ptc.Core\">H<pw:Subscript>Sed</pw:Subscript></Span></ml:id><ml:result /></ml:eval></math></region><region top=\"7527.12\" width=\"280\" left=\"19.2\" height=\"19\" converted-from=\"Mathcad14\" region-id=\"222\"><text><FlowDocument FontFamily=\"Tahoma\" FontStyle=\"Normal\" FontWeight=\"Normal\" FontSize=\"14.6666666666667\" Foreground=\"#FF000000\" Background=\"#00FFFFFF\" PagePadding=\"5,0,5,0\" AllowDrop=\"True\" Typography.Variants=\"Normal\" xmlns=\"http://schemas.microsoft.com/winfx/2006/xaml/presentation\"><Paragraph TextAlignment=\"Left\"><Run FontFamily=\"Arial\" FontStyle=\"Normal\" FontWeight=\"Bold\" FontSize=\"16\" Foreground=\"#FF008000\" Typography.Variants=\"Normal\"><Run.TextDecorations><TextDecorationCollection /></Run.TextDecorations>Sedimentation Tank Inlet Channel:</Run></Paragraph></FlowDocument></text></region><region top=\"7565.52051\" width=\"146\" left=\"288\" height=\"22\" converted-from=\"Mathcad14\" region-id=\"223\"><math><ml:eval><ml:id xml:space=\"preserve\"><Span xmlns=\"http://schemas.microsoft.com/winfx/2006/xaml/presentation\" xmlns:pw=\"clr-namespace:Ptc.Wpf;assembly=Ptc.Core\">EN<pw:Subscript>InletChannelGeom</pw:Subscript></Span></ml:id><ml:result /></ml:eval></math></region><region top=\"7575.12\" width=\"142\" left=\"28.8\" height=\"22\" converted-from=\"Mathcad14\" region-id=\"224\"><math><ml:eval><ml:id xml:space=\"preserve\"><Span xmlns=\"http://schemas.microsoft.com/winfx/2006/xaml/presentation\" xmlns:pw=\"clr-namespace:Ptc.Wpf;assembly=Ptc.Core\">HW<pw:Subscript>SedInletChannel</pw:Subscript></Span></ml:id><ml:result /></ml:eval></math></region><region top=\"7613.52051\" width=\"133\" left=\"28.8\" height=\"22\" converted-from=\"Mathcad14\" region-id=\"225\"><math><ml:eval><ml:id xml:space=\"preserve\"><Span xmlns=\"http://schemas.microsoft.com/winfx/2006/xaml/presentation\" xmlns:pw=\"clr-namespace:Ptc.Wpf;assembly=Ptc.Core\">W<pw:Subscript>SedInletChannel</pw:Subscript></Span></ml:id><ml:result /></ml:eval></math></region><region top=\"7651.92041\" width=\"103\" left=\"28.8\" height=\"22\" converted-from=\"Mathcad14\" region-id=\"226\"><math><ml:eval><ml:id xml:space=\"preserve\"><Span xmlns=\"http://schemas.microsoft.com/winfx/2006/xaml/presentation\" xmlns:pw=\"clr-namespace:Ptc.Wpf;assembly=Ptc.Core\">L<pw:Subscript>SedChannel</pw:Subscript></Span></ml:id><ml:result /></ml:eval></math></region><region top=\"7699.92041\" width=\"129\" left=\"28.8\" height=\"22\" converted-from=\"Mathcad14\" region-id=\"227\"><math><ml:eval><ml:id xml:space=\"preserve\"><Span xmlns=\"http://schemas.microsoft.com/winfx/2006/xaml/presentation\" xmlns:pw=\"clr-namespace:Ptc.Wpf;assembly=Ptc.Core\">H<pw:Subscript>SedInletChannel</pw:Subscript></Span></ml:id><ml:result /></ml:eval></math></region><region top=\"7699.92041\" width=\"117\" left=\"345.6\" height=\"22\" converted-from=\"Mathcad14\" region-id=\"228\"><math><ml:eval><ml:id xml:space=\"preserve\"><Span xmlns=\"http://schemas.microsoft.com/winfx/2006/xaml/presentation\" xmlns:pw=\"clr-namespace:Ptc.Wpf;assembly=Ptc.Core\">HL<pw:Subscript>SedWeirInlet</pw:Subscript></Span></ml:id><ml:result /></ml:eval></math></region><region top=\"7747.92041\" width=\"176\" left=\"28.8\" height=\"22\" converted-from=\"Mathcad14\" region-id=\"229\"><math><ml:eval><ml:id xml:space=\"preserve\"><Span xmlns=\"http://schemas.microsoft.com/winfx/2006/xaml/presentation\" xmlns:pw=\"clr-namespace:Ptc.Wpf;assembly=Ptc.Core\">W<pw:Subscript>SedInletChannelPreWeir</pw:Subscript></Span></ml:id><ml:result /></ml:eval></math></region><region top=\"7786.32031\" width=\"110\" left=\"28.8\" height=\"22\" converted-from=\"Mathcad14\" region-id=\"230\"><math><ml:eval><ml:id xml:space=\"preserve\"><Span xmlns=\"http://schemas.microsoft.com/winfx/2006/xaml/presentation\" xmlns:pw=\"clr-namespace:Ptc.Wpf;assembly=Ptc.Core\">H<pw:Subscript>SedWeirInlet</pw:Subscript></Span></ml:id><ml:result /></ml:eval></math></region><region top=\"7824.72\" width=\"114\" left=\"28.8\" height=\"22\" converted-from=\"Mathcad14\" region-id=\"231\"><math><ml:eval><ml:id xml:space=\"preserve\"><Span xmlns=\"http://schemas.microsoft.com/winfx/2006/xaml/presentation\" xmlns:pw=\"clr-namespace:Ptc.Wpf;assembly=Ptc.Core\">W<pw:Subscript>SedWeirInlet</pw:Subscript></Span></ml:id><ml:result /></ml:eval></math></region><region top=\"7891.92041\" width=\"304.56\" left=\"19.2\" height=\"19\" converted-from=\"Mathcad14\" region-id=\"232\"><text><FlowDocument FontFamily=\"Tahoma\" FontStyle=\"Normal\" FontWeight=\"Normal\" FontSize=\"14.6666666666667\" Foreground=\"#FF000000\" Background=\"#00FFFFFF\" PagePadding=\"5,0,5,0\" AllowDrop=\"True\" Typography.Variants=\"Normal\" xmlns=\"http://schemas.microsoft.com/winfx/2006/xaml/presentation\"><Paragraph TextAlignment=\"Left\"><Run FontFamily=\"Arial\" FontStyle=\"Normal\" FontWeight=\"Bold\" FontSize=\"16\" Foreground=\"#FF008000\" Typography.Variants=\"Normal\"><Run.TextDecorations><TextDecorationCollection /></Run.TextDecorations>Sedimentation Tank Effluent Launder:</Run></Paragraph></FlowDocument></text></region><region top=\"7939.92041\" width=\"146\" left=\"28.8\" height=\"22\" converted-from=\"Mathcad14\" region-id=\"233\"><math><ml:eval><ml:id xml:space=\"preserve\"><Span xmlns=\"http://schemas.microsoft.com/winfx/2006/xaml/presentation\" xmlns:pw=\"clr-namespace:Ptc.Wpf;assembly=Ptc.Core\">N<pw:Subscript>SedLaunderOrifices</pw:Subscript></Span></ml:id><ml:result /></ml:eval></math></region><region top=\"7949.52051\" width=\"196.64\" left=\"259.2\" height=\"16\" converted-from=\"Mathcad14\" region-id=\"234\"><text><FlowDocument FontFamily=\"Tahoma\" FontStyle=\"Normal\" FontWeight=\"Normal\" FontSize=\"14.6666666666667\" Foreground=\"#FF000000\" Background=\"#00FFFFFF\" PagePadding=\"5,0,5,0\" AllowDrop=\"True\" Typography.Variants=\"Normal\" xmlns=\"http://schemas.microsoft.com/winfx/2006/xaml/presentation\"><Paragraph TextAlignment=\"Left\"><Run FontFamily=\"Arial\" FontStyle=\"Normal\" FontWeight=\"Normal\" FontSize=\"13.3333333333333\" Typography.Variants=\"Normal\"><Run.TextDecorations><TextDecorationCollection /></Run.TextDecorations>Number of orifices per launder</Run></Paragraph></FlowDocument></text></region><region top=\"7987.92041\" width=\"170\" left=\"28.8\" height=\"22\" converted-from=\"Mathcad14\" region-id=\"235\"><math><ml:eval><ml:id xml:space=\"preserve\"><Span xmlns=\"http://schemas.microsoft.com/winfx/2006/xaml/presentation\" xmlns:pw=\"clr-namespace:Ptc.Wpf;assembly=Ptc.Core\">N<pw:Subscript>SedLaunderOrificesRow</pw:Subscript></Span></ml:id><ml:result /></ml:eval></math></region><region top=\"7987.92041\" width=\"175\" left=\"259.2\" height=\"16\" converted-from=\"Mathcad14\" region-id=\"236\"><text><FlowDocument FontFamily=\"Tahoma\" FontStyle=\"Normal\" FontWeight=\"Normal\" FontSize=\"14.6666666666667\" Foreground=\"#FF000000\" Background=\"#00FFFFFF\" PagePadding=\"5,0,5,0\" AllowDrop=\"True\" Typography.Variants=\"Normal\" xmlns=\"http://schemas.microsoft.com/winfx/2006/xaml/presentation\"><Paragraph TextAlignment=\"Left\"><Run FontFamily=\"Arial\" FontStyle=\"Normal\" FontWeight=\"Normal\" FontSize=\"13.3333333333333\" Typography.Variants=\"Normal\"><Run.TextDecorations><TextDecorationCollection /></Run.TextDecorations>Number of orifices per row</Run></Paragraph></FlowDocument></text></region><region top=\"8016.72\" width=\"104\" left=\"489.6\" height=\"22\" converted-from=\"Mathcad14\" region-id=\"237\"><math><ml:eval><ml:id xml:space=\"preserve\"><Span xmlns=\"http://schemas.microsoft.com/winfx/2006/xaml/presentation\" xmlns:pw=\"clr-namespace:Ptc.Wpf;assembly=Ptc.Core\">Z<pw:Subscript>SedLaunder</pw:Subscript></Span></ml:id><ml:result /></ml:eval></math></region><region top=\"8045.52051\" width=\"145\" left=\"28.8\" height=\"22\" converted-from=\"Mathcad14\" region-id=\"238\"><math><ml:eval><ml:id xml:space=\"preserve\"><Span xmlns=\"http://schemas.microsoft.com/winfx/2006/xaml/presentation\" xmlns:pw=\"clr-namespace:Ptc.Wpf;assembly=Ptc.Core\">Q<pw:Subscript>SedLaunderOrifices</pw:Subscript></Span></ml:id><ml:result /></ml:eval></math></region><region top=\"8083.92041\" width=\"164\" left=\"28.8\" height=\"22\" converted-from=\"Mathcad14\" region-id=\"239\"><math resultRef=\"-29\"><ml:eval><ml:id xml:space=\"preserve\"><Span xmlns=\"http://schemas.microsoft.com/winfx/2006/xaml/presentation\" xmlns:pw=\"clr-namespace:Ptc.Wpf;assembly=Ptc.Core\">B<pw:Subscript>SedLaunderOrifices</pw:Subscript></Span></ml:id><ml:result /></ml:eval></math></region><region top=\"8083.92041\" width=\"210.8\" left=\"259.2\" height=\"16\" converted-from=\"Mathcad14\" region-id=\"240\"><text><FlowDocument FontFamily=\"Tahoma\" FontStyle=\"Normal\" FontWeight=\"Normal\" FontSize=\"14.6666666666667\" Foreground=\"#FF000000\" Background=\"#00FFFFFF\" PagePadding=\"5,0,5,0\" AllowDrop=\"True\" Typography.Variants=\"Normal\" xmlns=\"http://schemas.microsoft.com/winfx/2006/xaml/presentation\"><Paragraph TextAlignment=\"Left\"><Run FontFamily=\"Arial\" FontStyle=\"Normal\" FontWeight=\"Normal\" FontSize=\"13.3333333333333\" Typography.Variants=\"Normal\"><Run.TextDecorations><TextDecorationCollection /></Run.TextDecorations>Center to center launder spacing</Run></Paragraph></FlowDocument></text></region><region top=\"8141.52051\" width=\"186.6\" left=\"38.4\" height=\"16\" converted-from=\"Mathcad14\" region-id=\"241\"><text><FlowDocument FontFamily=\"Tahoma\" FontStyle=\"Normal\" FontWeight=\"Normal\" FontSize=\"14.6666666666667\" Foreground=\"#FF000000\" Background=\"#00FFFFFF\" PagePadding=\"5,0,5,0\" AllowDrop=\"True\" Typography.Variants=\"Normal\" xmlns=\"http://schemas.microsoft.com/winfx/2006/xaml/presentation\"><Paragraph TextAlignment=\"Left\"><Run FontFamily=\"Arial\" FontStyle=\"Normal\" FontWeight=\"Bold\" FontSize=\"13.3333333333333\" Typography.Variants=\"Normal\"><Run.TextDecorations><TextDecorationCollection /></Run.TextDecorations>More Launder Dimensions</Run></Paragraph></FlowDocument></text></region><region top=\"8170.32031\" width=\"115\" left=\"38.4\" height=\"22\" converted-from=\"Mathcad14\" region-id=\"242\"><math><ml:eval><ml:id xml:space=\"preserve\"><Span xmlns=\"http://schemas.microsoft.com/winfx/2006/xaml/presentation\" xmlns:pw=\"clr-namespace:Ptc.Wpf;assembly=Ptc.Core\">ND<pw:Subscript>SedLaunder</pw:Subscript></Span></ml:id><ml:result /></ml:eval></math></region><region top=\"8208.721\" width=\"139\" left=\"38.4\" height=\"22\" converted-from=\"Mathcad14\" region-id=\"243\"><math><ml:eval><ml:id xml:space=\"preserve\"><Span xmlns=\"http://schemas.microsoft.com/winfx/2006/xaml/presentation\" xmlns:pw=\"clr-namespace:Ptc.Wpf;assembly=Ptc.Core\">D<pw:Subscript>SedLaunderOrifice</pw:Subscript></Span></ml:id><ml:result /></ml:eval></math></region><region top=\"8247.12\" width=\"103\" left=\"38.4\" height=\"22\" converted-from=\"Mathcad14\" region-id=\"244\"><math><ml:eval><ml:id xml:space=\"preserve\"><Span xmlns=\"http://schemas.microsoft.com/winfx/2006/xaml/presentation\" xmlns:pw=\"clr-namespace:Ptc.Wpf;assembly=Ptc.Core\">L<pw:Subscript>SedLaunder</pw:Subscript></Span></ml:id><ml:result /></ml:eval></math></region><region top=\"8285.52051\" width=\"146\" left=\"38.4\" height=\"22\" converted-from=\"Mathcad14\" region-id=\"245\"><math><ml:eval><ml:id xml:space=\"preserve\"><Span xmlns=\"http://schemas.microsoft.com/winfx/2006/xaml/presentation\" xmlns:pw=\"clr-namespace:Ptc.Wpf;assembly=Ptc.Core\">HL<pw:Subscript>SedLaunderOrifice</pw:Subscript></Span></ml:id><ml:result /></ml:eval></math></region><region top=\"8343.12\" width=\"293\" left=\"28.8\" height=\"19\" converted-from=\"Mathcad14\" region-id=\"246\"><text><FlowDocument FontFamily=\"Tahoma\" FontStyle=\"Normal\" FontWeight=\"Normal\" FontSize=\"14.6666666666667\" Foreground=\"#FF000000\" Background=\"#00FFFFFF\" PagePadding=\"5,0,5,0\" AllowDrop=\"True\" Typography.Variants=\"Normal\" xmlns=\"http://schemas.microsoft.com/winfx/2006/xaml/presentation\"><Paragraph TextAlignment=\"Left\"><Run FontFamily=\"Arial\" FontStyle=\"Normal\" FontWeight=\"Bold\" FontSize=\"16\" Foreground=\"#FF008000\" Typography.Variants=\"Normal\"><Run.TextDecorations><TextDecorationCollection /></Run.TextDecorations>Sedimentation Tank Inlet Manifold:</Run></Paragraph></FlowDocument></text></region><region top=\"8400.721\" width=\"120\" left=\"38.4\" height=\"22\" converted-from=\"Mathcad14\" region-id=\"247\"><math><ml:eval><ml:id xml:space=\"preserve\"><Span xmlns=\"http://schemas.microsoft.com/winfx/2006/xaml/presentation\" xmlns:pw=\"clr-namespace:Ptc.Wpf;assembly=Ptc.Core\">ND<pw:Subscript>SedManifold</pw:Subscript></Span></ml:id><ml:result /></ml:eval></math></region><region top=\"8400.721\" width=\"151\" left=\"345.6\" height=\"22\" converted-from=\"Mathcad14\" region-id=\"248\"><math><ml:eval><ml:id xml:space=\"preserve\"><Span xmlns=\"http://schemas.microsoft.com/winfx/2006/xaml/presentation\" xmlns:pw=\"clr-namespace:Ptc.Wpf;assembly=Ptc.Core\">L<pw:Subscript>SedManifoldDiffuser</pw:Subscript></Span></ml:id><ml:result /></ml:eval></math></region><region top=\"8448.721\" width=\"131\" left=\"38.4\" height=\"22\" converted-from=\"Mathcad14\" region-id=\"249\"><math><ml:eval><ml:id xml:space=\"preserve\"><Span xmlns=\"http://schemas.microsoft.com/winfx/2006/xaml/presentation\" xmlns:pw=\"clr-namespace:Ptc.Wpf;assembly=Ptc.Core\">Z<pw:Subscript>SedManifoldPipe</pw:Subscript></Span></ml:id><ml:result /></ml:eval></math></region><region top=\"8448.721\" width=\"146\" left=\"345.6\" height=\"22\" converted-from=\"Mathcad14\" region-id=\"250\"><math resultRef=\"-30\"><ml:eval><ml:id xml:space=\"preserve\"><Span xmlns=\"http://schemas.microsoft.com/winfx/2006/xaml/presentation\" xmlns:pw=\"clr-namespace:Ptc.Wpf;assembly=Ptc.Core\">ND<pw:Subscript>SedDiffuser</pw:Subscript></Span></ml:id><ml:result /></ml:eval></math></region><region top=\"8487.12\" width=\"131\" left=\"38.4\" height=\"22\" converted-from=\"Mathcad14\" region-id=\"251\"><math><ml:eval><ml:id xml:space=\"preserve\"><Span xmlns=\"http://schemas.microsoft.com/winfx/2006/xaml/presentation\" xmlns:pw=\"clr-namespace:Ptc.Wpf;assembly=Ptc.Core\">D<pw:Subscript>SedManifoldPort</pw:Subscript></Span></ml:id><ml:result /></ml:eval></math></region><region top=\"8496.721\" width=\"156\" left=\"345.6\" height=\"22\" converted-from=\"Mathcad14\" region-id=\"252\"><math resultRef=\"-31\"><ml:eval><ml:id xml:space=\"preserve\"><Span xmlns=\"http://schemas.microsoft.com/winfx/2006/xaml/presentation\" xmlns:pw=\"clr-namespace:Ptc.Wpf;assembly=Ptc.Core\">B<pw:Subscript>SedManifoldPort</pw:Subscript></Span></ml:id><ml:result /></ml:eval></math></region><region top=\"8535.12\" width=\"138\" left=\"38.4\" height=\"22\" converted-from=\"Mathcad14\" region-id=\"253\"><math><ml:eval><ml:id xml:space=\"preserve\"><Span xmlns=\"http://schemas.microsoft.com/winfx/2006/xaml/presentation\" xmlns:pw=\"clr-namespace:Ptc.Wpf;assembly=Ptc.Core\">N<pw:Subscript>SedManifoldPorts</pw:Subscript></Span></ml:id><ml:result /></ml:eval></math></region><region top=\"8544.721\" width=\"130\" left=\"345.6\" height=\"22\" converted-from=\"Mathcad14\" region-id=\"254\"><math><ml:eval><ml:id xml:space=\"preserve\"><Span xmlns=\"http://schemas.microsoft.com/winfx/2006/xaml/presentation\" xmlns:pw=\"clr-namespace:Ptc.Wpf;assembly=Ptc.Core\">L<pw:Subscript>SedManifoldPipe</pw:Subscript></Span></ml:id><ml:result /></ml:eval></math></region><region top=\"8621.52051\" width=\"128\" left=\"38.4\" height=\"53\" converted-from=\"Mathcad14\" region-id=\"255\"><math resultRef=\"-32\"><ml:eval><ml:id xml:space=\"preserve\"><Span xmlns=\"http://schemas.microsoft.com/winfx/2006/xaml/presentation\" xmlns:pw=\"clr-namespace:Ptc.Wpf;assembly=Ptc.Core\">ED<pw:Subscript>SedInlet</pw:Subscript></Span></ml:id><ml:result /></ml:eval></math></region><region top=\"8707.92\" width=\"131\" left=\"38.4\" height=\"22\" converted-from=\"Mathcad14\" region-id=\"256\"><math><ml:eval><ml:id xml:space=\"preserve\"><Span xmlns=\"http://schemas.microsoft.com/winfx/2006/xaml/presentation\" xmlns:pw=\"clr-namespace:Ptc.Wpf;assembly=Ptc.Core\">Q<pw:Subscript>SedManifoldPort</pw:Subscript></Span></ml:id><ml:result /></ml:eval></math></region><region top=\"8784.721\" width=\"119.36\" left=\"19.2\" height=\"19\" converted-from=\"Mathcad14\" region-id=\"257\"><text><FlowDocument FontFamily=\"Tahoma\" FontStyle=\"Normal\" FontWeight=\"Normal\" FontSize=\"14.6666666666667\" Foreground=\"#FF000000\" Background=\"#00FFFFFF\" PagePadding=\"5,0,5,0\" AllowDrop=\"True\" Typography.Variants=\"Normal\" xmlns=\"http://schemas.microsoft.com/winfx/2006/xaml/presentation\"><Paragraph TextAlignment=\"Left\"><Run FontFamily=\"Arial\" FontStyle=\"Normal\" FontWeight=\"Bold\" FontSize=\"16\" Foreground=\"#FF008000\" Typography.Variants=\"Normal\"><Run.TextDecorations><TextDecorationCollection /></Run.TextDecorations>Exit Channel:</Run></Paragraph></FlowDocument></text></region><region top=\"8813.52051\" width=\"128\" left=\"38.4\" height=\"22\" converted-from=\"Mathcad14\" region-id=\"258\"><math><ml:eval><ml:id xml:space=\"preserve\"><Span xmlns=\"http://schemas.microsoft.com/winfx/2006/xaml/presentation\" xmlns:pw=\"clr-namespace:Ptc.Wpf;assembly=Ptc.Core\">W<pw:Subscript>SedExitChannel</pw:Subscript></Span></ml:id><ml:result /></ml:eval></math></region><region top=\"8842.32\" width=\"124\" left=\"38.4\" height=\"22\" converted-from=\"Mathcad14\" region-id=\"259\"><math><ml:eval><ml:id xml:space=\"preserve\"><Span xmlns=\"http://schemas.microsoft.com/winfx/2006/xaml/presentation\" xmlns:pw=\"clr-namespace:Ptc.Wpf;assembly=Ptc.Core\">H<pw:Subscript>SedExitChannel</pw:Subscript></Span></ml:id><ml:result /></ml:eval></math></region><region top=\"8880.72\" width=\"137\" left=\"38.4\" height=\"22\" converted-from=\"Mathcad14\" region-id=\"260\"><math><ml:eval><ml:id xml:space=\"preserve\"><Span xmlns=\"http://schemas.microsoft.com/winfx/2006/xaml/presentation\" xmlns:pw=\"clr-namespace:Ptc.Wpf;assembly=Ptc.Core\">HW<pw:Subscript>SedExitChannel</pw:Subscript></Span></ml:id><ml:result /></ml:eval></math></region><region top=\"8890.319\" width=\"308.92\" left=\"259.2\" height=\"32\" converted-from=\"Mathcad14\" region-id=\"261\"><text><FlowDocument FontFamily=\"Tahoma\" FontStyle=\"Normal\" FontWeight=\"Normal\" FontSize=\"14.6666666666667\" Foreground=\"#FF000000\" Background=\"#00FFFFFF\" PagePadding=\"5,0,5,0\" AllowDrop=\"True\" Typography.Variants=\"Normal\" xmlns=\"http://schemas.microsoft.com/winfx/2006/xaml/presentation\"><Paragraph TextAlignment=\"Left\"><Run FontFamily=\"Arial\" FontStyle=\"Normal\" FontWeight=\"Normal\" FontSize=\"13.3333333333333\" Typography.Variants=\"Normal\"><Run.TextDecorations><TextDecorationCollection /></Run.TextDecorations>water height in exit channel from base of channel</Run></Paragraph></FlowDocument></text></region><region top=\"8928.72\" width=\"105\" left=\"38.4\" height=\"22\" converted-from=\"Mathcad14\" region-id=\"262\"><math><ml:eval><ml:id xml:space=\"preserve\"><Span xmlns=\"http://schemas.microsoft.com/winfx/2006/xaml/presentation\" xmlns:pw=\"clr-namespace:Ptc.Wpf;assembly=Ptc.Core\">H<pw:Subscript>SedWeirExit</pw:Subscript></Span></ml:id><ml:result /></ml:eval></math></region><region top=\"8986.319\" width=\"107\" left=\"19.2\" height=\"19\" converted-from=\"Mathcad14\" region-id=\"263\"><text><FlowDocument FontFamily=\"Tahoma\" FontStyle=\"Normal\" FontWeight=\"Normal\" FontSize=\"14.6666666666667\" Foreground=\"#FF000000\" Background=\"#00FFFFFF\" PagePadding=\"5,0,5,0\" AllowDrop=\"True\" Typography.Variants=\"Normal\" xmlns=\"http://schemas.microsoft.com/winfx/2006/xaml/presentation\"><Paragraph TextAlignment=\"Left\"><Run FontFamily=\"Arial\" FontStyle=\"Normal\" FontWeight=\"Bold\" FontSize=\"16\" Foreground=\"#FF008000\" Typography.Variants=\"Normal\"><Run.TextDecorations><TextDecorationCollection /></Run.TextDecorations>Lamella:</Run></Paragraph></FlowDocument></text></region><region top=\"9015.119\" width=\"84\" left=\"38.4\" height=\"22\" converted-from=\"Mathcad14\" region-id=\"264\"><math><ml:eval><ml:id xml:space=\"preserve\"><Span xmlns=\"http://schemas.microsoft.com/winfx/2006/xaml/presentation\" xmlns:pw=\"clr-namespace:Ptc.Wpf;assembly=Ptc.Core\">L<pw:Subscript>SedPlate</pw:Subscript></Span></ml:id><ml:result /></ml:eval></math></region><region top=\"9034.319\" width=\"264.28\" left=\"211.2\" height=\"16\" converted-from=\"Mathcad14\" region-id=\"265\"><text><FlowDocument FontFamily=\"Tahoma\" FontStyle=\"Normal\" FontWeight=\"Normal\" FontSize=\"14.6666666666667\" Foreground=\"#FF000000\" Background=\"#00FFFFFF\" PagePadding=\"5,0,5,0\" AllowDrop=\"True\" Typography.Variants=\"Normal\" xmlns=\"http://schemas.microsoft.com/winfx/2006/xaml/presentation\"><Paragraph TextAlignment=\"Left\"><Run FontFamily=\"Arial\" FontStyle=\"Normal\" FontWeight=\"Normal\" FontSize=\"13.3333333333333\" Typography.Variants=\"Normal\"><Run.TextDecorations><TextDecorationCollection /></Run.TextDecorations>center to center distance between lamella</Run></Paragraph></FlowDocument></text></region><region top=\"9043.92\" width=\"85\" left=\"38.4\" height=\"22\" converted-from=\"Mathcad14\" region-id=\"266\"><math><ml:eval><ml:id xml:space=\"preserve\"><Span xmlns=\"http://schemas.microsoft.com/winfx/2006/xaml/presentation\" xmlns:pw=\"clr-namespace:Ptc.Wpf;assembly=Ptc.Core\">B<pw:Subscript>SedPlate</pw:Subscript></Span></ml:id><ml:result /></ml:eval></math></region><region top=\"9063.119\" width=\"163.04\" left=\"211.2\" height=\"16\" converted-from=\"Mathcad14\" region-id=\"267\"><text><FlowDocument FontFamily=\"Tahoma\" FontStyle=\"Normal\" FontWeight=\"Normal\" FontSize=\"14.6666666666667\" Foreground=\"#FF000000\" Background=\"#00FFFFFF\" PagePadding=\"5,0,5,0\" AllowDrop=\"True\" Typography.Variants=\"Normal\" xmlns=\"http://schemas.microsoft.com/winfx/2006/xaml/presentation\"><Paragraph TextAlignment=\"Left\"><Run FontFamily=\"Arial\" FontStyle=\"Normal\" FontWeight=\"Normal\" FontSize=\"13.3333333333333\" Typography.Variants=\"Normal\"><Run.TextDecorations><TextDecorationCollection /></Run.TextDecorations>spacing between lamella</Run></Paragraph></FlowDocument></text></region><region top=\"9072.72\" width=\"116\" left=\"38.4\" height=\"22\" converted-from=\"Mathcad14\" region-id=\"268\"><math resultRef=\"-33\"><ml:eval><ml:id xml:space=\"preserve\"><Span xmlns=\"http://schemas.microsoft.com/winfx/2006/xaml/presentation\" xmlns:pw=\"clr-namespace:Ptc.Wpf;assembly=Ptc.Core\">S<pw:Subscript>SedPlate</pw:Subscript></Span></ml:id><ml:result /></ml:eval></math></region><region top=\"9111.119\" width=\"93\" left=\"38.4\" height=\"22\" converted-from=\"Mathcad14\" region-id=\"269\"><math><ml:eval><ml:id xml:space=\"preserve\"><Span xmlns=\"http://schemas.microsoft.com/winfx/2006/xaml/presentation\" xmlns:pw=\"clr-namespace:Ptc.Wpf;assembly=Ptc.Core\">N<pw:Subscript>SedPlates</pw:Subscript></Span></ml:id><ml:result /></ml:eval></math></region><region top=\"9111.119\" width=\"320.94\" left=\"211.2\" height=\"16\" converted-from=\"Mathcad14\" region-id=\"270\"><text><FlowDocument FontFamily=\"Tahoma\" FontStyle=\"Normal\" FontWeight=\"Normal\" FontSize=\"14.6666666666667\" Foreground=\"#FF000000\" Background=\"#00FFFFFF\" PagePadding=\"5,0,5,0\" AllowDrop=\"True\" Typography.Variants=\"Normal\" xmlns=\"http://schemas.microsoft.com/winfx/2006/xaml/presentation\"><Paragraph TextAlignment=\"Left\"><Run FontFamily=\"Arial\" FontStyle=\"Normal\" FontWeight=\"Normal\" FontSize=\"13.3333333333333\" Typography.Variants=\"Normal\"><Run.TextDecorations><TextDecorationCollection /></Run.TextDecorations>Number of Sed Plates per Sedimentation Tank Bay.</Run></Paragraph></FlowDocument></text></region><region top=\"9149.52\" width=\"109\" left=\"48\" height=\"22\" converted-from=\"Mathcad14\" region-id=\"271\"><math><ml:eval><ml:id xml:space=\"preserve\"><Span xmlns=\"http://schemas.microsoft.com/winfx/2006/xaml/presentation\" xmlns:pw=\"clr-namespace:Ptc.Wpf;assembly=Ptc.Core\">N<pw:Subscript>SedModules</pw:Subscript></Span></ml:id><ml:result /></ml:eval></math></region><region top=\"9149.52\" width=\"182.08\" left=\"230.4\" height=\"16\" converted-from=\"Mathcad14\" region-id=\"272\"><text><FlowDocument FontFamily=\"Tahoma\" FontStyle=\"Normal\" FontWeight=\"Normal\" FontSize=\"14.6666666666667\" Foreground=\"#FF000000\" Background=\"#00FFFFFF\" PagePadding=\"5,0,5,0\" AllowDrop=\"True\" Typography.Variants=\"Normal\" xmlns=\"http://schemas.microsoft.com/winfx/2006/xaml/presentation\"><Paragraph TextAlignment=\"Left\"><Run FontFamily=\"Arial\" FontStyle=\"Normal\" FontWeight=\"Normal\" FontSize=\"13.3333333333333\" Typography.Variants=\"Normal\"><Run.TextDecorations><TextDecorationCollection /></Run.TextDecorations>Number of modules per bay</Run></Paragraph></FlowDocument></text></region><region top=\"9197.52\" width=\"135\" left=\"48\" height=\"22\" converted-from=\"Mathcad14\" region-id=\"273\"><math><ml:eval><ml:id xml:space=\"preserve\"><Span xmlns=\"http://schemas.microsoft.com/winfx/2006/xaml/presentation\" xmlns:pw=\"clr-namespace:Ptc.Wpf;assembly=Ptc.Core\">N<pw:Subscript>SedModulePlates</pw:Subscript></Span></ml:id><ml:result /></ml:eval></math></region><region top=\"9197.52\" width=\"189.92\" left=\"230.4\" height=\"16\" converted-from=\"Mathcad14\" region-id=\"274\"><text><FlowDocument FontFamily=\"Tahoma\" FontStyle=\"Normal\" FontWeight=\"Normal\" FontSize=\"14.6666666666667\" Foreground=\"#FF000000\" Background=\"#00FFFFFF\" PagePadding=\"5,0,5,0\" AllowDrop=\"True\" Typography.Variants=\"Normal\" xmlns=\"http://schemas.microsoft.com/winfx/2006/xaml/presentation\"><Paragraph TextAlignment=\"Left\"><Run FontFamily=\"Arial\" FontStyle=\"Normal\" FontWeight=\"Normal\" FontSize=\"13.3333333333333\" Typography.Variants=\"Normal\"><Run.TextDecorations><TextDecorationCollection /></Run.TextDecorations>Number of plates per module</Run></Paragraph></FlowDocument></text></region><region top=\"9255.119\" width=\"117\" left=\"48\" height=\"22\" converted-from=\"Mathcad14\" region-id=\"275\"><math resultRef=\"-34\"><ml:eval><ml:id xml:space=\"preserve\"><Span xmlns=\"http://schemas.microsoft.com/winfx/2006/xaml/presentation\" xmlns:pw=\"clr-namespace:Ptc.Wpf;assembly=Ptc.Core\">AN<pw:Subscript>SedPlate</pw:Subscript></Span></ml:id><ml:result /></ml:eval></math></region><region top=\"9293.52\" width=\"94\" left=\"230.4\" height=\"22\" converted-from=\"Mathcad14\" region-id=\"276\"><math><ml:eval><ml:id xml:space=\"preserve\"><Span xmlns=\"http://schemas.microsoft.com/winfx/2006/xaml/presentation\" xmlns:pw=\"clr-namespace:Ptc.Wpf;assembly=Ptc.Core\">L<pw:Subscript>SedActive</pw:Subscript></Span></ml:id><ml:result /></ml:eval></math></region><region top=\"9341.52\" width=\"104\" left=\"230.4\" height=\"22\" converted-from=\"Mathcad14\" region-id=\"277\"><math><ml:eval><ml:id xml:space=\"preserve\"><Span xmlns=\"http://schemas.microsoft.com/winfx/2006/xaml/presentation\" xmlns:pw=\"clr-namespace:Ptc.Wpf;assembly=Ptc.Core\">Z<pw:Subscript>SedLaunder</pw:Subscript></Span></ml:id><ml:result /></ml:eval></math></region><region top=\"9399.119\" width=\"74\" left=\"38.4\" height=\"22\" converted-from=\"Mathcad14\" region-id=\"278\"><math><ml:eval><ml:id xml:space=\"preserve\"><Span xmlns=\"http://schemas.microsoft.com/winfx/2006/xaml/presentation\" xmlns:pw=\"clr-namespace:Ptc.Wpf;assembly=Ptc.Core\">HW<pw:Subscript>Sed</pw:Subscript></Span></ml:id><ml:result /></ml:eval></math></region><region top=\"9437.52\" width=\"61\" left=\"38.4\" height=\"22\" converted-from=\"Mathcad14\" region-id=\"279\"><math><ml:eval><ml:id xml:space=\"preserve\"><Span xmlns=\"http://schemas.microsoft.com/winfx/2006/xaml/presentation\" xmlns:pw=\"clr-namespace:Ptc.Wpf;assembly=Ptc.Core\">H<pw:Subscript>Sed</pw:Subscript></Span></ml:id><ml:result /></ml:eval></math></region><region top=\"9527.52051\" width=\"832\" left=\"0\" height=\"19.2\" region-id=\"280\"><text is-text-block=\"true\"><FlowDocument FontFamily=\"Mathcad UniMath\" xmlns=\"http://schemas.microsoft.com/winfx/2006/xaml/presentation\"><Paragraph xml:space=\"preserve\">---↑  ---</Paragraph></FlowDocument></text></region><region top=\"9656.16\" width=\"129\" left=\"9.6\" height=\"19\" converted-from=\"Mathcad14\" region-id=\"281\"><text><FlowDocument FontFamily=\"Tahoma\" FontStyle=\"Normal\" FontWeight=\"Normal\" FontSize=\"14.6666666666667\" Foreground=\"#FF000000\" Background=\"#00FFFFFF\" PagePadding=\"5,0,5,0\" AllowDrop=\"True\" Typography.Variants=\"Normal\" xmlns=\"http://schemas.microsoft.com/winfx/2006/xaml/presentation\"><Paragraph Margin=\"0,0,0,0\" TextAlignment=\"Left\"><Run FontFamily=\"Arial\" FontStyle=\"Normal\" FontWeight=\"Bold\" FontSize=\"16\" Foreground=\"#FF008000\" Typography.Variants=\"Normal\"><Run.TextDecorations><TextDecorationCollection /></Run.TextDecorations>SRSF</Run></Paragraph></FlowDocument></text></region><region top=\"9675.36\" width=\"832\" left=\"0\" height=\"19.2\" region-id=\"282\"><text is-text-block=\"true\"><FlowDocument FontFamily=\"Mathcad UniMath\" xmlns=\"http://schemas.microsoft.com/winfx/2006/xaml/presentation\"><Paragraph xml:space=\"preserve\">---↓  ---</Paragraph></FlowDocument></text><mc14-conversion-loss-annotations><annotation>CollapsedArea</annotation></mc14-conversion-loss-annotations></region><region top=\"9804\" width=\"50\" left=\"48\" height=\"22\" converted-from=\"Mathcad14\" region-id=\"283\"><math><ml:eval><ml:id xml:space=\"preserve\"><Span xmlns=\"http://schemas.microsoft.com/winfx/2006/xaml/presentation\" xmlns:pw=\"clr-namespace:Ptc.Wpf;assembly=Ptc.Core\">H<pw:Subscript>Fi</pw:Subscript></Span></ml:id><ml:result /></ml:eval></math></region><region top=\"9832.8\" width=\"48\" left=\"48\" height=\"22\" converted-from=\"Mathcad14\" region-id=\"284\"><math><ml:eval><ml:id xml:space=\"preserve\"><Span xmlns=\"http://schemas.microsoft.com/winfx/2006/xaml/presentation\" xmlns:pw=\"clr-namespace:Ptc.Wpf;assembly=Ptc.Core\">L<pw:Subscript>Fi</pw:Subscript></Span></ml:id><ml:result /></ml:eval></math></region><region top=\"9861.6\" width=\"54\" left=\"48\" height=\"22\" converted-from=\"Mathcad14\" region-id=\"285\"><math><ml:eval><ml:id xml:space=\"preserve\"><Span xmlns=\"http://schemas.microsoft.com/winfx/2006/xaml/presentation\" xmlns:pw=\"clr-namespace:Ptc.Wpf;assembly=Ptc.Core\">W<pw:Subscript>Fi</pw:Subscript></Span></ml:id><ml:result /></ml:eval></math></region><region top=\"9890.4\" width=\"157\" left=\"48\" height=\"22\" converted-from=\"Mathcad14\" region-id=\"286\"><math resultRef=\"-35\"><ml:eval><ml:id xml:space=\"preserve\"><Span xmlns=\"http://schemas.microsoft.com/winfx/2006/xaml/presentation\" xmlns:pw=\"clr-namespace:Ptc.Wpf;assembly=Ptc.Core\">B<pw:Subscript>FiManifoldBranch</pw:Subscript></Span></ml:id><ml:result /></ml:eval></math></region><region top=\"9948\" width=\"93\" left=\"48\" height=\"22\" converted-from=\"Mathcad14\" region-id=\"287\"><math><ml:eval><ml:id xml:space=\"preserve\"><Span xmlns=\"http://schemas.microsoft.com/winfx/2006/xaml/presentation\" xmlns:pw=\"clr-namespace:Ptc.Wpf;assembly=Ptc.Core\">ND<pw:Subscript>FiTrunk</pw:Subscript></Span></ml:id><ml:result /></ml:eval></math></region><region top=\"9986.4\" width=\"156\" left=\"48\" height=\"22\" converted-from=\"Mathcad14\" region-id=\"288\"><math resultRef=\"-36\"><ml:eval><ml:id xml:space=\"preserve\"><Span xmlns=\"http://schemas.microsoft.com/winfx/2006/xaml/presentation\" xmlns:pw=\"clr-namespace:Ptc.Wpf;assembly=Ptc.Core\">ND<pw:Subscript>FiManBranch</pw:Subscript></Span></ml:id><ml:result /></ml:eval></math></region><region top=\"10053.6\" width=\"110\" left=\"48\" height=\"22\" converted-from=\"Mathcad14\" region-id=\"289\"><math><ml:eval><ml:id xml:space=\"preserve\"><Span xmlns=\"http://schemas.microsoft.com/winfx/2006/xaml/presentation\" xmlns:pw=\"clr-namespace:Ptc.Wpf;assembly=Ptc.Core\">ND<pw:Subscript>FiBwTrunk</pw:Subscript></Span></ml:id><ml:result /></ml:eval></math></region><region top=\"10082.4\" width=\"141\" left=\"48\" height=\"22\" converted-from=\"Mathcad14\" region-id=\"290\"><math><ml:eval><ml:id xml:space=\"preserve\"><Span xmlns=\"http://schemas.microsoft.com/winfx/2006/xaml/presentation\" xmlns:pw=\"clr-namespace:Ptc.Wpf;assembly=Ptc.Core\">ND<pw:Subscript>FiBwManBranch</pw:Subscript></Span></ml:id><ml:result /></ml:eval></math></region><region top=\"10120.8\" width=\"114\" left=\"48\" height=\"22\" converted-from=\"Mathcad14\" region-id=\"291\"><math><ml:eval><ml:id xml:space=\"preserve\"><Span xmlns=\"http://schemas.microsoft.com/winfx/2006/xaml/presentation\" xmlns:pw=\"clr-namespace:Ptc.Wpf;assembly=Ptc.Core\">ND<pw:Subscript>FiExitWaste</pw:Subscript></Span></ml:id><ml:result /></ml:eval></math></region><region top=\"10159.2\" width=\"132\" left=\"48\" height=\"22\" converted-from=\"Mathcad14\" region-id=\"292\"><math><ml:eval><ml:id xml:space=\"preserve\"><Span xmlns=\"http://schemas.microsoft.com/winfx/2006/xaml/presentation\" xmlns:pw=\"clr-namespace:Ptc.Wpf;assembly=Ptc.Core\">ND<pw:Subscript>FiBwWeirDrain</pw:Subscript></Span></ml:id><ml:result /></ml:eval></math></region><region top=\"10188\" width=\"388.12\" left=\"278.4\" height=\"32\" converted-from=\"Mathcad14\" region-id=\"293\"><text><FlowDocument FontFamily=\"Tahoma\" FontStyle=\"Normal\" FontWeight=\"Normal\" FontSize=\"14.6666666666667\" Foreground=\"#FF000000\" Background=\"#00FFFFFF\" PagePadding=\"5,0,5,0\" AllowDrop=\"True\" Typography.Variants=\"Normal\" xmlns=\"http://schemas.microsoft.com/winfx/2006/xaml/presentation\"><Paragraph TextAlignment=\"Left\"><Run FontFamily=\"Arial\" FontStyle=\"Normal\" FontWeight=\"Normal\" FontSize=\"13.3333333333333\" Typography.Variants=\"Normal\"><Run.TextDecorations><TextDecorationCollection /></Run.TextDecorations>For the box that holds keeps the end of the siphon submerged</Run></Paragraph></FlowDocument></text></region><region top=\"10197.6\" width=\"106\" left=\"48\" height=\"22\" converted-from=\"Mathcad14\" region-id=\"294\"><math><ml:eval><ml:id xml:space=\"preserve\"><Span xmlns=\"http://schemas.microsoft.com/winfx/2006/xaml/presentation\" xmlns:pw=\"clr-namespace:Ptc.Wpf;assembly=Ptc.Core\">ND<pw:Subscript>FiBwDrain</pw:Subscript></Span></ml:id><ml:result /></ml:eval></math></region><region top=\"10236\" width=\"152\" left=\"48\" height=\"22\" converted-from=\"Mathcad14\" region-id=\"295\"><math resultRef=\"-37\"><ml:eval><ml:id xml:space=\"preserve\"><Span xmlns=\"http://schemas.microsoft.com/winfx/2006/xaml/presentation\" xmlns:pw=\"clr-namespace:Ptc.Wpf;assembly=Ptc.Core\">ND<pw:Subscript>FiSandOutlet</pw:Subscript></Span></ml:id><ml:result /></ml:eval></math></region><region top=\"10264.8\" width=\"338.96\" left=\"259.2\" height=\"16\" converted-from=\"Mathcad14\" region-id=\"296\"><text><FlowDocument FontFamily=\"Tahoma\" FontStyle=\"Normal\" FontWeight=\"Normal\" FontSize=\"14.6666666666667\" Foreground=\"#FF000000\" Background=\"#00FFFFFF\" PagePadding=\"5,0,5,0\" AllowDrop=\"True\" Typography.Variants=\"Normal\" xmlns=\"http://schemas.microsoft.com/winfx/2006/xaml/presentation\"><Paragraph TextAlignment=\"Left\"><Run FontFamily=\"Arial\" FontStyle=\"Normal\" FontWeight=\"Normal\" FontSize=\"13.3333333333333\" Typography.Variants=\"Normal\"><Run.TextDecorations><TextDecorationCollection /></Run.TextDecorations>This is the time required to empty the filter of the sand.</Run></Paragraph></FlowDocument></text></region><region top=\"10274.4\" width=\"80\" left=\"48\" height=\"22\" converted-from=\"Mathcad14\" region-id=\"297\"><math><ml:eval><ml:id xml:space=\"preserve\"><Span xmlns=\"http://schemas.microsoft.com/winfx/2006/xaml/presentation\" xmlns:pw=\"clr-namespace:Ptc.Wpf;assembly=Ptc.Core\">Ti<pw:Subscript>FiSand</pw:Subscript></Span></ml:id><ml:result /></ml:eval></math></region><region top=\"10322.4\" width=\"145\" left=\"48\" height=\"22\" converted-from=\"Mathcad14\" region-id=\"298\"><math><ml:eval><ml:id xml:space=\"preserve\"><Span xmlns=\"http://schemas.microsoft.com/winfx/2006/xaml/presentation\" xmlns:pw=\"clr-namespace:Ptc.Wpf;assembly=Ptc.Core\">ND<pw:Subscript>FiSiphonAirValve</pw:Subscript></Span></ml:id><ml:result /></ml:eval></math></region><region top=\"10370.4\" width=\"98\" left=\"48\" height=\"22\" converted-from=\"Mathcad14\" region-id=\"299\"><math><ml:eval><ml:id xml:space=\"preserve\"><Span xmlns=\"http://schemas.microsoft.com/winfx/2006/xaml/presentation\" xmlns:pw=\"clr-namespace:Ptc.Wpf;assembly=Ptc.Core\">ND<pw:Subscript>FiSiphon</pw:Subscript></Span></ml:id><ml:result /></ml:eval></math></region><region top=\"10418.4\" width=\"111\" left=\"48\" height=\"22\" converted-from=\"Mathcad14\" region-id=\"300\"><math><ml:eval><ml:id xml:space=\"preserve\"><Span xmlns=\"http://schemas.microsoft.com/winfx/2006/xaml/presentation\" xmlns:pw=\"clr-namespace:Ptc.Wpf;assembly=Ptc.Core\">Q<pw:Subscript>FiSiphonMax</pw:Subscript></Span></ml:id><ml:result /></ml:eval></math></region><region top=\"10476\" width=\"153\" left=\"48\" height=\"22\" converted-from=\"Mathcad14\" region-id=\"301\"><math><ml:eval><ml:id xml:space=\"preserve\"><Span xmlns=\"http://schemas.microsoft.com/winfx/2006/xaml/presentation\" xmlns:pw=\"clr-namespace:Ptc.Wpf;assembly=Ptc.Core\">B<pw:Subscript>FiSiphonManOrifices</pw:Subscript></Span></ml:id><ml:result /></ml:eval></math></region><region top=\"10514.4\" width=\"155\" left=\"48\" height=\"22\" converted-from=\"Mathcad14\" region-id=\"302\"><math><ml:eval><ml:id xml:space=\"preserve\"><Span xmlns=\"http://schemas.microsoft.com/winfx/2006/xaml/presentation\" xmlns:pw=\"clr-namespace:Ptc.Wpf;assembly=Ptc.Core\">N<pw:Subscript>FiSiphonManOrifices</pw:Subscript></Span></ml:id><ml:result /></ml:eval></math></region><region top=\"10552.8\" width=\"154\" left=\"48\" height=\"22\" converted-from=\"Mathcad14\" region-id=\"303\"><math><ml:eval><ml:id xml:space=\"preserve\"><Span xmlns=\"http://schemas.microsoft.com/winfx/2006/xaml/presentation\" xmlns:pw=\"clr-namespace:Ptc.Wpf;assembly=Ptc.Core\">D<pw:Subscript>FiSiphonManOrifices</pw:Subscript></Span></ml:id><ml:result /></ml:eval></math></region><region top=\"10591.2\" width=\"117\" left=\"48\" height=\"22\" converted-from=\"Mathcad14\" region-id=\"304\"><math><ml:eval><ml:id xml:space=\"preserve\"><Span xmlns=\"http://schemas.microsoft.com/winfx/2006/xaml/presentation\" xmlns:pw=\"clr-namespace:Ptc.Wpf;assembly=Ptc.Core\">Ti<pw:Subscript>FiBwInitiation</pw:Subscript></Span></ml:id><ml:result /></ml:eval></math></region><region top=\"10639.2\" width=\"78\" left=\"48\" height=\"22\" converted-from=\"Mathcad14\" region-id=\"305\"><math><ml:eval><ml:id xml:space=\"preserve\"><Span xmlns=\"http://schemas.microsoft.com/winfx/2006/xaml/presentation\" xmlns:pw=\"clr-namespace:Ptc.Wpf;assembly=Ptc.Core\">H<pw:Subscript>FiSand</pw:Subscript></Span></ml:id><ml:result /></ml:eval></math></region><region top=\"10677.6\" width=\"82\" left=\"48\" height=\"22\" converted-from=\"Mathcad14\" region-id=\"306\"><math resultRef=\"-38\"><ml:eval><ml:id xml:space=\"preserve\"><Span xmlns=\"http://schemas.microsoft.com/winfx/2006/xaml/presentation\" xmlns:pw=\"clr-namespace:Ptc.Wpf;assembly=Ptc.Core\">N<pw:Subscript>FiLayer</pw:Subscript></Span></ml:id><ml:result /></ml:eval></math></region><region top=\"10706.4\" width=\"81\" left=\"48\" height=\"22\" converted-from=\"Mathcad14\" region-id=\"307\"><math><ml:eval><ml:id xml:space=\"preserve\"><Span xmlns=\"http://schemas.microsoft.com/winfx/2006/xaml/presentation\" xmlns:pw=\"clr-namespace:Ptc.Wpf;assembly=Ptc.Core\">H<pw:Subscript>FiLayer</pw:Subscript></Span></ml:id><ml:result /></ml:eval></math></region><region top=\"10716\" width=\"159\" left=\"355.2\" height=\"37\" converted-from=\"Mathcad14\" region-id=\"308\"><math resultRef=\"-39\"><ml:eval><ml:id xml:space=\"preserve\"><Span xmlns=\"http://schemas.microsoft.com/winfx/2006/xaml/presentation\" xmlns:pw=\"clr-namespace:Ptc.Wpf;assembly=Ptc.Core\">V<pw:Subscript>FiLayer</pw:Subscript></Span></ml:id><ml:result /></ml:eval></math></region><region top=\"10754.4\" width=\"104\" left=\"48\" height=\"22\" converted-from=\"Mathcad14\" region-id=\"309\"><math><ml:eval><ml:id xml:space=\"preserve\"><Span xmlns=\"http://schemas.microsoft.com/winfx/2006/xaml/presentation\" xmlns:pw=\"clr-namespace:Ptc.Wpf;assembly=Ptc.Core\">HL<pw:Subscript>FiTerminal</pw:Subscript></Span></ml:id><ml:result /></ml:eval></math></region><region top=\"10764\" width=\"102\" left=\"355.2\" height=\"37\" converted-from=\"Mathcad14\" region-id=\"310\"><math resultRef=\"-40\"><ml:eval><ml:id xml:space=\"preserve\"><Span xmlns=\"http://schemas.microsoft.com/winfx/2006/xaml/presentation\" xmlns:pw=\"clr-namespace:Ptc.Wpf;assembly=Ptc.Core\">V<pw:Subscript>FiBw</pw:Subscript></Span></ml:id><ml:result /></ml:eval></math></region><region top=\"10792.8\" width=\"122\" left=\"48\" height=\"22\" converted-from=\"Mathcad14\" region-id=\"311\"><math><ml:eval><ml:id xml:space=\"preserve\"><Span xmlns=\"http://schemas.microsoft.com/winfx/2006/xaml/presentation\" xmlns:pw=\"clr-namespace:Ptc.Wpf;assembly=Ptc.Core\">HL<pw:Subscript>FiBwInitiation</pw:Subscript></Span></ml:id><ml:result /></ml:eval></math></region><region top=\"10831.2\" width=\"88\" left=\"48\" height=\"22\" converted-from=\"Mathcad14\" region-id=\"312\"><math><ml:eval><ml:id xml:space=\"preserve\"><Span xmlns=\"http://schemas.microsoft.com/winfx/2006/xaml/presentation\" xmlns:pw=\"clr-namespace:Ptc.Wpf;assembly=Ptc.Core\">HL<pw:Subscript>FiBwSS</pw:Subscript></Span></ml:id><ml:result /></ml:eval></math></region><region top=\"10831.2\" width=\"78\" left=\"364.8\" height=\"22\" converted-from=\"Mathcad14\" region-id=\"313\"><math><ml:eval><ml:id xml:space=\"preserve\"><Span xmlns=\"http://schemas.microsoft.com/winfx/2006/xaml/presentation\" xmlns:pw=\"clr-namespace:Ptc.Wpf;assembly=Ptc.Core\">D<pw:Subscript>FiSand</pw:Subscript></Span></ml:id><ml:result /></ml:eval></math></region><region top=\"10869.6\" width=\"51\" left=\"48\" height=\"22\" converted-from=\"Mathcad14\" region-id=\"314\"><math><ml:eval><ml:id xml:space=\"preserve\"><Span xmlns=\"http://schemas.microsoft.com/winfx/2006/xaml/presentation\" xmlns:pw=\"clr-namespace:Ptc.Wpf;assembly=Ptc.Core\">N<pw:Subscript>Fi</pw:Subscript></Span></ml:id><ml:result /></ml:eval></math></region><region top=\"10965.6\" width=\"50\" left=\"48\" height=\"22\" converted-from=\"Mathcad14\" region-id=\"315\"><math><ml:eval><ml:id xml:space=\"preserve\"><Span xmlns=\"http://schemas.microsoft.com/winfx/2006/xaml/presentation\" xmlns:pw=\"clr-namespace:Ptc.Wpf;assembly=Ptc.Core\">Q<pw:Subscript>Fi</pw:Subscript></Span></ml:id><ml:result /></ml:eval></math></region><region top=\"11023.2\" width=\"146\" left=\"48\" height=\"30\" converted-from=\"Mathcad14\" region-id=\"316\"><math resultRef=\"-41\"><ml:eval><ml:id xml:space=\"preserve\"><Span xmlns=\"http://schemas.microsoft.com/winfx/2006/xaml/presentation\" xmlns:pw=\"clr-namespace:Ptc.Wpf;assembly=Ptc.Core\">W<pw:Subscript>Slots</pw:Subscript></Span></ml:id><ml:result /></ml:eval></math></region><region top=\"11061.6\" width=\"187\" left=\"48\" height=\"30\" converted-from=\"Mathcad14\" region-id=\"317\"><math resultRef=\"-42\"><ml:eval><ml:id xml:space=\"preserve\"><Span xmlns=\"http://schemas.microsoft.com/winfx/2006/xaml/presentation\" xmlns:pw=\"clr-namespace:Ptc.Wpf;assembly=Ptc.Core\">B<pw:Subscript>FiBwManSlot</pw:Subscript></Span></ml:id><ml:result /></ml:eval></math></region><region top=\"11090.4\" width=\"111\" left=\"48\" height=\"22\" converted-from=\"Mathcad14\" region-id=\"318\"><math><ml:eval><ml:id xml:space=\"preserve\"><Span xmlns=\"http://schemas.microsoft.com/winfx/2006/xaml/presentation\" xmlns:pw=\"clr-namespace:Ptc.Wpf;assembly=Ptc.Core\">L<pw:Subscript>FiBwManSlot</pw:Subscript></Span></ml:id><ml:result /></ml:eval></math></region><region top=\"11138.4\" width=\"170\" left=\"48\" height=\"30\" converted-from=\"Mathcad14\" region-id=\"319\"><math resultRef=\"-43\"><ml:eval><ml:id xml:space=\"preserve\"><Span xmlns=\"http://schemas.microsoft.com/winfx/2006/xaml/presentation\" xmlns:pw=\"clr-namespace:Ptc.Wpf;assembly=Ptc.Core\">B<pw:Subscript>FiManSlot</pw:Subscript></Span></ml:id><ml:result /></ml:eval></math></region><region top=\"11176.8\" width=\"94\" left=\"48\" height=\"22\" converted-from=\"Mathcad14\" region-id=\"320\"><math><ml:eval><ml:id xml:space=\"preserve\"><Span xmlns=\"http://schemas.microsoft.com/winfx/2006/xaml/presentation\" xmlns:pw=\"clr-namespace:Ptc.Wpf;assembly=Ptc.Core\">L<pw:Subscript>FiManSlot</pw:Subscript></Span></ml:id><ml:result /></ml:eval></math></region><region top=\"11215.2\" width=\"102\" left=\"48\" height=\"22\" converted-from=\"Mathcad14\" region-id=\"321\"><math resultRef=\"-44\"><ml:eval><ml:id xml:space=\"preserve\"><Span xmlns=\"http://schemas.microsoft.com/winfx/2006/xaml/presentation\" xmlns:pw=\"clr-namespace:Ptc.Wpf;assembly=Ptc.Core\">N<pw:Subscript>FiSlotRows</pw:Subscript></Span></ml:id><ml:result /></ml:eval></math></region><region top=\"11282.4\" width=\"88\" left=\"48\" height=\"22\" converted-from=\"Mathcad14\" region-id=\"322\"><math><ml:eval><ml:id xml:space=\"preserve\"><Span xmlns=\"http://schemas.microsoft.com/winfx/2006/xaml/presentation\" xmlns:pw=\"clr-namespace:Ptc.Wpf;assembly=Ptc.Core\">Z<pw:Subscript>FiBottom</pw:Subscript></Span></ml:id><ml:result /></ml:eval></math></region><region top=\"11330.4\" width=\"71\" left=\"48\" height=\"22\" converted-from=\"Mathcad14\" region-id=\"323\"><math><ml:eval><ml:id xml:space=\"preserve\"><Span xmlns=\"http://schemas.microsoft.com/winfx/2006/xaml/presentation\" xmlns:pw=\"clr-namespace:Ptc.Wpf;assembly=Ptc.Core\">Z<pw:Subscript>FiTop</pw:Subscript></Span></ml:id><ml:result /></ml:eval></math></region><region top=\"11368.8\" width=\"50.36\" left=\"48\" height=\"16\" converted-from=\"Mathcad14\" region-id=\"324\"><text><FlowDocument FontFamily=\"Tahoma\" FontStyle=\"Normal\" FontWeight=\"Normal\" FontSize=\"14.6666666666667\" Foreground=\"#FF000000\" Background=\"#00FFFFFF\" PagePadding=\"5,0,5,0\" AllowDrop=\"True\" Typography.Variants=\"Normal\" xmlns=\"http://schemas.microsoft.com/winfx/2006/xaml/presentation\"><Paragraph TextAlignment=\"Left\"><Run FontFamily=\"Arial\" FontStyle=\"Normal\" FontWeight=\"Normal\" FontSize=\"13.3333333333333\" Typography.Variants=\"Normal\" xml:space=\"preserve\"><Run.TextDecorations><TextDecorationCollection /></Run.TextDecorations>Weirs </Run></Paragraph></FlowDocument></text></region><region top=\"11388\" width=\"84\" left=\"48\" height=\"22\" converted-from=\"Mathcad14\" region-id=\"325\"><math><ml:eval><ml:id xml:space=\"preserve\"><Span xmlns=\"http://schemas.microsoft.com/winfx/2006/xaml/presentation\" xmlns:pw=\"clr-namespace:Ptc.Wpf;assembly=Ptc.Core\">HL<pw:Subscript>FiWeir</pw:Subscript></Span></ml:id><ml:result /></ml:eval></math></region><region top=\"11416.8\" width=\"75\" left=\"48\" height=\"22\" converted-from=\"Mathcad14\" region-id=\"326\"><math><ml:eval><ml:id xml:space=\"preserve\"><Span xmlns=\"http://schemas.microsoft.com/winfx/2006/xaml/presentation\" xmlns:pw=\"clr-namespace:Ptc.Wpf;assembly=Ptc.Core\">L<pw:Subscript>FiWeir</pw:Subscript></Span></ml:id><ml:result /></ml:eval></math></region><region top=\"11445.6\" width=\"123\" left=\"48\" height=\"22\" converted-from=\"Mathcad14\" region-id=\"327\"><math><ml:eval><ml:id xml:space=\"preserve\"><Span xmlns=\"http://schemas.microsoft.com/winfx/2006/xaml/presentation\" xmlns:pw=\"clr-namespace:Ptc.Wpf;assembly=Ptc.Core\">Z<pw:Subscript>FiEntranceWeir</pw:Subscript></Span></ml:id><ml:result /></ml:eval></math></region><region top=\"11484\" width=\"93\" left=\"48\" height=\"22\" converted-from=\"Mathcad14\" region-id=\"328\"><math><ml:eval><ml:id xml:space=\"preserve\"><Span xmlns=\"http://schemas.microsoft.com/winfx/2006/xaml/presentation\" xmlns:pw=\"clr-namespace:Ptc.Wpf;assembly=Ptc.Core\">Z<pw:Subscript>FiBwWeir</pw:Subscript></Span></ml:id><ml:result /></ml:eval></math></region><region top=\"11522.4\" width=\"324.76\" left=\"259.2\" height=\"16\" converted-from=\"Mathcad14\" region-id=\"329\"><text><FlowDocument FontFamily=\"Tahoma\" FontStyle=\"Normal\" FontWeight=\"Normal\" FontSize=\"14.6666666666667\" Foreground=\"#FF000000\" Background=\"#00FFFFFF\" PagePadding=\"5,0,5,0\" AllowDrop=\"True\" Typography.Variants=\"Normal\" xmlns=\"http://schemas.microsoft.com/winfx/2006/xaml/presentation\"><Paragraph TextAlignment=\"Left\"><Run FontFamily=\"Arial\" FontStyle=\"Normal\" FontWeight=\"Normal\" FontSize=\"13.3333333333333\" Typography.Variants=\"Normal\"><Run.TextDecorations><TextDecorationCollection /></Run.TextDecorations>This is the centerline elevation of the siphon orifices</Run></Paragraph></FlowDocument></text></region><region top=\"11532\" width=\"111\" left=\"48\" height=\"22\" converted-from=\"Mathcad14\" region-id=\"330\"><math><ml:eval><ml:id xml:space=\"preserve\"><Span xmlns=\"http://schemas.microsoft.com/winfx/2006/xaml/presentation\" xmlns:pw=\"clr-namespace:Ptc.Wpf;assembly=Ptc.Core\">Z<pw:Subscript>FiSiphonInlet</pw:Subscript></Span></ml:id><ml:result /></ml:eval></math></region><region top=\"11570.4\" width=\"95\" left=\"48\" height=\"22\" converted-from=\"Mathcad14\" region-id=\"331\"><math><ml:eval><ml:id xml:space=\"preserve\"><Span xmlns=\"http://schemas.microsoft.com/winfx/2006/xaml/presentation\" xmlns:pw=\"clr-namespace:Ptc.Wpf;assembly=Ptc.Core\">Z<pw:Subscript>FiExitWeir</pw:Subscript></Span></ml:id><ml:result /></ml:eval></math></region><region top=\"11599.2\" width=\"107\" left=\"48\" height=\"22\" converted-from=\"Mathcad14\" region-id=\"332\"><math><ml:eval><ml:id xml:space=\"preserve\"><Span xmlns=\"http://schemas.microsoft.com/winfx/2006/xaml/presentation\" xmlns:pw=\"clr-namespace:Ptc.Wpf;assembly=Ptc.Core\">Z<pw:Subscript>FiExitBottom</pw:Subscript></Span></ml:id><ml:result /></ml:eval></math></region><region top=\"11599.2\" width=\"199.8\" left=\"278.4\" height=\"16\" converted-from=\"Mathcad14\" region-id=\"333\"><text><FlowDocument FontFamily=\"Tahoma\" FontStyle=\"Normal\" FontWeight=\"Normal\" FontSize=\"14.6666666666667\" Foreground=\"#FF000000\" Background=\"#00FFFFFF\" PagePadding=\"5,0,5,0\" AllowDrop=\"True\" Typography.Variants=\"Normal\" xmlns=\"http://schemas.microsoft.com/winfx/2006/xaml/presentation\"><Paragraph TextAlignment=\"Left\"><Run FontFamily=\"Arial\" FontStyle=\"Normal\" FontWeight=\"Normal\" FontSize=\"13.3333333333333\" Typography.Variants=\"Normal\"><Run.TextDecorations><TextDecorationCollection /></Run.TextDecorations>bottom of the filtered water box</Run></Paragraph></FlowDocument></text></region><region top=\"11628\" width=\"135\" left=\"48\" height=\"22\" converted-from=\"Mathcad14\" region-id=\"334\"><math><ml:eval><ml:id xml:space=\"preserve\"><Span xmlns=\"http://schemas.microsoft.com/winfx/2006/xaml/presentation\" xmlns:pw=\"clr-namespace:Ptc.Wpf;assembly=Ptc.Core\">Z<pw:Subscript>FiEntranceBottom</pw:Subscript></Span></ml:id><ml:result /></ml:eval></math></region><region top=\"11628\" width=\"177.6\" left=\"288\" height=\"16\" converted-from=\"Mathcad14\" region-id=\"335\"><text><FlowDocument FontFamily=\"Tahoma\" FontStyle=\"Normal\" FontWeight=\"Normal\" FontSize=\"14.6666666666667\" Foreground=\"#FF000000\" Background=\"#00FFFFFF\" PagePadding=\"5,0,5,0\" AllowDrop=\"True\" Typography.Variants=\"Normal\" xmlns=\"http://schemas.microsoft.com/winfx/2006/xaml/presentation\"><Paragraph TextAlignment=\"Left\"><Run FontFamily=\"Arial\" FontStyle=\"Normal\" FontWeight=\"Normal\" FontSize=\"13.3333333333333\" Typography.Variants=\"Normal\"><Run.TextDecorations><TextDecorationCollection /></Run.TextDecorations>bottom of the entrance box</Run></Paragraph></FlowDocument></text></region><region top=\"11666.4\" width=\"136\" left=\"48\" height=\"22\" converted-from=\"Mathcad14\" region-id=\"336\"><math><ml:eval><ml:id xml:space=\"preserve\"><Span xmlns=\"http://schemas.microsoft.com/winfx/2006/xaml/presentation\" xmlns:pw=\"clr-namespace:Ptc.Wpf;assembly=Ptc.Core\">Z<pw:Subscript>FiSiphonCoupling</pw:Subscript></Span></ml:id><ml:result /></ml:eval></math></region><region top=\"11695.2\" width=\"88\" left=\"48\" height=\"22\" converted-from=\"Mathcad14\" region-id=\"337\"><math><ml:eval><ml:id xml:space=\"preserve\"><Span xmlns=\"http://schemas.microsoft.com/winfx/2006/xaml/presentation\" xmlns:pw=\"clr-namespace:Ptc.Wpf;assembly=Ptc.Core\">Z<pw:Subscript>FiBwTop</pw:Subscript></Span></ml:id><ml:result /></ml:eval></math></region><region top=\"11752.8\" width=\"100\" left=\"38.4\" height=\"22\" converted-from=\"Mathcad14\" region-id=\"338\"><math><ml:eval><ml:id xml:space=\"preserve\"><Span xmlns=\"http://schemas.microsoft.com/winfx/2006/xaml/presentation\" xmlns:pw=\"clr-namespace:Ptc.Wpf;assembly=Ptc.Core\">W<pw:Subscript>FiBwDrain</pw:Subscript></Span></ml:id><ml:result /></ml:eval></math></region><region top=\"11800.8\" width=\"96\" left=\"38.4\" height=\"22\" converted-from=\"Mathcad14\" region-id=\"339\"><math><ml:eval><ml:id xml:space=\"preserve\"><Span xmlns=\"http://schemas.microsoft.com/winfx/2006/xaml/presentation\" xmlns:pw=\"clr-namespace:Ptc.Wpf;assembly=Ptc.Core\">H<pw:Subscript>FiBwDrain</pw:Subscript></Span></ml:id><ml:result /></ml:eval></math></region><region top=\"12054\" width=\"832\" left=\"0\" height=\"19.2\" region-id=\"340\"><text is-text-block=\"true\"><FlowDocument FontFamily=\"Mathcad UniMath\" xmlns=\"http://schemas.microsoft.com/winfx/2006/xaml/presentation\"><Paragraph xml:space=\"preserve\">---↑  ---</Paragraph></FlowDocument></text></region><region top=\"12163.44\" width=\"832\" left=\"0\" height=\"19.2\" region-id=\"341\"><text is-text-block=\"true\"><FlowDocument FontFamily=\"Mathcad UniMath\" xmlns=\"http://schemas.microsoft.com/winfx/2006/xaml/presentation\"><Paragraph xml:space=\"preserve\">---↓  ---</Paragraph></FlowDocument></text><mc14-conversion-loss-annotations><annotation>CollapsedArea</annotation></mc14-conversion-loss-annotations></region><region top=\"12253.6807\" width=\"91\" left=\"76.8\" height=\"22\" converted-from=\"Mathcad14\" region-id=\"342\"><math><ml:eval><ml:id xml:space=\"preserve\"><Span xmlns=\"http://schemas.microsoft.com/winfx/2006/xaml/presentation\" xmlns:pw=\"clr-namespace:Ptc.Wpf;assembly=Ptc.Core\">N<pw:Subscript>Launders</pw:Subscript></Span></ml:id><ml:result /></ml:eval></math></region><region top=\"12282.48\" width=\"134\" left=\"76.8\" height=\"22\" converted-from=\"Mathcad14\" region-id=\"343\"><math><ml:eval><ml:id xml:space=\"preserve\"><Span xmlns=\"http://schemas.microsoft.com/winfx/2006/xaml/presentation\" xmlns:pw=\"clr-namespace:Ptc.Wpf;assembly=Ptc.Core\">L<pw:Subscript>LaunderPipeTotal</pw:Subscript></Span></ml:id><ml:result /></ml:eval></math></region><region top=\"12320.8809\" width=\"140\" left=\"76.8\" height=\"22\" converted-from=\"Mathcad14\" region-id=\"344\"><math><ml:eval><ml:id xml:space=\"preserve\"><Span xmlns=\"http://schemas.microsoft.com/winfx/2006/xaml/presentation\" xmlns:pw=\"clr-namespace:Ptc.Wpf;assembly=Ptc.Core\">N<pw:Subscript>LaunderCouplings</pw:Subscript></Span></ml:id><ml:result /></ml:eval></math></region><region top=\"12359.28\" width=\"126\" left=\"76.8\" height=\"22\" converted-from=\"Mathcad14\" region-id=\"345\"><math><ml:eval><ml:id xml:space=\"preserve\"><Span xmlns=\"http://schemas.microsoft.com/winfx/2006/xaml/presentation\" xmlns:pw=\"clr-namespace:Ptc.Wpf;assembly=Ptc.Core\">N<pw:Subscript>ValveCouplings</pw:Subscript></Span></ml:id><ml:result /></ml:eval></math></region><region top=\"12397.6807\" width=\"122\" left=\"76.8\" height=\"22\" converted-from=\"Mathcad14\" region-id=\"346\"><math><ml:eval><ml:id xml:space=\"preserve\"><Span xmlns=\"http://schemas.microsoft.com/winfx/2006/xaml/presentation\" xmlns:pw=\"clr-namespace:Ptc.Wpf;assembly=Ptc.Core\">N<pw:Subscript>SedPlatesTotal</pw:Subscript></Span></ml:id><ml:result /></ml:eval></math></region><region top=\"12426.48\" width=\"140\" left=\"76.8\" height=\"22\" converted-from=\"Mathcad14\" region-id=\"347\"><math><ml:eval><ml:id xml:space=\"preserve\"><Span xmlns=\"http://schemas.microsoft.com/winfx/2006/xaml/presentation\" xmlns:pw=\"clr-namespace:Ptc.Wpf;assembly=Ptc.Core\">N<pw:Subscript>SedPlatesPerSheet</pw:Subscript></Span></ml:id><ml:result /></ml:eval></math></region><region top=\"12464.8809\" width=\"123\" left=\"76.8\" height=\"22\" converted-from=\"Mathcad14\" region-id=\"348\"><math><ml:eval><ml:id xml:space=\"preserve\"><Span xmlns=\"http://schemas.microsoft.com/winfx/2006/xaml/presentation\" xmlns:pw=\"clr-namespace:Ptc.Wpf;assembly=Ptc.Core\">N<pw:Subscript>SedPlateSheets</pw:Subscript></Span></ml:id><ml:result /></ml:eval></math></region><region top=\"12512.8809\" width=\"77\" left=\"76.8\" height=\"22\" converted-from=\"Mathcad14\" region-id=\"349\"><math><ml:eval><ml:id xml:space=\"preserve\"><Span xmlns=\"http://schemas.microsoft.com/winfx/2006/xaml/presentation\" xmlns:pw=\"clr-namespace:Ptc.Wpf;assembly=Ptc.Core\">N<pw:Subscript>Valves</pw:Subscript></Span></ml:id><ml:result /></ml:eval></math></region><region top=\"12560.8809\" width=\"81\" left=\"76.8\" height=\"22\" converted-from=\"Mathcad14\" region-id=\"350\"><math><ml:eval><ml:id xml:space=\"preserve\"><Span xmlns=\"http://schemas.microsoft.com/winfx/2006/xaml/presentation\" xmlns:pw=\"clr-namespace:Ptc.Wpf;assembly=Ptc.Core\">A<pw:Subscript>EtFloor</pw:Subscript></Span></ml:id><ml:result /></ml:eval></math></region><region top=\"12608.8809\" width=\"125\" left=\"76.8\" height=\"22\" converted-from=\"Mathcad14\" region-id=\"351\"><math><ml:eval><ml:id xml:space=\"preserve\"><Span xmlns=\"http://schemas.microsoft.com/winfx/2006/xaml/presentation\" xmlns:pw=\"clr-namespace:Ptc.Wpf;assembly=Ptc.Core\">W<pw:Subscript>FlocWithWalls</pw:Subscript></Span></ml:id><ml:result /></ml:eval></math></region><region top=\"12637.6807\" width=\"119\" left=\"76.8\" height=\"22\" converted-from=\"Mathcad14\" region-id=\"352\"><math><ml:eval><ml:id xml:space=\"preserve\"><Span xmlns=\"http://schemas.microsoft.com/winfx/2006/xaml/presentation\" xmlns:pw=\"clr-namespace:Ptc.Wpf;assembly=Ptc.Core\">L<pw:Subscript>FlocWithWalls</pw:Subscript></Span></ml:id><ml:result /></ml:eval></math></region><region top=\"12676.08\" width=\"101\" left=\"76.8\" height=\"22\" converted-from=\"Mathcad14\" region-id=\"353\"><math><ml:eval><ml:id xml:space=\"preserve\"><Span xmlns=\"http://schemas.microsoft.com/winfx/2006/xaml/presentation\" xmlns:pw=\"clr-namespace:Ptc.Wpf;assembly=Ptc.Core\">Vol<pw:Subscript>FlocFloor</pw:Subscript></Span></ml:id><ml:result /></ml:eval></math></region><region top=\"12714.48\" width=\"93\" left=\"76.8\" height=\"22\" converted-from=\"Mathcad14\" region-id=\"354\"><math><ml:eval><ml:id xml:space=\"preserve\"><Span xmlns=\"http://schemas.microsoft.com/winfx/2006/xaml/presentation\" xmlns:pw=\"clr-namespace:Ptc.Wpf;assembly=Ptc.Core\">A<pw:Subscript>FlocFloor</pw:Subscript></Span></ml:id><ml:result /></ml:eval></math></region><region top=\"12762.48\" width=\"105\" left=\"76.8\" height=\"22\" converted-from=\"Mathcad14\" region-id=\"355\"><math><ml:eval><ml:id xml:space=\"preserve\"><Span xmlns=\"http://schemas.microsoft.com/winfx/2006/xaml/presentation\" xmlns:pw=\"clr-namespace:Ptc.Wpf;assembly=Ptc.Core\">Vol<pw:Subscript>SedSlopes</pw:Subscript></Span></ml:id><ml:result /></ml:eval></math></region><region top=\"12800.8809\" width=\"92\" left=\"76.8\" height=\"22\" converted-from=\"Mathcad14\" region-id=\"356\"><math><ml:eval><ml:id xml:space=\"preserve\"><Span xmlns=\"http://schemas.microsoft.com/winfx/2006/xaml/presentation\" xmlns:pw=\"clr-namespace:Ptc.Wpf;assembly=Ptc.Core\">A<pw:Subscript>SedWalls</pw:Subscript></Span></ml:id><ml:result /></ml:eval></math></region><region top=\"12839.28\" width=\"90\" left=\"76.8\" height=\"22\" converted-from=\"Mathcad14\" region-id=\"357\"><math><ml:eval><ml:id xml:space=\"preserve\"><Span xmlns=\"http://schemas.microsoft.com/winfx/2006/xaml/presentation\" xmlns:pw=\"clr-namespace:Ptc.Wpf;assembly=Ptc.Core\">A<pw:Subscript>SedFloor</pw:Subscript></Span></ml:id><ml:result /></ml:eval></math></region><region top=\"12881.28\" width=\"832\" left=\"0\" height=\"19.2\" region-id=\"358\"><text is-text-block=\"true\"><FlowDocument FontFamily=\"Mathcad UniMath\" xmlns=\"http://schemas.microsoft.com/winfx/2006/xaml/presentation\"><Paragraph xml:space=\"preserve\">---↑  ---</Paragraph></FlowDocument></text></region><region top=\"12904.32\" width=\"129\" left=\"9.6\" height=\"19\" converted-from=\"Mathcad14\" region-id=\"359\"><text><FlowDocument FontFamily=\"Tahoma\" FontStyle=\"Normal\" FontWeight=\"Normal\" FontSize=\"14.6666666666667\" Foreground=\"#FF000000\" Background=\"#00FFFFFF\" PagePadding=\"5,0,5,0\" AllowDrop=\"True\" Typography.Variants=\"Normal\" xmlns=\"http://schemas.microsoft.com/winfx/2006/xaml/presentation\"><Paragraph Margin=\"0,0,0,0\" TextAlignment=\"Left\"><Run FontFamily=\"Arial\" FontStyle=\"Normal\" FontWeight=\"Bold\" FontSize=\"16\" Foreground=\"#FF008000\" Typography.Variants=\"Normal\"><Run.TextDecorations><TextDecorationCollection /></Run.TextDecorations>Materials List</Run></Paragraph></FlowDocument></text></region><region top=\"13077.12\" width=\"239.32\" left=\"28.8\" height=\"19\" converted-from=\"Mathcad14\" region-id=\"360\"><text><FlowDocument FontFamily=\"Tahoma\" FontStyle=\"Normal\" FontWeight=\"Normal\" FontSize=\"14.6666666666667\" Foreground=\"#FF000000\" Background=\"#00FFFFFF\" PagePadding=\"5,0,5,0\" AllowDrop=\"True\" Typography.Variants=\"Normal\" xmlns=\"http://schemas.microsoft.com/winfx/2006/xaml/presentation\"><Paragraph Margin=\"0,0,0,0\" TextAlignment=\"Left\"><Run FontFamily=\"Arial\" FontStyle=\"Normal\" FontWeight=\"Bold\" FontSize=\"16\" Foreground=\"#FF008000\" Typography.Variants=\"Normal\"><Run.TextDecorations><TextDecorationCollection /></Run.TextDecorations>Plant Summary Calculations:</Run></Paragraph></FlowDocument></text></region><region top=\"13125.12\" width=\"320\" left=\"28.8\" height=\"22\" converted-from=\"Mathcad14\" region-id=\"361\"><math><ml:define><ml:id label=\"Variable\" xml:space=\"preserve\"><Span xmlns=\"http://schemas.microsoft.com/winfx/2006/xaml/presentation\" xmlns:pw=\"clr-namespace:Ptc.Wpf;assembly=Ptc.Core\">HL<pw:Subscript>PlantTotal</pw:Subscript></Span></ml:id><ml:apply><ml:minus /><ml:apply><ml:minus /><ml:id xml:space=\"preserve\"><Span xmlns=\"http://schemas.microsoft.com/winfx/2006/xaml/presentation\" xmlns:pw=\"clr-namespace:Ptc.Wpf;assembly=Ptc.Core\">Z<pw:Subscript>EtTop</pw:Subscript></Span></ml:id><ml:id xml:space=\"preserve\"><Span xmlns=\"http://schemas.microsoft.com/winfx/2006/xaml/presentation\" xmlns:pw=\"clr-namespace:Ptc.Wpf;assembly=Ptc.Core\">H<pw:Subscript>PlantFreeboard</pw:Subscript></Span></ml:id></ml:apply><ml:id xml:space=\"preserve\"><Span xmlns=\"http://schemas.microsoft.com/winfx/2006/xaml/presentation\" xmlns:pw=\"clr-namespace:Ptc.Wpf;assembly=Ptc.Core\">Z<pw:Subscript>FiExitWeir</pw:Subscript></Span></ml:id></ml:apply></ml:define></math></region><region top=\"13173.12\" width=\"103\" left=\"28.8\" height=\"22\" converted-from=\"Mathcad14\" region-id=\"362\"><math><ml:eval><ml:id xml:space=\"preserve\"><Span xmlns=\"http://schemas.microsoft.com/winfx/2006/xaml/presentation\" xmlns:pw=\"clr-namespace:Ptc.Wpf;assembly=Ptc.Core\">HL<pw:Subscript>PlantTotal</pw:Subscript></Span></ml:id><ml:result /></ml:eval></math></region><region top=\"13307.5205\" width=\"454.5\" left=\"9.6\" height=\"21\" converted-from=\"Mathcad14\" region-id=\"363\"><text><FlowDocument FontFamily=\"Tahoma\" FontStyle=\"Normal\" FontWeight=\"Normal\" FontSize=\"14.6666666666667\" Foreground=\"#FF000000\" Background=\"#00FFFFFF\" PagePadding=\"5,0,5,0\" AllowDrop=\"True\" Typography.Variants=\"Normal\" xmlns=\"http://schemas.microsoft.com/winfx/2006/xaml/presentation\"><Paragraph TextAlignment=\"Left\"><Run FontFamily=\"Arial\" FontStyle=\"Normal\" FontWeight=\"Bold\" FontSize=\"18.6666666666667\" Typography.Variants=\"Normal\"><Run.TextDecorations><TextDecorationCollection /></Run.TextDecorations>Make AC variables that are shorter than 598 lines</Run></Paragraph></FlowDocument></text></region><region top=\"13345.92\" width=\"832\" left=\"0\" height=\"19.2\" region-id=\"364\"><text is-text-block=\"true\"><FlowDocument FontFamily=\"Mathcad UniMath\" xmlns=\"http://schemas.microsoft.com/winfx/2006/xaml/presentation\"><Paragraph xml:space=\"preserve\">---↓  ---</Paragraph></FlowDocument></text><mc14-conversion-loss-annotations><annotation>CollapsedArea</annotation></mc14-conversion-loss-annotations></region><region top=\"13416.9609\" width=\"310\" left=\"67.2\" height=\"49\" converted-from=\"Mathcad14\" region-id=\"365\"><math><ml:define><ml:id label=\"Variable\" xml:space=\"preserve\"><Span xmlns=\"http://schemas.microsoft.com/winfx/2006/xaml/presentation\" xmlns:pw=\"clr-namespace:Ptc.Wpf;assembly=Ptc.Core\">AC<pw:Subscript>CdcA</pw:Subscript></Span></ml:id><ml:program><ml:if><ml:test><ml:apply><ml:lessThan /><ml:apply><ml:id xml:space=\"preserve\">last</ml:id><ml:id xml:space=\"preserve\"><Span xmlns=\"http://schemas.microsoft.com/winfx/2006/xaml/presentation\" xmlns:pw=\"clr-namespace:Ptc.Wpf;assembly=Ptc.Core\">AC<pw:Subscript>Cdc</pw:Subscript></Span></ml:id></ml:apply><ml:real>598</ml:real></ml:apply></ml:test><ml:then><ml:program><ml:id xml:space=\"preserve\"><Span xmlns=\"http://schemas.microsoft.com/winfx/2006/xaml/presentation\" xmlns:pw=\"clr-namespace:Ptc.Wpf;assembly=Ptc.Core\">AC<pw:Subscript>Cdc</pw:Subscript></Span></ml:id></ml:program></ml:then><ml:else><ml:program><ml:apply><ml:id xml:space=\"preserve\">submatrix</ml:id><ml:sequence><ml:id xml:space=\"preserve\"><Span xmlns=\"http://schemas.microsoft.com/winfx/2006/xaml/presentation\" xmlns:pw=\"clr-namespace:Ptc.Wpf;assembly=Ptc.Core\">AC<pw:Subscript>Cdc</pw:Subscript></Span></ml:id><ml:real>0</ml:real><ml:real>598</ml:real><ml:real>0</ml:real><ml:real>0</ml:real></ml:sequence></ml:apply></ml:program></ml:else></ml:if></ml:program></ml:define></math><mc14-conversion-loss-annotations><annotation>Otherwise</annotation></mc14-conversion-loss-annotations></region><region top=\"13493.7607\" width=\"441\" left=\"67.2\" height=\"49\" converted-from=\"Mathcad14\" region-id=\"366\"><math><ml:define><ml:id label=\"Variable\" xml:space=\"preserve\"><Span xmlns=\"http://schemas.microsoft.com/winfx/2006/xaml/presentation\" xmlns:pw=\"clr-namespace:Ptc.Wpf;assembly=Ptc.Core\">AC<pw:Subscript>CdcB</pw:Subscript></Span></ml:id><ml:program><ml:if><ml:test><ml:apply><ml:lessThan /><ml:apply><ml:id xml:space=\"preserve\">last</ml:id><ml:id xml:space=\"preserve\"><Span xmlns=\"http://schemas.microsoft.com/winfx/2006/xaml/presentation\" xmlns:pw=\"clr-namespace:Ptc.Wpf;assembly=Ptc.Core\">AC<pw:Subscript>Cdc</pw:Subscript></Span></ml:id></ml:apply><ml:real>1197</ml:real></ml:apply></ml:test><ml:then><ml:program><ml:apply><ml:id xml:space=\"preserve\">submatrix</ml:id><ml:sequence><ml:id xml:space=\"preserve\"><Span xmlns=\"http://schemas.microsoft.com/winfx/2006/xaml/presentation\" xmlns:pw=\"clr-namespace:Ptc.Wpf;assembly=Ptc.Core\">AC<pw:Subscript>Cdc</pw:Subscript></Span></ml:id><ml:real>599</ml:real><ml:apply><ml:id xml:space=\"preserve\">last</ml:id><ml:id xml:space=\"preserve\"><Span xmlns=\"http://schemas.microsoft.com/winfx/2006/xaml/presentation\" xmlns:pw=\"clr-namespace:Ptc.Wpf;assembly=Ptc.Core\">AC<pw:Subscript>Cdc</pw:Subscript></Span></ml:id></ml:apply><ml:real>0</ml:real><ml:real>0</ml:real></ml:sequence></ml:apply></ml:program></ml:then><ml:else><ml:program><ml:apply><ml:id xml:space=\"preserve\">submatrix</ml:id><ml:sequence><ml:id xml:space=\"preserve\"><Span xmlns=\"http://schemas.microsoft.com/winfx/2006/xaml/presentation\" xmlns:pw=\"clr-namespace:Ptc.Wpf;assembly=Ptc.Core\">AC<pw:Subscript>Cdc</pw:Subscript></Span></ml:id><ml:real>599</ml:real><ml:real>1197</ml:real><ml:real>0</ml:real><ml:real>0</ml:real></ml:sequence></ml:apply></ml:program></ml:else></ml:if></ml:program></ml:define></math><mc14-conversion-loss-annotations><annotation>Otherwise</annotation></mc14-conversion-loss-annotations></region><region top=\"13570.5605\" width=\"447\" left=\"57.6\" height=\"49\" converted-from=\"Mathcad14\" region-id=\"367\"><math><ml:define><ml:id label=\"Variable\" xml:space=\"preserve\"><Span xmlns=\"http://schemas.microsoft.com/winfx/2006/xaml/presentation\" xmlns:pw=\"clr-namespace:Ptc.Wpf;assembly=Ptc.Core\">AC<pw:Subscript>CdcC</pw:Subscript></Span></ml:id><ml:program><ml:if><ml:test><ml:apply><ml:lessThan /><ml:apply><ml:id xml:space=\"preserve\">last</ml:id><ml:id xml:space=\"preserve\"><Span xmlns=\"http://schemas.microsoft.com/winfx/2006/xaml/presentation\" xmlns:pw=\"clr-namespace:Ptc.Wpf;assembly=Ptc.Core\">AC<pw:Subscript>Cdc</pw:Subscript></Span></ml:id></ml:apply><ml:real>1796</ml:real></ml:apply></ml:test><ml:then><ml:program><ml:apply><ml:id xml:space=\"preserve\">submatrix</ml:id><ml:sequence><ml:id xml:space=\"preserve\"><Span xmlns=\"http://schemas.microsoft.com/winfx/2006/xaml/presentation\" xmlns:pw=\"clr-namespace:Ptc.Wpf;assembly=Ptc.Core\">AC<pw:Subscript>Cdc</pw:Subscript></Span></ml:id><ml:real>1198</ml:real><ml:apply><ml:id xml:space=\"preserve\">last</ml:id><ml:id xml:space=\"preserve\"><Span xmlns=\"http://schemas.microsoft.com/winfx/2006/xaml/presentation\" xmlns:pw=\"clr-namespace:Ptc.Wpf;assembly=Ptc.Core\">AC<pw:Subscript>Cdc</pw:Subscript></Span></ml:id></ml:apply><ml:real>0</ml:real><ml:real>0</ml:real></ml:sequence></ml:apply></ml:program></ml:then><ml:else><ml:program><ml:apply><ml:id xml:space=\"preserve\">submatrix</ml:id><ml:sequence><ml:id xml:space=\"preserve\"><Span xmlns=\"http://schemas.microsoft.com/winfx/2006/xaml/presentation\" xmlns:pw=\"clr-namespace:Ptc.Wpf;assembly=Ptc.Core\">AC<pw:Subscript>Cdc</pw:Subscript></Span></ml:id><ml:real>1198</ml:real><ml:real>1796</ml:real><ml:real>0</ml:real><ml:real>0</ml:real></ml:sequence></ml:apply></ml:program></ml:else></ml:if></ml:program></ml:define></math><mc14-conversion-loss-annotations><annotation>Otherwise</annotation></mc14-conversion-loss-annotations></region><region top=\"13676.1611\" width=\"363\" left=\"652.8\" height=\"49\" converted-from=\"Mathcad14\" region-id=\"368\"><math><ml:define><ml:id label=\"Variable\" xml:space=\"preserve\"><Span xmlns=\"http://schemas.microsoft.com/winfx/2006/xaml/presentation\" xmlns:pw=\"clr-namespace:Ptc.Wpf;assembly=Ptc.Core\">AC<pw:Subscript>SedTankA</pw:Subscript></Span></ml:id><ml:program><ml:if><ml:test><ml:apply><ml:lessThan /><ml:apply><ml:id xml:space=\"preserve\">last</ml:id><ml:id xml:space=\"preserve\"><Span xmlns=\"http://schemas.microsoft.com/winfx/2006/xaml/presentation\" xmlns:pw=\"clr-namespace:Ptc.Wpf;assembly=Ptc.Core\">AC<pw:Subscript>SedTank</pw:Subscript></Span></ml:id></ml:apply><ml:real>598</ml:real></ml:apply></ml:test><ml:then><ml:program><ml:id xml:space=\"preserve\"><Span xmlns=\"http://schemas.microsoft.com/winfx/2006/xaml/presentation\" xmlns:pw=\"clr-namespace:Ptc.Wpf;assembly=Ptc.Core\">AC<pw:Subscript>SedTank</pw:Subscript></Span></ml:id></ml:program></ml:then><ml:else><ml:program><ml:apply><ml:id xml:space=\"preserve\">submatrix</ml:id><ml:sequence><ml:id xml:space=\"preserve\"><Span xmlns=\"http://schemas.microsoft.com/winfx/2006/xaml/presentation\" xmlns:pw=\"clr-namespace:Ptc.Wpf;assembly=Ptc.Core\">AC<pw:Subscript>SedTank</pw:Subscript></Span></ml:id><ml:real>0</ml:real><ml:real>598</ml:real><ml:real>0</ml:real><ml:real>0</ml:real></ml:sequence></ml:apply></ml:program></ml:else></ml:if></ml:program></ml:define></math><mc14-conversion-loss-annotations><annotation>Otherwise</annotation></mc14-conversion-loss-annotations></region><region top=\"13714.5605\" width=\"323\" left=\"67.2\" height=\"49\" converted-from=\"Mathcad14\" region-id=\"369\"><math><ml:define><ml:id label=\"Variable\" xml:space=\"preserve\"><Span xmlns=\"http://schemas.microsoft.com/winfx/2006/xaml/presentation\" xmlns:pw=\"clr-namespace:Ptc.Wpf;assembly=Ptc.Core\">AC<pw:Subscript>FilterA</pw:Subscript></Span></ml:id><ml:program><ml:if><ml:test><ml:apply><ml:lessThan /><ml:apply><ml:id xml:space=\"preserve\">last</ml:id><ml:id xml:space=\"preserve\"><Span xmlns=\"http://schemas.microsoft.com/winfx/2006/xaml/presentation\" xmlns:pw=\"clr-namespace:Ptc.Wpf;assembly=Ptc.Core\">AC<pw:Subscript>Filter</pw:Subscript></Span></ml:id></ml:apply><ml:real>598</ml:real></ml:apply></ml:test><ml:then><ml:program><ml:id xml:space=\"preserve\"><Span xmlns=\"http://schemas.microsoft.com/winfx/2006/xaml/presentation\" xmlns:pw=\"clr-namespace:Ptc.Wpf;assembly=Ptc.Core\">AC<pw:Subscript>Filter</pw:Subscript></Span></ml:id></ml:program></ml:then><ml:else><ml:program><ml:apply><ml:id xml:space=\"preserve\">submatrix</ml:id><ml:sequence><ml:id xml:space=\"preserve\"><Span xmlns=\"http://schemas.microsoft.com/winfx/2006/xaml/presentation\" xmlns:pw=\"clr-namespace:Ptc.Wpf;assembly=Ptc.Core\">AC<pw:Subscript>Filter</pw:Subscript></Span></ml:id><ml:real>0</ml:real><ml:real>598</ml:real><ml:real>0</ml:real><ml:real>0</ml:real></ml:sequence></ml:apply></ml:program></ml:else></ml:if></ml:program></ml:define></math><mc14-conversion-loss-annotations><annotation>Otherwise</annotation></mc14-conversion-loss-annotations></region><region top=\"13781.7607\" width=\"548\" left=\"652.8\" height=\"49\" converted-from=\"Mathcad14\" region-id=\"370\"><math><ml:define><ml:id label=\"Variable\" xml:space=\"preserve\"><Span xmlns=\"http://schemas.microsoft.com/winfx/2006/xaml/presentation\" xmlns:pw=\"clr-namespace:Ptc.Wpf;assembly=Ptc.Core\">AC<pw:Subscript>SedTankB</pw:Subscript></Span></ml:id><ml:program><ml:if><ml:test><ml:apply><ml:lessThan /><ml:apply><ml:id xml:space=\"preserve\">last</ml:id><ml:id xml:space=\"preserve\"><Span xmlns=\"http://schemas.microsoft.com/winfx/2006/xaml/presentation\" xmlns:pw=\"clr-namespace:Ptc.Wpf;assembly=Ptc.Core\">AC<pw:Subscript>SedTank</pw:Subscript></Span></ml:id></ml:apply><ml:real>1197</ml:real></ml:apply></ml:test><ml:then><ml:program><ml:apply><ml:id xml:space=\"preserve\">submatrix</ml:id><ml:sequence><ml:id xml:space=\"preserve\"><Span xmlns=\"http://schemas.microsoft.com/winfx/2006/xaml/presentation\" xmlns:pw=\"clr-namespace:Ptc.Wpf;assembly=Ptc.Core\">AC<pw:Subscript>SedTank</pw:Subscript></Span></ml:id><ml:real>599</ml:real><ml:apply><ml:id xml:space=\"preserve\">last</ml:id><ml:id xml:space=\"preserve\"><Span xmlns=\"http://schemas.microsoft.com/winfx/2006/xaml/presentation\" xmlns:pw=\"clr-namespace:Ptc.Wpf;assembly=Ptc.Core\">AC<pw:Subscript>SedTank</pw:Subscript></Span></ml:id></ml:apply><ml:real>0</ml:real><ml:real>0</ml:real></ml:sequence></ml:apply></ml:program></ml:then><ml:else><ml:program><ml:apply><ml:id xml:space=\"preserve\">submatrix</ml:id><ml:sequence><ml:id xml:space=\"preserve\"><Span xmlns=\"http://schemas.microsoft.com/winfx/2006/xaml/presentation\" xmlns:pw=\"clr-namespace:Ptc.Wpf;assembly=Ptc.Core\">AC<pw:Subscript>SedTank</pw:Subscript></Span></ml:id><ml:real>599</ml:real><ml:real>1197</ml:real><ml:real>0</ml:real><ml:real>0</ml:real></ml:sequence></ml:apply></ml:program></ml:else></ml:if></ml:program></ml:define></math><mc14-conversion-loss-annotations><annotation>Otherwise</annotation></mc14-conversion-loss-annotations></region><region top=\"13820.1611\" width=\"468\" left=\"67.2\" height=\"49\" converted-from=\"Mathcad14\" region-id=\"371\"><math><ml:define><ml:id label=\"Variable\" xml:space=\"preserve\"><Span xmlns=\"http://schemas.microsoft.com/winfx/2006/xaml/presentation\" xmlns:pw=\"clr-namespace:Ptc.Wpf;assembly=Ptc.Core\">AC<pw:Subscript>FilterB</pw:Subscript></Span></ml:id><ml:program><ml:if><ml:test><ml:apply><ml:lessThan /><ml:apply><ml:id xml:space=\"preserve\">last</ml:id><ml:id xml:space=\"preserve\"><Span xmlns=\"http://schemas.microsoft.com/winfx/2006/xaml/presentation\" xmlns:pw=\"clr-namespace:Ptc.Wpf;assembly=Ptc.Core\">AC<pw:Subscript>Filter</pw:Subscript></Span></ml:id></ml:apply><ml:real>1197</ml:real></ml:apply></ml:test><ml:then><ml:program><ml:apply><ml:id xml:space=\"preserve\">submatrix</ml:id><ml:sequence><ml:id xml:space=\"preserve\"><Span xmlns=\"http://schemas.microsoft.com/winfx/2006/xaml/presentation\" xmlns:pw=\"clr-namespace:Ptc.Wpf;assembly=Ptc.Core\">AC<pw:Subscript>Filter</pw:Subscript></Span></ml:id><ml:real>599</ml:real><ml:apply><ml:id xml:space=\"preserve\">last</ml:id><ml:id xml:space=\"preserve\"><Span xmlns=\"http://schemas.microsoft.com/winfx/2006/xaml/presentation\" xmlns:pw=\"clr-namespace:Ptc.Wpf;assembly=Ptc.Core\">AC<pw:Subscript>Filter</pw:Subscript></Span></ml:id></ml:apply><ml:real>0</ml:real><ml:real>0</ml:real></ml:sequence></ml:apply></ml:program></ml:then><ml:else><ml:program><ml:apply><ml:id xml:space=\"preserve\">submatrix</ml:id><ml:sequence><ml:id xml:space=\"preserve\"><Span xmlns=\"http://schemas.microsoft.com/winfx/2006/xaml/presentation\" xmlns:pw=\"clr-namespace:Ptc.Wpf;assembly=Ptc.Core\">AC<pw:Subscript>Filter</pw:Subscript></Span></ml:id><ml:real>599</ml:real><ml:real>1197</ml:real><ml:real>0</ml:real><ml:real>0</ml:real></ml:sequence></ml:apply></ml:program></ml:else></ml:if></ml:program></ml:define></math><mc14-conversion-loss-annotations><annotation>Otherwise</annotation></mc14-conversion-loss-annotations></region><region top=\"13868.1611\" width=\"554\" left=\"652.8\" height=\"49\" converted-from=\"Mathcad14\" region-id=\"372\"><math><ml:define><ml:id label=\"Variable\" xml:space=\"preserve\"><Span xmlns=\"http://schemas.microsoft.com/winfx/2006/xaml/presentation\" xmlns:pw=\"clr-namespace:Ptc.Wpf;assembly=Ptc.Core\">AC<pw:Subscript>SedTankC</pw:Subscript></Span></ml:id><ml:program><ml:if><ml:test><ml:apply><ml:lessThan /><ml:apply><ml:id xml:space=\"preserve\">last</ml:id><ml:id xml:space=\"preserve\"><Span xmlns=\"http://schemas.microsoft.com/winfx/2006/xaml/presentation\" xmlns:pw=\"clr-namespace:Ptc.Wpf;assembly=Ptc.Core\">AC<pw:Subscript>SedTank</pw:Subscript></Span></ml:id></ml:apply><ml:real>1796</ml:real></ml:apply></ml:test><ml:then><ml:program><ml:apply><ml:id xml:space=\"preserve\">submatrix</ml:id><ml:sequence><ml:id xml:space=\"preserve\"><Span xmlns=\"http://schemas.microsoft.com/winfx/2006/xaml/presentation\" xmlns:pw=\"clr-namespace:Ptc.Wpf;assembly=Ptc.Core\">AC<pw:Subscript>SedTank</pw:Subscript></Span></ml:id><ml:real>1198</ml:real><ml:apply><ml:id xml:space=\"preserve\">last</ml:id><ml:id xml:space=\"preserve\"><Span xmlns=\"http://schemas.microsoft.com/winfx/2006/xaml/presentation\" xmlns:pw=\"clr-namespace:Ptc.Wpf;assembly=Ptc.Core\">AC<pw:Subscript>SedTank</pw:Subscript></Span></ml:id></ml:apply><ml:real>0</ml:real><ml:real>0</ml:real></ml:sequence></ml:apply></ml:program></ml:then><ml:else><ml:program><ml:apply><ml:id xml:space=\"preserve\">submatrix</ml:id><ml:sequence><ml:id xml:space=\"preserve\"><Span xmlns=\"http://schemas.microsoft.com/winfx/2006/xaml/presentation\" xmlns:pw=\"clr-namespace:Ptc.Wpf;assembly=Ptc.Core\">AC<pw:Subscript>SedTank</pw:Subscript></Span></ml:id><ml:real>1198</ml:real><ml:real>1796</ml:real><ml:real>0</ml:real><ml:real>0</ml:real></ml:sequence></ml:apply></ml:program></ml:else></ml:if></ml:program></ml:define></math><mc14-conversion-loss-annotations><annotation>Otherwise</annotation></mc14-conversion-loss-annotations></region><region top=\"13906.5605\" width=\"474\" left=\"67.2\" height=\"49\" converted-from=\"Mathcad14\" region-id=\"373\"><math><ml:define><ml:id label=\"Variable\" xml:space=\"preserve\"><Span xmlns=\"http://schemas.microsoft.com/winfx/2006/xaml/presentation\" xmlns:pw=\"clr-namespace:Ptc.Wpf;assembly=Ptc.Core\">AC<pw:Subscript>FilterC</pw:Subscript></Span></ml:id><ml:program><ml:if><ml:test><ml:apply><ml:lessThan /><ml:apply><ml:id xml:space=\"preserve\">last</ml:id><ml:id xml:space=\"preserve\"><Span xmlns=\"http://schemas.microsoft.com/winfx/2006/xaml/presentation\" xmlns:pw=\"clr-namespace:Ptc.Wpf;assembly=Ptc.Core\">AC<pw:Subscript>Filter</pw:Subscript></Span></ml:id></ml:apply><ml:real>1796</ml:real></ml:apply></ml:test><ml:then><ml:program><ml:apply><ml:id xml:space=\"preserve\">submatrix</ml:id><ml:sequence><ml:id xml:space=\"preserve\"><Span xmlns=\"http://schemas.microsoft.com/winfx/2006/xaml/presentation\" xmlns:pw=\"clr-namespace:Ptc.Wpf;assembly=Ptc.Core\">AC<pw:Subscript>Filter</pw:Subscript></Span></ml:id><ml:real>1198</ml:real><ml:apply><ml:id xml:space=\"preserve\">last</ml:id><ml:id xml:space=\"preserve\"><Span xmlns=\"http://schemas.microsoft.com/winfx/2006/xaml/presentation\" xmlns:pw=\"clr-namespace:Ptc.Wpf;assembly=Ptc.Core\">AC<pw:Subscript>Filter</pw:Subscript></Span></ml:id></ml:apply><ml:real>0</ml:real><ml:real>0</ml:real></ml:sequence></ml:apply></ml:program></ml:then><ml:else><ml:program><ml:apply><ml:id xml:space=\"preserve\">submatrix</ml:id><ml:sequence><ml:id xml:space=\"preserve\"><Span xmlns=\"http://schemas.microsoft.com/winfx/2006/xaml/presentation\" xmlns:pw=\"clr-namespace:Ptc.Wpf;assembly=Ptc.Core\">AC<pw:Subscript>Filter</pw:Subscript></Span></ml:id><ml:real>1198</ml:real><ml:real>1796</ml:real><ml:real>0</ml:real><ml:real>0</ml:real></ml:sequence></ml:apply></ml:program></ml:else></ml:if></ml:program></ml:define></math><mc14-conversion-loss-annotations><annotation>Otherwise</annotation></mc14-conversion-loss-annotations></region><region top=\"13954.5605\" width=\"394\" left=\"652.8\" height=\"49\" converted-from=\"Mathcad14\" region-id=\"374\"><math><ml:define><ml:id label=\"Variable\" xml:space=\"preserve\"><Span xmlns=\"http://schemas.microsoft.com/winfx/2006/xaml/presentation\" xmlns:pw=\"clr-namespace:Ptc.Wpf;assembly=Ptc.Core\">AC<pw:Subscript>ChemTanksA</pw:Subscript></Span></ml:id><ml:program><ml:if><ml:test><ml:apply><ml:lessThan /><ml:apply><ml:id xml:space=\"preserve\">last</ml:id><ml:id xml:space=\"preserve\"><Span xmlns=\"http://schemas.microsoft.com/winfx/2006/xaml/presentation\" xmlns:pw=\"clr-namespace:Ptc.Wpf;assembly=Ptc.Core\">AC<pw:Subscript>ChemTanks</pw:Subscript></Span></ml:id></ml:apply><ml:real>598</ml:real></ml:apply></ml:test><ml:then><ml:program><ml:id xml:space=\"preserve\"><Span xmlns=\"http://schemas.microsoft.com/winfx/2006/xaml/presentation\" xmlns:pw=\"clr-namespace:Ptc.Wpf;assembly=Ptc.Core\">AC<pw:Subscript>ChemTanks</pw:Subscript></Span></ml:id></ml:program></ml:then><ml:else><ml:program><ml:apply><ml:id xml:space=\"preserve\">submatrix</ml:id><ml:sequence><ml:id xml:space=\"preserve\"><Span xmlns=\"http://schemas.microsoft.com/winfx/2006/xaml/presentation\" xmlns:pw=\"clr-namespace:Ptc.Wpf;assembly=Ptc.Core\">AC<pw:Subscript>ChemTanks</pw:Subscript></Span></ml:id><ml:real>0</ml:real><ml:real>598</ml:real><ml:real>0</ml:real><ml:real>0</ml:real></ml:sequence></ml:apply></ml:program></ml:else></ml:if></ml:program></ml:define></math><mc14-conversion-loss-annotations><annotation>Otherwise</annotation></mc14-conversion-loss-annotations></region><region top=\"13992.9609\" width=\"475\" left=\"57.6\" height=\"49\" converted-from=\"Mathcad14\" region-id=\"375\"><math><ml:define><ml:id label=\"Variable\" xml:space=\"preserve\"><Span xmlns=\"http://schemas.microsoft.com/winfx/2006/xaml/presentation\" xmlns:pw=\"clr-namespace:Ptc.Wpf;assembly=Ptc.Core\">AC<pw:Subscript>FilterD</pw:Subscript></Span></ml:id><ml:program><ml:if><ml:test><ml:apply><ml:lessThan /><ml:apply><ml:id xml:space=\"preserve\">last</ml:id><ml:id xml:space=\"preserve\"><Span xmlns=\"http://schemas.microsoft.com/winfx/2006/xaml/presentation\" xmlns:pw=\"clr-namespace:Ptc.Wpf;assembly=Ptc.Core\">AC<pw:Subscript>Filter</pw:Subscript></Span></ml:id></ml:apply><ml:real>2395</ml:real></ml:apply></ml:test><ml:then><ml:program><ml:apply><ml:id xml:space=\"preserve\">submatrix</ml:id><ml:sequence><ml:id xml:space=\"preserve\"><Span xmlns=\"http://schemas.microsoft.com/winfx/2006/xaml/presentation\" xmlns:pw=\"clr-namespace:Ptc.Wpf;assembly=Ptc.Core\">AC<pw:Subscript>Filter</pw:Subscript></Span></ml:id><ml:real>1797</ml:real><ml:apply><ml:id xml:space=\"preserve\">last</ml:id><ml:id xml:space=\"preserve\"><Span xmlns=\"http://schemas.microsoft.com/winfx/2006/xaml/presentation\" xmlns:pw=\"clr-namespace:Ptc.Wpf;assembly=Ptc.Core\">AC<pw:Subscript>Filter</pw:Subscript></Span></ml:id></ml:apply><ml:real>0</ml:real><ml:real>0</ml:real></ml:sequence></ml:apply></ml:program></ml:then><ml:else><ml:program><ml:apply><ml:id xml:space=\"preserve\">submatrix</ml:id><ml:sequence><ml:id xml:space=\"preserve\"><Span xmlns=\"http://schemas.microsoft.com/winfx/2006/xaml/presentation\" xmlns:pw=\"clr-namespace:Ptc.Wpf;assembly=Ptc.Core\">AC<pw:Subscript>Filter</pw:Subscript></Span></ml:id><ml:real>1797</ml:real><ml:real>2395</ml:real><ml:real>0</ml:real><ml:real>0</ml:real></ml:sequence></ml:apply></ml:program></ml:else></ml:if></ml:program></ml:define></math><mc14-conversion-loss-annotations><annotation>Otherwise</annotation></mc14-conversion-loss-annotations></region><region top=\"14098.5605\" width=\"369\" left=\"67.2\" height=\"49\" converted-from=\"Mathcad14\" region-id=\"376\"><math><ml:define><ml:id label=\"Variable\" xml:space=\"preserve\"><Span xmlns=\"http://schemas.microsoft.com/winfx/2006/xaml/presentation\" xmlns:pw=\"clr-namespace:Ptc.Wpf;assembly=Ptc.Core\">AC<pw:Subscript>FlocTankA</pw:Subscript></Span></ml:id><ml:program><ml:if><ml:test><ml:apply><ml:lessThan /><ml:apply><ml:id xml:space=\"preserve\">last</ml:id><ml:id xml:space=\"preserve\"><Span xmlns=\"http://schemas.microsoft.com/winfx/2006/xaml/presentation\" xmlns:pw=\"clr-namespace:Ptc.Wpf;assembly=Ptc.Core\">AC<pw:Subscript>FlocTank</pw:Subscript></Span></ml:id></ml:apply><ml:real>598</ml:real></ml:apply></ml:test><ml:then><ml:program><ml:id xml:space=\"preserve\"><Span xmlns=\"http://schemas.microsoft.com/winfx/2006/xaml/presentation\" xmlns:pw=\"clr-namespace:Ptc.Wpf;assembly=Ptc.Core\">AC<pw:Subscript>FlocTank</pw:Subscript></Span></ml:id></ml:program></ml:then><ml:else><ml:program><ml:apply><ml:id xml:space=\"preserve\">submatrix</ml:id><ml:sequence><ml:id xml:space=\"preserve\"><Span xmlns=\"http://schemas.microsoft.com/winfx/2006/xaml/presentation\" xmlns:pw=\"clr-namespace:Ptc.Wpf;assembly=Ptc.Core\">AC<pw:Subscript>FlocTank</pw:Subscript></Span></ml:id><ml:real>0</ml:real><ml:real>598</ml:real><ml:real>0</ml:real><ml:real>0</ml:real></ml:sequence></ml:apply></ml:program></ml:else></ml:if></ml:program></ml:define></math><mc14-conversion-loss-annotations><annotation>Otherwise</annotation></mc14-conversion-loss-annotations></region><region top=\"14156.1611\" width=\"609\" left=\"652.8\" height=\"49\" converted-from=\"Mathcad14\" region-id=\"377\"><math><ml:define><ml:id label=\"Variable\" xml:space=\"preserve\"><Span xmlns=\"http://schemas.microsoft.com/winfx/2006/xaml/presentation\" xmlns:pw=\"clr-namespace:Ptc.Wpf;assembly=Ptc.Core\">AC<pw:Subscript>ChemTanksB</pw:Subscript></Span></ml:id><ml:program><ml:if><ml:test><ml:apply><ml:lessThan /><ml:apply><ml:id xml:space=\"preserve\">last</ml:id><ml:id xml:space=\"preserve\"><Span xmlns=\"http://schemas.microsoft.com/winfx/2006/xaml/presentation\" xmlns:pw=\"clr-namespace:Ptc.Wpf;assembly=Ptc.Core\">AC<pw:Subscript>ChemTanks</pw:Subscript></Span></ml:id></ml:apply><ml:real>1197</ml:real></ml:apply></ml:test><ml:then><ml:program><ml:apply><ml:id xml:space=\"preserve\">submatrix</ml:id><ml:sequence><ml:id xml:space=\"preserve\"><Span xmlns=\"http://schemas.microsoft.com/winfx/2006/xaml/presentation\" xmlns:pw=\"clr-namespace:Ptc.Wpf;assembly=Ptc.Core\">AC<pw:Subscript>ChemTanks</pw:Subscript></Span></ml:id><ml:real>599</ml:real><ml:apply><ml:id xml:space=\"preserve\">last</ml:id><ml:id xml:space=\"preserve\"><Span xmlns=\"http://schemas.microsoft.com/winfx/2006/xaml/presentation\" xmlns:pw=\"clr-namespace:Ptc.Wpf;assembly=Ptc.Core\">AC<pw:Subscript>ChemTanks</pw:Subscript></Span></ml:id></ml:apply><ml:real>0</ml:real><ml:real>0</ml:real></ml:sequence></ml:apply></ml:program></ml:then><ml:else><ml:program><ml:apply><ml:id xml:space=\"preserve\">submatrix</ml:id><ml:sequence><ml:id xml:space=\"preserve\"><Span xmlns=\"http://schemas.microsoft.com/winfx/2006/xaml/presentation\" xmlns:pw=\"clr-namespace:Ptc.Wpf;assembly=Ptc.Core\">AC<pw:Subscript>ChemTanks</pw:Subscript></Span></ml:id><ml:real>599</ml:real><ml:real>1197</ml:real><ml:real>0</ml:real><ml:real>0</ml:real></ml:sequence></ml:apply></ml:program></ml:else></ml:if></ml:program></ml:define></math><mc14-conversion-loss-annotations><annotation>Otherwise</annotation></mc14-conversion-loss-annotations></region><region top=\"14194.5605\" width=\"560\" left=\"67.2\" height=\"49\" converted-from=\"Mathcad14\" region-id=\"378\"><math><ml:define><ml:id label=\"Variable\" xml:space=\"preserve\"><Span xmlns=\"http://schemas.microsoft.com/winfx/2006/xaml/presentation\" xmlns:pw=\"clr-namespace:Ptc.Wpf;assembly=Ptc.Core\">AC<pw:Subscript>FlocTankB</pw:Subscript></Span></ml:id><ml:program><ml:if><ml:test><ml:apply><ml:lessThan /><ml:apply><ml:id xml:space=\"preserve\">last</ml:id><ml:id xml:space=\"preserve\"><Span xmlns=\"http://schemas.microsoft.com/winfx/2006/xaml/presentation\" xmlns:pw=\"clr-namespace:Ptc.Wpf;assembly=Ptc.Core\">AC<pw:Subscript>FlocTank</pw:Subscript></Span></ml:id></ml:apply><ml:real>1197</ml:real></ml:apply></ml:test><ml:then><ml:program><ml:apply><ml:id xml:space=\"preserve\">submatrix</ml:id><ml:sequence><ml:id xml:space=\"preserve\"><Span xmlns=\"http://schemas.microsoft.com/winfx/2006/xaml/presentation\" xmlns:pw=\"clr-namespace:Ptc.Wpf;assembly=Ptc.Core\">AC<pw:Subscript>FlocTank</pw:Subscript></Span></ml:id><ml:real>599</ml:real><ml:apply><ml:id xml:space=\"preserve\">last</ml:id><ml:id xml:space=\"preserve\"><Span xmlns=\"http://schemas.microsoft.com/winfx/2006/xaml/presentation\" xmlns:pw=\"clr-namespace:Ptc.Wpf;assembly=Ptc.Core\">AC<pw:Subscript>FlocTank</pw:Subscript></Span></ml:id></ml:apply><ml:real>0</ml:real><ml:real>0</ml:real></ml:sequence></ml:apply></ml:program></ml:then><ml:else><ml:program><ml:apply><ml:id xml:space=\"preserve\">submatrix</ml:id><ml:sequence><ml:id xml:space=\"preserve\"><Span xmlns=\"http://schemas.microsoft.com/winfx/2006/xaml/presentation\" xmlns:pw=\"clr-namespace:Ptc.Wpf;assembly=Ptc.Core\">AC<pw:Subscript>FlocTank</pw:Subscript></Span></ml:id><ml:real>599</ml:real><ml:real>1197</ml:real><ml:real>0</ml:real><ml:real>0</ml:real></ml:sequence></ml:apply></ml:program></ml:else></ml:if></ml:program></ml:define></math><mc14-conversion-loss-annotations><annotation>Otherwise</annotation></mc14-conversion-loss-annotations></region><region top=\"14261.7607\" width=\"615\" left=\"652.8\" height=\"49\" converted-from=\"Mathcad14\" region-id=\"379\"><math><ml:define><ml:id label=\"Variable\" xml:space=\"preserve\"><Span xmlns=\"http://schemas.microsoft.com/winfx/2006/xaml/presentation\" xmlns:pw=\"clr-namespace:Ptc.Wpf;assembly=Ptc.Core\">AC<pw:Subscript>ChemTanksC</pw:Subscript></Span></ml:id><ml:program><ml:if><ml:test><ml:apply><ml:lessThan /><ml:apply><ml:id xml:space=\"preserve\">last</ml:id><ml:id xml:space=\"preserve\"><Span xmlns=\"http://schemas.microsoft.com/winfx/2006/xaml/presentation\" xmlns:pw=\"clr-namespace:Ptc.Wpf;assembly=Ptc.Core\">AC<pw:Subscript>ChemTanks</pw:Subscript></Span></ml:id></ml:apply><ml:real>1796</ml:real></ml:apply></ml:test><ml:then><ml:program><ml:apply><ml:id xml:space=\"preserve\">submatrix</ml:id><ml:sequence><ml:id xml:space=\"preserve\"><Span xmlns=\"http://schemas.microsoft.com/winfx/2006/xaml/presentation\" xmlns:pw=\"clr-namespace:Ptc.Wpf;assembly=Ptc.Core\">AC<pw:Subscript>ChemTanks</pw:Subscript></Span></ml:id><ml:real>1198</ml:real><ml:apply><ml:id xml:space=\"preserve\">last</ml:id><ml:id xml:space=\"preserve\"><Span xmlns=\"http://schemas.microsoft.com/winfx/2006/xaml/presentation\" xmlns:pw=\"clr-namespace:Ptc.Wpf;assembly=Ptc.Core\">AC<pw:Subscript>ChemTanks</pw:Subscript></Span></ml:id></ml:apply><ml:real>0</ml:real><ml:real>0</ml:real></ml:sequence></ml:apply></ml:program></ml:then><ml:else><ml:program><ml:apply><ml:id xml:space=\"preserve\">submatrix</ml:id><ml:sequence><ml:id xml:space=\"preserve\"><Span xmlns=\"http://schemas.microsoft.com/winfx/2006/xaml/presentation\" xmlns:pw=\"clr-namespace:Ptc.Wpf;assembly=Ptc.Core\">AC<pw:Subscript>ChemTanks</pw:Subscript></Span></ml:id><ml:real>1198</ml:real><ml:real>1796</ml:real><ml:real>0</ml:real><ml:real>0</ml:real></ml:sequence></ml:apply></ml:program></ml:else></ml:if></ml:program></ml:define></math><mc14-conversion-loss-annotations><annotation>Otherwise</annotation></mc14-conversion-loss-annotations></region><region top=\"14300.1611\" width=\"566\" left=\"67.2\" height=\"49\" converted-from=\"Mathcad14\" region-id=\"380\"><math><ml:define><ml:id label=\"Variable\" xml:space=\"preserve\"><Span xmlns=\"http://schemas.microsoft.com/winfx/2006/xaml/presentation\" xmlns:pw=\"clr-namespace:Ptc.Wpf;assembly=Ptc.Core\">AC<pw:Subscript>FlocTankC</pw:Subscript></Span></ml:id><ml:program><ml:if><ml:test><ml:apply><ml:lessThan /><ml:apply><ml:id xml:space=\"preserve\">last</ml:id><ml:id xml:space=\"preserve\"><Span xmlns=\"http://schemas.microsoft.com/winfx/2006/xaml/presentation\" xmlns:pw=\"clr-namespace:Ptc.Wpf;assembly=Ptc.Core\">AC<pw:Subscript>FlocTank</pw:Subscript></Span></ml:id></ml:apply><ml:real>1796</ml:real></ml:apply></ml:test><ml:then><ml:program><ml:apply><ml:id xml:space=\"preserve\">submatrix</ml:id><ml:sequence><ml:id xml:space=\"preserve\"><Span xmlns=\"http://schemas.microsoft.com/winfx/2006/xaml/presentation\" xmlns:pw=\"clr-namespace:Ptc.Wpf;assembly=Ptc.Core\">AC<pw:Subscript>FlocTank</pw:Subscript></Span></ml:id><ml:real>1198</ml:real><ml:apply><ml:id xml:space=\"preserve\">last</ml:id><ml:id xml:space=\"preserve\"><Span xmlns=\"http://schemas.microsoft.com/winfx/2006/xaml/presentation\" xmlns:pw=\"clr-namespace:Ptc.Wpf;assembly=Ptc.Core\">AC<pw:Subscript>FlocTank</pw:Subscript></Span></ml:id></ml:apply><ml:real>0</ml:real><ml:real>0</ml:real></ml:sequence></ml:apply></ml:program></ml:then><ml:else><ml:program><ml:apply><ml:id xml:space=\"preserve\">submatrix</ml:id><ml:sequence><ml:id xml:space=\"preserve\"><Span xmlns=\"http://schemas.microsoft.com/winfx/2006/xaml/presentation\" xmlns:pw=\"clr-namespace:Ptc.Wpf;assembly=Ptc.Core\">AC<pw:Subscript>FlocTank</pw:Subscript></Span></ml:id><ml:real>1198</ml:real><ml:real>1796</ml:real><ml:real>0</ml:real><ml:real>0</ml:real></ml:sequence></ml:apply></ml:program></ml:else></ml:if></ml:program></ml:define></math><mc14-conversion-loss-annotations><annotation>Otherwise</annotation></mc14-conversion-loss-annotations></region><region top=\"14424.9609\" width=\"544\" left=\"67.2\" height=\"49\" converted-from=\"Mathcad14\" region-id=\"381\"><math><ml:define><ml:id label=\"Variable\" xml:space=\"preserve\"><Span xmlns=\"http://schemas.microsoft.com/winfx/2006/xaml/presentation\" xmlns:pw=\"clr-namespace:Ptc.Wpf;assembly=Ptc.Core\">AC<pw:Subscript>FlocTankD</pw:Subscript></Span></ml:id><ml:program><ml:if><ml:test><ml:apply><ml:lessThan /><ml:apply><ml:id xml:space=\"preserve\">last</ml:id><ml:id xml:space=\"preserve\"><Span xmlns=\"http://schemas.microsoft.com/winfx/2006/xaml/presentation\" xmlns:pw=\"clr-namespace:Ptc.Wpf;assembly=Ptc.Core\">AC<pw:Subscript>FlocTank</pw:Subscript></Span></ml:id></ml:apply><ml:real>2395</ml:real></ml:apply></ml:test><ml:then><ml:program><ml:apply><ml:id xml:space=\"preserve\">submatrix</ml:id><ml:sequence><ml:id xml:space=\"preserve\"><Span xmlns=\"http://schemas.microsoft.com/winfx/2006/xaml/presentation\" xmlns:pw=\"clr-namespace:Ptc.Wpf;assembly=Ptc.Core\">AC<pw:Subscript>FlocTank</pw:Subscript></Span></ml:id><ml:real>1797</ml:real><ml:apply><ml:id xml:space=\"preserve\">last</ml:id><ml:id xml:space=\"preserve\"><Span xmlns=\"http://schemas.microsoft.com/winfx/2006/xaml/presentation\" xmlns:pw=\"clr-namespace:Ptc.Wpf;assembly=Ptc.Core\">AC<pw:Subscript>Filter</pw:Subscript></Span></ml:id></ml:apply><ml:real>0</ml:real><ml:real>0</ml:real></ml:sequence></ml:apply></ml:program></ml:then><ml:else><ml:program><ml:apply><ml:id xml:space=\"preserve\">submatrix</ml:id><ml:sequence><ml:id xml:space=\"preserve\"><Span xmlns=\"http://schemas.microsoft.com/winfx/2006/xaml/presentation\" xmlns:pw=\"clr-namespace:Ptc.Wpf;assembly=Ptc.Core\">AC<pw:Subscript>FlocTank</pw:Subscript></Span></ml:id><ml:real>1797</ml:real><ml:real>2395</ml:real><ml:real>0</ml:real><ml:real>0</ml:real></ml:sequence></ml:apply></ml:program></ml:else></ml:if></ml:program></ml:define></math><mc14-conversion-loss-annotations><annotation>Otherwise</annotation></mc14-conversion-loss-annotations></region><region top=\"14482.5605\" width=\"415\" left=\"652.8\" height=\"49\" converted-from=\"Mathcad14\" region-id=\"382\"><math><ml:define><ml:id label=\"Variable\" xml:space=\"preserve\"><Span xmlns=\"http://schemas.microsoft.com/winfx/2006/xaml/presentation\" xmlns:pw=\"clr-namespace:Ptc.Wpf;assembly=Ptc.Core\">AC<pw:Subscript>DrainChannelA</pw:Subscript></Span></ml:id><ml:program><ml:if><ml:test><ml:apply><ml:lessThan /><ml:apply><ml:id xml:space=\"preserve\">last</ml:id><ml:id xml:space=\"preserve\"><Span xmlns=\"http://schemas.microsoft.com/winfx/2006/xaml/presentation\" xmlns:pw=\"clr-namespace:Ptc.Wpf;assembly=Ptc.Core\">AC<pw:Subscript>DrainChannel</pw:Subscript></Span></ml:id></ml:apply><ml:real>598</ml:real></ml:apply></ml:test><ml:then><ml:program><ml:id xml:space=\"preserve\"><Span xmlns=\"http://schemas.microsoft.com/winfx/2006/xaml/presentation\" xmlns:pw=\"clr-namespace:Ptc.Wpf;assembly=Ptc.Core\">AC<pw:Subscript>DrainChannel</pw:Subscript></Span></ml:id></ml:program></ml:then><ml:else><ml:program><ml:apply><ml:id xml:space=\"preserve\">submatrix</ml:id><ml:sequence><ml:id xml:space=\"preserve\"><Span xmlns=\"http://schemas.microsoft.com/winfx/2006/xaml/presentation\" xmlns:pw=\"clr-namespace:Ptc.Wpf;assembly=Ptc.Core\">AC<pw:Subscript>DrainChannel</pw:Subscript></Span></ml:id><ml:real>0</ml:real><ml:real>598</ml:real><ml:real>0</ml:real><ml:real>0</ml:real></ml:sequence></ml:apply></ml:program></ml:else></ml:if></ml:program></ml:define></math><mc14-conversion-loss-annotations><annotation>Otherwise</annotation></mc14-conversion-loss-annotations></region><region top=\"14520.9609\" width=\"417\" left=\"67.2\" height=\"49\" converted-from=\"Mathcad14\" region-id=\"383\"><math><ml:define><ml:id label=\"Variable\" xml:space=\"preserve\"><Span xmlns=\"http://schemas.microsoft.com/winfx/2006/xaml/presentation\" xmlns:pw=\"clr-namespace:Ptc.Wpf;assembly=Ptc.Core\">AC<pw:Subscript>EntranceTankA</pw:Subscript></Span></ml:id><ml:program><ml:if><ml:test><ml:apply><ml:lessThan /><ml:apply><ml:id xml:space=\"preserve\">last</ml:id><ml:id xml:space=\"preserve\"><Span xmlns=\"http://schemas.microsoft.com/winfx/2006/xaml/presentation\" xmlns:pw=\"clr-namespace:Ptc.Wpf;assembly=Ptc.Core\">AC<pw:Subscript>EntranceTank</pw:Subscript></Span></ml:id></ml:apply><ml:real>598</ml:real></ml:apply></ml:test><ml:then><ml:program><ml:id xml:space=\"preserve\"><Span xmlns=\"http://schemas.microsoft.com/winfx/2006/xaml/presentation\" xmlns:pw=\"clr-namespace:Ptc.Wpf;assembly=Ptc.Core\">AC<pw:Subscript>EntranceTank</pw:Subscript></Span></ml:id></ml:program></ml:then><ml:else><ml:program><ml:apply><ml:id xml:space=\"preserve\">submatrix</ml:id><ml:sequence><ml:id xml:space=\"preserve\"><Span xmlns=\"http://schemas.microsoft.com/winfx/2006/xaml/presentation\" xmlns:pw=\"clr-namespace:Ptc.Wpf;assembly=Ptc.Core\">AC<pw:Subscript>EntranceTank</pw:Subscript></Span></ml:id><ml:real>0</ml:real><ml:real>598</ml:real><ml:real>0</ml:real><ml:real>0</ml:real></ml:sequence></ml:apply></ml:program></ml:else></ml:if></ml:program></ml:define></math><mc14-conversion-loss-annotations><annotation>Otherwise</annotation></mc14-conversion-loss-annotations></region><region top=\"14549.7607\" width=\"658\" left=\"652.8\" height=\"49\" converted-from=\"Mathcad14\" region-id=\"384\"><math><ml:define><ml:id label=\"Variable\" xml:space=\"preserve\"><Span xmlns=\"http://schemas.microsoft.com/winfx/2006/xaml/presentation\" xmlns:pw=\"clr-namespace:Ptc.Wpf;assembly=Ptc.Core\">AC<pw:Subscript>DrainChannelB</pw:Subscript></Span></ml:id><ml:program><ml:if><ml:test><ml:apply><ml:lessThan /><ml:apply><ml:id xml:space=\"preserve\">last</ml:id><ml:id xml:space=\"preserve\"><Span xmlns=\"http://schemas.microsoft.com/winfx/2006/xaml/presentation\" xmlns:pw=\"clr-namespace:Ptc.Wpf;assembly=Ptc.Core\">AC<pw:Subscript>DrainChannel</pw:Subscript></Span></ml:id></ml:apply><ml:real>1197</ml:real></ml:apply></ml:test><ml:then><ml:program><ml:apply><ml:id xml:space=\"preserve\">submatrix</ml:id><ml:sequence><ml:id xml:space=\"preserve\"><Span xmlns=\"http://schemas.microsoft.com/winfx/2006/xaml/presentation\" xmlns:pw=\"clr-namespace:Ptc.Wpf;assembly=Ptc.Core\">AC<pw:Subscript>DrainChannel</pw:Subscript></Span></ml:id><ml:real>1198</ml:real><ml:apply><ml:id xml:space=\"preserve\">last</ml:id><ml:id xml:space=\"preserve\"><Span xmlns=\"http://schemas.microsoft.com/winfx/2006/xaml/presentation\" xmlns:pw=\"clr-namespace:Ptc.Wpf;assembly=Ptc.Core\">AC<pw:Subscript>DrainChannel</pw:Subscript></Span></ml:id></ml:apply><ml:real>0</ml:real><ml:real>0</ml:real></ml:sequence></ml:apply></ml:program></ml:then><ml:else><ml:program><ml:apply><ml:id xml:space=\"preserve\">submatrix</ml:id><ml:sequence><ml:id xml:space=\"preserve\"><Span xmlns=\"http://schemas.microsoft.com/winfx/2006/xaml/presentation\" xmlns:pw=\"clr-namespace:Ptc.Wpf;assembly=Ptc.Core\">AC<pw:Subscript>DrainChannel</pw:Subscript></Span></ml:id><ml:real>1198</ml:real><ml:real>1796</ml:real><ml:real>0</ml:real><ml:real>0</ml:real></ml:sequence></ml:apply></ml:program></ml:else></ml:if></ml:program></ml:define></math><mc14-conversion-loss-annotations><annotation>Otherwise</annotation></mc14-conversion-loss-annotations></region><region top=\"14588.1611\" width=\"656\" left=\"67.2\" height=\"49\" converted-from=\"Mathcad14\" region-id=\"385\"><math><ml:define><ml:id label=\"Variable\" xml:space=\"preserve\"><Span xmlns=\"http://schemas.microsoft.com/winfx/2006/xaml/presentation\" xmlns:pw=\"clr-namespace:Ptc.Wpf;assembly=Ptc.Core\">AC<pw:Subscript>EntranceTankB</pw:Subscript></Span></ml:id><ml:program><ml:if><ml:test><ml:apply><ml:lessThan /><ml:apply><ml:id xml:space=\"preserve\">last</ml:id><ml:id xml:space=\"preserve\"><Span xmlns=\"http://schemas.microsoft.com/winfx/2006/xaml/presentation\" xmlns:pw=\"clr-namespace:Ptc.Wpf;assembly=Ptc.Core\">AC<pw:Subscript>EntranceTank</pw:Subscript></Span></ml:id></ml:apply><ml:real>1197</ml:real></ml:apply></ml:test><ml:then><ml:program><ml:apply><ml:id xml:space=\"preserve\">submatrix</ml:id><ml:sequence><ml:id xml:space=\"preserve\"><Span xmlns=\"http://schemas.microsoft.com/winfx/2006/xaml/presentation\" xmlns:pw=\"clr-namespace:Ptc.Wpf;assembly=Ptc.Core\">AC<pw:Subscript>EntranceTank</pw:Subscript></Span></ml:id><ml:real>599</ml:real><ml:apply><ml:id xml:space=\"preserve\">last</ml:id><ml:id xml:space=\"preserve\"><Span xmlns=\"http://schemas.microsoft.com/winfx/2006/xaml/presentation\" xmlns:pw=\"clr-namespace:Ptc.Wpf;assembly=Ptc.Core\">AC<pw:Subscript>EntranceTank</pw:Subscript></Span></ml:id></ml:apply><ml:real>0</ml:real><ml:real>0</ml:real></ml:sequence></ml:apply></ml:program></ml:then><ml:else><ml:program><ml:apply><ml:id xml:space=\"preserve\">submatrix</ml:id><ml:sequence><ml:id xml:space=\"preserve\"><Span xmlns=\"http://schemas.microsoft.com/winfx/2006/xaml/presentation\" xmlns:pw=\"clr-namespace:Ptc.Wpf;assembly=Ptc.Core\">AC<pw:Subscript>EntranceTank</pw:Subscript></Span></ml:id><ml:real>599</ml:real><ml:real>1197</ml:real><ml:real>0</ml:real><ml:real>0</ml:real></ml:sequence></ml:apply></ml:program></ml:else></ml:if></ml:program></ml:define></math><mc14-conversion-loss-annotations><annotation>Otherwise</annotation></mc14-conversion-loss-annotations></region><region top=\"14636.1611\" width=\"658\" left=\"652.8\" height=\"49\" converted-from=\"Mathcad14\" region-id=\"386\"><math><ml:define><ml:id label=\"Variable\" xml:space=\"preserve\"><Span xmlns=\"http://schemas.microsoft.com/winfx/2006/xaml/presentation\" xmlns:pw=\"clr-namespace:Ptc.Wpf;assembly=Ptc.Core\">AC<pw:Subscript>DrainChannelC</pw:Subscript></Span></ml:id><ml:program><ml:if><ml:test><ml:apply><ml:lessThan /><ml:apply><ml:id xml:space=\"preserve\">last</ml:id><ml:id xml:space=\"preserve\"><Span xmlns=\"http://schemas.microsoft.com/winfx/2006/xaml/presentation\" xmlns:pw=\"clr-namespace:Ptc.Wpf;assembly=Ptc.Core\">AC<pw:Subscript>DrainChannel</pw:Subscript></Span></ml:id></ml:apply><ml:real>1796</ml:real></ml:apply></ml:test><ml:then><ml:program><ml:apply><ml:id xml:space=\"preserve\">submatrix</ml:id><ml:sequence><ml:id xml:space=\"preserve\"><Span xmlns=\"http://schemas.microsoft.com/winfx/2006/xaml/presentation\" xmlns:pw=\"clr-namespace:Ptc.Wpf;assembly=Ptc.Core\">AC<pw:Subscript>DrainChannel</pw:Subscript></Span></ml:id><ml:real>1198</ml:real><ml:apply><ml:id xml:space=\"preserve\">last</ml:id><ml:id xml:space=\"preserve\"><Span xmlns=\"http://schemas.microsoft.com/winfx/2006/xaml/presentation\" xmlns:pw=\"clr-namespace:Ptc.Wpf;assembly=Ptc.Core\">AC<pw:Subscript>DrainChannel</pw:Subscript></Span></ml:id></ml:apply><ml:real>0</ml:real><ml:real>0</ml:real></ml:sequence></ml:apply></ml:program></ml:then><ml:else><ml:program><ml:apply><ml:id xml:space=\"preserve\">submatrix</ml:id><ml:sequence><ml:id xml:space=\"preserve\"><Span xmlns=\"http://schemas.microsoft.com/winfx/2006/xaml/presentation\" xmlns:pw=\"clr-namespace:Ptc.Wpf;assembly=Ptc.Core\">AC<pw:Subscript>DrainChannel</pw:Subscript></Span></ml:id><ml:real>1198</ml:real><ml:real>1796</ml:real><ml:real>0</ml:real><ml:real>0</ml:real></ml:sequence></ml:apply></ml:program></ml:else></ml:if></ml:program></ml:define></math><mc14-conversion-loss-annotations><annotation>Otherwise</annotation></mc14-conversion-loss-annotations></region><region top=\"14674.5605\" width=\"662\" left=\"67.2\" height=\"49\" converted-from=\"Mathcad14\" region-id=\"387\"><math><ml:define><ml:id label=\"Variable\" xml:space=\"preserve\"><Span xmlns=\"http://schemas.microsoft.com/winfx/2006/xaml/presentation\" xmlns:pw=\"clr-namespace:Ptc.Wpf;assembly=Ptc.Core\">AC<pw:Subscript>EntranceTankC</pw:Subscript></Span></ml:id><ml:program><ml:if><ml:test><ml:apply><ml:lessThan /><ml:apply><ml:id xml:space=\"preserve\">last</ml:id><ml:id xml:space=\"preserve\"><Span xmlns=\"http://schemas.microsoft.com/winfx/2006/xaml/presentation\" xmlns:pw=\"clr-namespace:Ptc.Wpf;assembly=Ptc.Core\">AC<pw:Subscript>EntranceTank</pw:Subscript></Span></ml:id></ml:apply><ml:real>1796</ml:real></ml:apply></ml:test><ml:then><ml:program><ml:apply><ml:id xml:space=\"preserve\">submatrix</ml:id><ml:sequence><ml:id xml:space=\"preserve\"><Span xmlns=\"http://schemas.microsoft.com/winfx/2006/xaml/presentation\" xmlns:pw=\"clr-namespace:Ptc.Wpf;assembly=Ptc.Core\">AC<pw:Subscript>EntranceTank</pw:Subscript></Span></ml:id><ml:real>1198</ml:real><ml:apply><ml:id xml:space=\"preserve\">last</ml:id><ml:id xml:space=\"preserve\"><Span xmlns=\"http://schemas.microsoft.com/winfx/2006/xaml/presentation\" xmlns:pw=\"clr-namespace:Ptc.Wpf;assembly=Ptc.Core\">AC<pw:Subscript>EntranceTank</pw:Subscript></Span></ml:id></ml:apply><ml:real>0</ml:real><ml:real>0</ml:real></ml:sequence></ml:apply></ml:program></ml:then><ml:else><ml:program><ml:apply><ml:id xml:space=\"preserve\">submatrix</ml:id><ml:sequence><ml:id xml:space=\"preserve\"><Span xmlns=\"http://schemas.microsoft.com/winfx/2006/xaml/presentation\" xmlns:pw=\"clr-namespace:Ptc.Wpf;assembly=Ptc.Core\">AC<pw:Subscript>EntranceTank</pw:Subscript></Span></ml:id><ml:real>1198</ml:real><ml:real>1796</ml:real><ml:real>0</ml:real><ml:real>0</ml:real></ml:sequence></ml:apply></ml:program></ml:else></ml:if></ml:program></ml:define></math><mc14-conversion-loss-annotations><annotation>Otherwise</annotation></mc14-conversion-loss-annotations></region><region top=\"14780.1611\" width=\"452\" left=\"67.2\" height=\"49\" converted-from=\"Mathcad14\" region-id=\"388\"><math><ml:define><ml:id label=\"Variable\" xml:space=\"preserve\"><Span xmlns=\"http://schemas.microsoft.com/winfx/2006/xaml/presentation\" xmlns:pw=\"clr-namespace:Ptc.Wpf;assembly=Ptc.Core\">AC<pw:Subscript>OperatorAccessA</pw:Subscript></Span></ml:id><ml:program><ml:if><ml:test><ml:apply><ml:lessThan /><ml:apply><ml:id xml:space=\"preserve\">last</ml:id><ml:id xml:space=\"preserve\"><Span xmlns=\"http://schemas.microsoft.com/winfx/2006/xaml/presentation\" xmlns:pw=\"clr-namespace:Ptc.Wpf;assembly=Ptc.Core\">AC<pw:Subscript>OperatorAccess</pw:Subscript></Span></ml:id></ml:apply><ml:real>598</ml:real></ml:apply></ml:test><ml:then><ml:program><ml:id xml:space=\"preserve\"><Span xmlns=\"http://schemas.microsoft.com/winfx/2006/xaml/presentation\" xmlns:pw=\"clr-namespace:Ptc.Wpf;assembly=Ptc.Core\">AC<pw:Subscript>OperatorAccess</pw:Subscript></Span></ml:id></ml:program></ml:then><ml:else><ml:program><ml:apply><ml:id xml:space=\"preserve\">submatrix</ml:id><ml:sequence><ml:id xml:space=\"preserve\"><Span xmlns=\"http://schemas.microsoft.com/winfx/2006/xaml/presentation\" xmlns:pw=\"clr-namespace:Ptc.Wpf;assembly=Ptc.Core\">AC<pw:Subscript>OperatorAccess</pw:Subscript></Span></ml:id><ml:real>0</ml:real><ml:real>598</ml:real><ml:real>0</ml:real><ml:real>0</ml:real></ml:sequence></ml:apply></ml:program></ml:else></ml:if></ml:program></ml:define></math><mc14-conversion-loss-annotations><annotation>Otherwise</annotation></mc14-conversion-loss-annotations></region><region top=\"14866.5605\" width=\"705\" left=\"67.2\" height=\"49\" converted-from=\"Mathcad14\" region-id=\"389\"><math><ml:define><ml:id label=\"Variable\" xml:space=\"preserve\"><Span xmlns=\"http://schemas.microsoft.com/winfx/2006/xaml/presentation\" xmlns:pw=\"clr-namespace:Ptc.Wpf;assembly=Ptc.Core\">AC<pw:Subscript>OperatorAccessB</pw:Subscript></Span></ml:id><ml:program><ml:if><ml:test><ml:apply><ml:lessThan /><ml:apply><ml:id xml:space=\"preserve\">last</ml:id><ml:id xml:space=\"preserve\"><Span xmlns=\"http://schemas.microsoft.com/winfx/2006/xaml/presentation\" xmlns:pw=\"clr-namespace:Ptc.Wpf;assembly=Ptc.Core\">AC<pw:Subscript>OperatorAccess</pw:Subscript></Span></ml:id></ml:apply><ml:real>1197</ml:real></ml:apply></ml:test><ml:then><ml:program><ml:apply><ml:id xml:space=\"preserve\">submatrix</ml:id><ml:sequence><ml:id xml:space=\"preserve\"><Span xmlns=\"http://schemas.microsoft.com/winfx/2006/xaml/presentation\" xmlns:pw=\"clr-namespace:Ptc.Wpf;assembly=Ptc.Core\">AC<pw:Subscript>OperatorAccess</pw:Subscript></Span></ml:id><ml:real>599</ml:real><ml:apply><ml:id xml:space=\"preserve\">last</ml:id><ml:id xml:space=\"preserve\"><Span xmlns=\"http://schemas.microsoft.com/winfx/2006/xaml/presentation\" xmlns:pw=\"clr-namespace:Ptc.Wpf;assembly=Ptc.Core\">AC<pw:Subscript>OperatorAccess</pw:Subscript></Span></ml:id></ml:apply><ml:real>0</ml:real><ml:real>0</ml:real></ml:sequence></ml:apply></ml:program></ml:then><ml:else><ml:program><ml:apply><ml:id xml:space=\"preserve\">submatrix</ml:id><ml:sequence><ml:id xml:space=\"preserve\"><Span xmlns=\"http://schemas.microsoft.com/winfx/2006/xaml/presentation\" xmlns:pw=\"clr-namespace:Ptc.Wpf;assembly=Ptc.Core\">AC<pw:Subscript>OperatorAccess</pw:Subscript></Span></ml:id><ml:real>599</ml:real><ml:real>1197</ml:real><ml:real>0</ml:real><ml:real>0</ml:real></ml:sequence></ml:apply></ml:program></ml:else></ml:if></ml:program></ml:define></math><mc14-conversion-loss-annotations><annotation>Otherwise</annotation></mc14-conversion-loss-annotations></region><region top=\"14972.1611\" width=\"711\" left=\"67.2\" height=\"49\" converted-from=\"Mathcad14\" region-id=\"390\"><math><ml:define><ml:id label=\"Variable\" xml:space=\"preserve\"><Span xmlns=\"http://schemas.microsoft.com/winfx/2006/xaml/presentation\" xmlns:pw=\"clr-namespace:Ptc.Wpf;assembly=Ptc.Core\">AC<pw:Subscript>OperatorAccessC</pw:Subscript></Span></ml:id><ml:program><ml:if><ml:test><ml:apply><ml:lessThan /><ml:apply><ml:id xml:space=\"preserve\">last</ml:id><ml:id xml:space=\"preserve\"><Span xmlns=\"http://schemas.microsoft.com/winfx/2006/xaml/presentation\" xmlns:pw=\"clr-namespace:Ptc.Wpf;assembly=Ptc.Core\">AC<pw:Subscript>OperatorAccess</pw:Subscript></Span></ml:id></ml:apply><ml:real>1796</ml:real></ml:apply></ml:test><ml:then><ml:program><ml:apply><ml:id xml:space=\"preserve\">submatrix</ml:id><ml:sequence><ml:id xml:space=\"preserve\"><Span xmlns=\"http://schemas.microsoft.com/winfx/2006/xaml/presentation\" xmlns:pw=\"clr-namespace:Ptc.Wpf;assembly=Ptc.Core\">AC<pw:Subscript>OperatorAccess</pw:Subscript></Span></ml:id><ml:real>1198</ml:real><ml:apply><ml:id xml:space=\"preserve\">last</ml:id><ml:id xml:space=\"preserve\"><Span xmlns=\"http://schemas.microsoft.com/winfx/2006/xaml/presentation\" xmlns:pw=\"clr-namespace:Ptc.Wpf;assembly=Ptc.Core\">AC<pw:Subscript>OperatorAccess</pw:Subscript></Span></ml:id></ml:apply><ml:real>0</ml:real><ml:real>0</ml:real></ml:sequence></ml:apply></ml:program></ml:then><ml:else><ml:program><ml:apply><ml:id xml:space=\"preserve\">submatrix</ml:id><ml:sequence><ml:id xml:space=\"preserve\"><Span xmlns=\"http://schemas.microsoft.com/winfx/2006/xaml/presentation\" xmlns:pw=\"clr-namespace:Ptc.Wpf;assembly=Ptc.Core\">AC<pw:Subscript>OperatorAccess</pw:Subscript></Span></ml:id><ml:real>1198</ml:real><ml:real>1796</ml:real><ml:real>0</ml:real><ml:real>0</ml:real></ml:sequence></ml:apply></ml:program></ml:else></ml:if></ml:program></ml:define></math><mc14-conversion-loss-annotations><annotation>Otherwise</annotation></mc14-conversion-loss-annotations></region><region top=\"15212.1611\" width=\"359\" left=\"864\" height=\"45\" converted-from=\"Mathcad14\" region-id=\"391\"><math><ml:define><ml:id label=\"Variable\" xml:space=\"preserve\"><Span xmlns=\"http://schemas.microsoft.com/winfx/2006/xaml/presentation\" xmlns:pw=\"clr-namespace:Ptc.Wpf;assembly=Ptc.Core\">AC<pw:Subscript>ZZMatApplyA</pw:Subscript></Span></ml:id><ml:program><ml:if><ml:test><ml:apply><ml:lessThan /><ml:apply><ml:id xml:space=\"preserve\">last</ml:id><ml:id xml:space=\"preserve\"><Span xmlns=\"http://schemas.microsoft.com/winfx/2006/xaml/presentation\" xmlns:pw=\"clr-namespace:Ptc.Wpf;assembly=Ptc.Core\">AC<pw:Subscript>MatApply</pw:Subscript></Span></ml:id></ml:apply><ml:real>598</ml:real></ml:apply></ml:test><ml:then><ml:program><ml:id xml:space=\"preserve\"><Span xmlns=\"http://schemas.microsoft.com/winfx/2006/xaml/presentation\" xmlns:pw=\"clr-namespace:Ptc.Wpf;assembly=Ptc.Core\">AC<pw:Subscript>MatApply</pw:Subscript></Span></ml:id></ml:program></ml:then><ml:else><ml:program><ml:apply><ml:id xml:space=\"preserve\">submatrix</ml:id><ml:sequence><ml:id xml:space=\"preserve\"><Span xmlns=\"http://schemas.microsoft.com/winfx/2006/xaml/presentation\" xmlns:pw=\"clr-namespace:Ptc.Wpf;assembly=Ptc.Core\">AC<pw:Subscript>MatApply</pw:Subscript></Span></ml:id><ml:real>0</ml:real><ml:real>598</ml:real><ml:real>0</ml:real><ml:real>0</ml:real></ml:sequence></ml:apply></ml:program></ml:else></ml:if></ml:program></ml:define></math><mc14-conversion-loss-annotations><annotation>Otherwise</annotation></mc14-conversion-loss-annotations></region><region top=\"15250.5605\" width=\"360\" left=\"67.2\" height=\"49\" converted-from=\"Mathcad14\" region-id=\"392\"><math><ml:define><ml:id label=\"Variable\" xml:space=\"preserve\"><Span xmlns=\"http://schemas.microsoft.com/winfx/2006/xaml/presentation\" xmlns:pw=\"clr-namespace:Ptc.Wpf;assembly=Ptc.Core\">AC<pw:Subscript>ZZLayoutA</pw:Subscript></Span></ml:id><ml:program><ml:if><ml:test><ml:apply><ml:lessThan /><ml:apply><ml:id xml:space=\"preserve\">last</ml:id><ml:id xml:space=\"preserve\"><Span xmlns=\"http://schemas.microsoft.com/winfx/2006/xaml/presentation\" xmlns:pw=\"clr-namespace:Ptc.Wpf;assembly=Ptc.Core\">AC<pw:Subscript>Layout</pw:Subscript></Span></ml:id></ml:apply><ml:real>598</ml:real></ml:apply></ml:test><ml:then><ml:program><ml:id xml:space=\"preserve\"><Span xmlns=\"http://schemas.microsoft.com/winfx/2006/xaml/presentation\" xmlns:pw=\"clr-namespace:Ptc.Wpf;assembly=Ptc.Core\">AC<pw:Subscript>Layout</pw:Subscript></Span></ml:id></ml:program></ml:then><ml:else><ml:program><ml:apply><ml:id xml:space=\"preserve\">submatrix</ml:id><ml:sequence><ml:id xml:space=\"preserve\"><Span xmlns=\"http://schemas.microsoft.com/winfx/2006/xaml/presentation\" xmlns:pw=\"clr-namespace:Ptc.Wpf;assembly=Ptc.Core\">AC<pw:Subscript>Layout</pw:Subscript></Span></ml:id><ml:real>0</ml:real><ml:real>598</ml:real><ml:real>0</ml:real><ml:real>0</ml:real></ml:sequence></ml:apply></ml:program></ml:else></ml:if></ml:program></ml:define></math><mc14-conversion-loss-annotations><annotation>Otherwise</annotation></mc14-conversion-loss-annotations></region><region top=\"15336.9609\" width=\"603\" left=\"854.4\" height=\"49\" converted-from=\"Mathcad14\" region-id=\"393\"><math><ml:define><ml:id label=\"Variable\" xml:space=\"preserve\"><Span xmlns=\"http://schemas.microsoft.com/winfx/2006/xaml/presentation\" xmlns:pw=\"clr-namespace:Ptc.Wpf;assembly=Ptc.Core\">AC<pw:Subscript>ZZMatApplyB</pw:Subscript></Span></ml:id><ml:program><ml:if><ml:test><ml:apply><ml:lessThan /><ml:apply><ml:id xml:space=\"preserve\">last</ml:id><ml:id xml:space=\"preserve\"><Span xmlns=\"http://schemas.microsoft.com/winfx/2006/xaml/presentation\" xmlns:pw=\"clr-namespace:Ptc.Wpf;assembly=Ptc.Core\">AC<pw:Subscript>MatApply</pw:Subscript></Span></ml:id></ml:apply><ml:real>1197</ml:real></ml:apply></ml:test><ml:then><ml:program><ml:apply><ml:id xml:space=\"preserve\">submatrix</ml:id><ml:sequence><ml:id xml:space=\"preserve\"><Span xmlns=\"http://schemas.microsoft.com/winfx/2006/xaml/presentation\" xmlns:pw=\"clr-namespace:Ptc.Wpf;assembly=Ptc.Core\">AC<pw:Subscript>MatApply</pw:Subscript></Span></ml:id><ml:real>1198</ml:real><ml:apply><ml:id xml:space=\"preserve\">last</ml:id><ml:id xml:space=\"preserve\"><Span xmlns=\"http://schemas.microsoft.com/winfx/2006/xaml/presentation\" xmlns:pw=\"clr-namespace:Ptc.Wpf;assembly=Ptc.Core\">AC<pw:Subscript>MatApply</pw:Subscript></Span></ml:id></ml:apply><ml:real>0</ml:real><ml:real>0</ml:real></ml:sequence></ml:apply></ml:program></ml:then><ml:else><ml:program><ml:apply><ml:id xml:space=\"preserve\">submatrix</ml:id><ml:sequence><ml:id xml:space=\"preserve\"><Span xmlns=\"http://schemas.microsoft.com/winfx/2006/xaml/presentation\" xmlns:pw=\"clr-namespace:Ptc.Wpf;assembly=Ptc.Core\">AC<pw:Subscript>MatApply</pw:Subscript></Span></ml:id><ml:real>1198</ml:real><ml:real>1796</ml:real><ml:real>0</ml:real><ml:real>0</ml:real></ml:sequence></ml:apply></ml:program></ml:else></ml:if></ml:program></ml:define></math><mc14-conversion-loss-annotations><annotation>Otherwise</annotation></mc14-conversion-loss-annotations></region><region top=\"15346.5605\" width=\"531\" left=\"67.2\" height=\"49\" converted-from=\"Mathcad14\" region-id=\"394\"><math><ml:define><ml:id label=\"Variable\" xml:space=\"preserve\"><Span xmlns=\"http://schemas.microsoft.com/winfx/2006/xaml/presentation\" xmlns:pw=\"clr-namespace:Ptc.Wpf;assembly=Ptc.Core\">AC<pw:Subscript>ZZLayoutB</pw:Subscript></Span></ml:id><ml:program><ml:if><ml:test><ml:apply><ml:lessThan /><ml:apply><ml:id xml:space=\"preserve\">last</ml:id><ml:id xml:space=\"preserve\"><Span xmlns=\"http://schemas.microsoft.com/winfx/2006/xaml/presentation\" xmlns:pw=\"clr-namespace:Ptc.Wpf;assembly=Ptc.Core\">AC<pw:Subscript>Layout</pw:Subscript></Span></ml:id></ml:apply><ml:real>1197</ml:real></ml:apply></ml:test><ml:then><ml:program><ml:apply><ml:id xml:space=\"preserve\">submatrix</ml:id><ml:sequence><ml:id xml:space=\"preserve\"><Span xmlns=\"http://schemas.microsoft.com/winfx/2006/xaml/presentation\" xmlns:pw=\"clr-namespace:Ptc.Wpf;assembly=Ptc.Core\">AC<pw:Subscript>Layout</pw:Subscript></Span></ml:id><ml:real>1198</ml:real><ml:apply><ml:id xml:space=\"preserve\">last</ml:id><ml:id xml:space=\"preserve\"><Span xmlns=\"http://schemas.microsoft.com/winfx/2006/xaml/presentation\" xmlns:pw=\"clr-namespace:Ptc.Wpf;assembly=Ptc.Core\">AC<pw:Subscript>Layout</pw:Subscript></Span></ml:id></ml:apply><ml:real>0</ml:real><ml:real>0</ml:real></ml:sequence></ml:apply></ml:program></ml:then><ml:else><ml:program><ml:apply><ml:id xml:space=\"preserve\">submatrix</ml:id><ml:sequence><ml:id xml:space=\"preserve\"><Span xmlns=\"http://schemas.microsoft.com/winfx/2006/xaml/presentation\" xmlns:pw=\"clr-namespace:Ptc.Wpf;assembly=Ptc.Core\">AC<pw:Subscript>Layout</pw:Subscript></Span></ml:id><ml:real>1198</ml:real><ml:real>1796</ml:real><ml:real>0</ml:real><ml:real>0</ml:real></ml:sequence></ml:apply></ml:program></ml:else></ml:if></ml:program></ml:define></math><mc14-conversion-loss-annotations><annotation>Otherwise</annotation></mc14-conversion-loss-annotations></region><region top=\"15452.1611\" width=\"531\" left=\"67.2\" height=\"49\" converted-from=\"Mathcad14\" region-id=\"395\"><math><ml:define><ml:id label=\"Variable\" xml:space=\"preserve\"><Span xmlns=\"http://schemas.microsoft.com/winfx/2006/xaml/presentation\" xmlns:pw=\"clr-namespace:Ptc.Wpf;assembly=Ptc.Core\">AC<pw:Subscript>ZZLayoutC</pw:Subscript></Span></ml:id><ml:program><ml:if><ml:test><ml:apply><ml:lessThan /><ml:apply><ml:id xml:space=\"preserve\">last</ml:id><ml:id xml:space=\"preserve\"><Span xmlns=\"http://schemas.microsoft.com/winfx/2006/xaml/presentation\" xmlns:pw=\"clr-namespace:Ptc.Wpf;assembly=Ptc.Core\">AC<pw:Subscript>Layout</pw:Subscript></Span></ml:id></ml:apply><ml:real>1796</ml:real></ml:apply></ml:test><ml:then><ml:program><ml:apply><ml:id xml:space=\"preserve\">submatrix</ml:id><ml:sequence><ml:id xml:space=\"preserve\"><Span xmlns=\"http://schemas.microsoft.com/winfx/2006/xaml/presentation\" xmlns:pw=\"clr-namespace:Ptc.Wpf;assembly=Ptc.Core\">AC<pw:Subscript>Layout</pw:Subscript></Span></ml:id><ml:real>1198</ml:real><ml:apply><ml:id xml:space=\"preserve\">last</ml:id><ml:id xml:space=\"preserve\"><Span xmlns=\"http://schemas.microsoft.com/winfx/2006/xaml/presentation\" xmlns:pw=\"clr-namespace:Ptc.Wpf;assembly=Ptc.Core\">AC<pw:Subscript>Layout</pw:Subscript></Span></ml:id></ml:apply><ml:real>0</ml:real><ml:real>0</ml:real></ml:sequence></ml:apply></ml:program></ml:then><ml:else><ml:program><ml:apply><ml:id xml:space=\"preserve\">submatrix</ml:id><ml:sequence><ml:id xml:space=\"preserve\"><Span xmlns=\"http://schemas.microsoft.com/winfx/2006/xaml/presentation\" xmlns:pw=\"clr-namespace:Ptc.Wpf;assembly=Ptc.Core\">AC<pw:Subscript>Layout</pw:Subscript></Span></ml:id><ml:real>1198</ml:real><ml:real>1796</ml:real><ml:real>0</ml:real><ml:real>0</ml:real></ml:sequence></ml:apply></ml:program></ml:else></ml:if></ml:program></ml:define></math><mc14-conversion-loss-annotations><annotation>Otherwise</annotation></mc14-conversion-loss-annotations></region><region top=\"15452.1611\" width=\"603\" left=\"854.4\" height=\"49\" converted-from=\"Mathcad14\" region-id=\"396\"><math><ml:define><ml:id label=\"Variable\" xml:space=\"preserve\"><Span xmlns=\"http://schemas.microsoft.com/winfx/2006/xaml/presentation\" xmlns:pw=\"clr-namespace:Ptc.Wpf;assembly=Ptc.Core\">AC<pw:Subscript>ZZMatApplyC</pw:Subscript></Span></ml:id><ml:program><ml:if><ml:test><ml:apply><ml:lessThan /><ml:apply><ml:id xml:space=\"preserve\">last</ml:id><ml:id xml:space=\"preserve\"><Span xmlns=\"http://schemas.microsoft.com/winfx/2006/xaml/presentation\" xmlns:pw=\"clr-namespace:Ptc.Wpf;assembly=Ptc.Core\">AC<pw:Subscript>MatApply</pw:Subscript></Span></ml:id></ml:apply><ml:real>1796</ml:real></ml:apply></ml:test><ml:then><ml:program><ml:apply><ml:id xml:space=\"preserve\">submatrix</ml:id><ml:sequence><ml:id xml:space=\"preserve\"><Span xmlns=\"http://schemas.microsoft.com/winfx/2006/xaml/presentation\" xmlns:pw=\"clr-namespace:Ptc.Wpf;assembly=Ptc.Core\">AC<pw:Subscript>MatApply</pw:Subscript></Span></ml:id><ml:real>1198</ml:real><ml:apply><ml:id xml:space=\"preserve\">last</ml:id><ml:id xml:space=\"preserve\"><Span xmlns=\"http://schemas.microsoft.com/winfx/2006/xaml/presentation\" xmlns:pw=\"clr-namespace:Ptc.Wpf;assembly=Ptc.Core\">AC<pw:Subscript>MatApply</pw:Subscript></Span></ml:id></ml:apply><ml:real>0</ml:real><ml:real>0</ml:real></ml:sequence></ml:apply></ml:program></ml:then><ml:else><ml:program><ml:apply><ml:id xml:space=\"preserve\">submatrix</ml:id><ml:sequence><ml:id xml:space=\"preserve\"><Span xmlns=\"http://schemas.microsoft.com/winfx/2006/xaml/presentation\" xmlns:pw=\"clr-namespace:Ptc.Wpf;assembly=Ptc.Core\">AC<pw:Subscript>MatApply</pw:Subscript></Span></ml:id><ml:real>1198</ml:real><ml:real>1796</ml:real><ml:real>0</ml:real><ml:real>0</ml:real></ml:sequence></ml:apply></ml:program></ml:else></ml:if></ml:program></ml:define></math><mc14-conversion-loss-annotations><annotation>Otherwise</annotation></mc14-conversion-loss-annotations></region><region top=\"15561.3613\" width=\"832\" left=\"0\" height=\"19.2\" region-id=\"397\"><text is-text-block=\"true\"><FlowDocument FontFamily=\"Mathcad UniMath\" xmlns=\"http://schemas.microsoft.com/winfx/2006/xaml/presentation\"><Paragraph xml:space=\"preserve\">---↑  ---</Paragraph></FlowDocument></text></region><region top=\"15670.8\" width=\"202\" left=\"9.6\" height=\"21\" converted-from=\"Mathcad14\" region-id=\"398\"><text><FlowDocument FontFamily=\"Tahoma\" FontStyle=\"Normal\" FontWeight=\"Normal\" FontSize=\"14.6666666666667\" Foreground=\"#FF000000\" Background=\"#00FFFFFF\" PagePadding=\"5,0,5,0\" AllowDrop=\"True\" Typography.Variants=\"Normal\" xmlns=\"http://schemas.microsoft.com/winfx/2006/xaml/presentation\"><Paragraph TextAlignment=\"Left\"><Run FontFamily=\"Arial\" FontStyle=\"Normal\" FontWeight=\"Bold\" FontSize=\"18.6666666666667\" Typography.Variants=\"Normal\"><Run.TextDecorations><TextDecorationCollection /></Run.TextDecorations>Display AC variables</Run></Paragraph></FlowDocument></text></region><region top=\"15709.2\" width=\"832\" left=\"0\" height=\"19.2\" region-id=\"399\"><text is-text-block=\"true\"><FlowDocument FontFamily=\"Mathcad UniMath\" xmlns=\"http://schemas.microsoft.com/winfx/2006/xaml/presentation\"><Paragraph xml:space=\"preserve\">---↓  ---</Paragraph></FlowDocument></text><mc14-conversion-loss-annotations><annotation>CollapsedArea</annotation></mc14-conversion-loss-annotations></region><region top=\"15828.24\" width=\"133\" left=\"9.6\" height=\"22\" converted-from=\"Mathcad14\" region-id=\"400\"><math><ml:eval><ml:id xml:space=\"preserve\"><Span xmlns=\"http://schemas.microsoft.com/winfx/2006/xaml/presentation\" xmlns:pw=\"clr-namespace:Ptc.Wpf;assembly=Ptc.Core\">AC<pw:Subscript>EntranceTankA</pw:Subscript></Span></ml:id><ml:result /></ml:eval><resultFormat><table /></resultFormat></math></region><region top=\"15972.24\" width=\"131\" left=\"681.6\" height=\"22\" converted-from=\"Mathcad14\" region-id=\"401\"><math><ml:eval><ml:id xml:space=\"preserve\"><Span xmlns=\"http://schemas.microsoft.com/winfx/2006/xaml/presentation\" xmlns:pw=\"clr-namespace:Ptc.Wpf;assembly=Ptc.Core\">AC<pw:Subscript>EntranceTankB</pw:Subscript></Span></ml:id><ml:result /></ml:eval><resultFormat><table /></resultFormat></math></region><region top=\"16049.041\" width=\"131\" left=\"1113.6\" height=\"22\" converted-from=\"Mathcad14\" region-id=\"402\"><math><ml:eval><ml:id xml:space=\"preserve\"><Span xmlns=\"http://schemas.microsoft.com/winfx/2006/xaml/presentation\" xmlns:pw=\"clr-namespace:Ptc.Wpf;assembly=Ptc.Core\">AC<pw:Subscript>EntranceTankC</pw:Subscript></Span></ml:id><ml:result /></ml:eval></math></region><region top=\"16202.6406\" width=\"109\" left=\"67.2\" height=\"22\" converted-from=\"Mathcad14\" region-id=\"403\"><math><ml:eval><ml:id xml:space=\"preserve\"><Span xmlns=\"http://schemas.microsoft.com/winfx/2006/xaml/presentation\" xmlns:pw=\"clr-namespace:Ptc.Wpf;assembly=Ptc.Core\">AC<pw:Subscript>FlocTankA</pw:Subscript></Span></ml:id><ml:result /></ml:eval><resultFormat><table /></resultFormat></math></region><region top=\"16308.24\" width=\"107\" left=\"566.4\" height=\"22\" converted-from=\"Mathcad14\" region-id=\"404\"><math><ml:eval><ml:id xml:space=\"preserve\"><Span xmlns=\"http://schemas.microsoft.com/winfx/2006/xaml/presentation\" xmlns:pw=\"clr-namespace:Ptc.Wpf;assembly=Ptc.Core\">AC<pw:Subscript>FlocTankB</pw:Subscript></Span></ml:id><ml:result /></ml:eval><resultFormat><table /></resultFormat></math></region><region top=\"16365.8408\" width=\"108\" left=\"1468.8\" height=\"22\" converted-from=\"Mathcad14\" region-id=\"405\"><math><ml:eval><ml:id xml:space=\"preserve\"><Span xmlns=\"http://schemas.microsoft.com/winfx/2006/xaml/presentation\" xmlns:pw=\"clr-namespace:Ptc.Wpf;assembly=Ptc.Core\">AC<pw:Subscript>FlocTankD</pw:Subscript></Span></ml:id><ml:result /></ml:eval></math></region><region top=\"16423.4414\" width=\"107\" left=\"892.8\" height=\"22\" converted-from=\"Mathcad14\" region-id=\"406\"><math><ml:eval><ml:id xml:space=\"preserve\"><Span xmlns=\"http://schemas.microsoft.com/winfx/2006/xaml/presentation\" xmlns:pw=\"clr-namespace:Ptc.Wpf;assembly=Ptc.Core\">AC<pw:Subscript>FlocTankC</pw:Subscript></Span></ml:id><ml:result /></ml:eval></math></region><region top=\"16529.041\" width=\"146\" left=\"57.6\" height=\"22\" converted-from=\"Mathcad14\" region-id=\"407\"><math><ml:eval><ml:id xml:space=\"preserve\"><Span xmlns=\"http://schemas.microsoft.com/winfx/2006/xaml/presentation\" xmlns:pw=\"clr-namespace:Ptc.Wpf;assembly=Ptc.Core\">AC<pw:Subscript>OperatorAccessA</pw:Subscript></Span></ml:id><ml:result /></ml:eval><resultFormat><table /></resultFormat></math></region><region top=\"16529.041\" width=\"144\" left=\"1190.4\" height=\"22\" converted-from=\"Mathcad14\" region-id=\"408\"><math><ml:eval><ml:id xml:space=\"preserve\"><Span xmlns=\"http://schemas.microsoft.com/winfx/2006/xaml/presentation\" xmlns:pw=\"clr-namespace:Ptc.Wpf;assembly=Ptc.Core\">AC<pw:Subscript>OperatorAccessC</pw:Subscript></Span></ml:id><ml:result /></ml:eval><resultFormat><table /></resultFormat></math></region><region top=\"16577.041\" width=\"144\" left=\"652.8\" height=\"22\" converted-from=\"Mathcad14\" region-id=\"409\"><math><ml:eval><ml:id xml:space=\"preserve\"><Span xmlns=\"http://schemas.microsoft.com/winfx/2006/xaml/presentation\" xmlns:pw=\"clr-namespace:Ptc.Wpf;assembly=Ptc.Core\">AC<pw:Subscript>OperatorAccessB</pw:Subscript></Span></ml:id><ml:result /></ml:eval><resultFormat><table /></resultFormat></math></region><region top=\"16797.84\" width=\"106\" left=\"28.8\" height=\"22\" converted-from=\"Mathcad14\" region-id=\"410\"><math><ml:eval><ml:id xml:space=\"preserve\"><Span xmlns=\"http://schemas.microsoft.com/winfx/2006/xaml/presentation\" xmlns:pw=\"clr-namespace:Ptc.Wpf;assembly=Ptc.Core\">AC<pw:Subscript>SedTankA</pw:Subscript></Span></ml:id><ml:result /></ml:eval><resultFormat><table /></resultFormat></math></region><region top=\"16797.84\" width=\"104\" left=\"672\" height=\"22\" converted-from=\"Mathcad14\" region-id=\"411\"><math><ml:eval><ml:id xml:space=\"preserve\"><Span xmlns=\"http://schemas.microsoft.com/winfx/2006/xaml/presentation\" xmlns:pw=\"clr-namespace:Ptc.Wpf;assembly=Ptc.Core\">AC<pw:Subscript>SedTankB</pw:Subscript></Span></ml:id><ml:result /></ml:eval><resultFormat><table /></resultFormat></math></region><region top=\"16807.4414\" width=\"104\" left=\"1228.8\" height=\"22\" converted-from=\"Mathcad14\" region-id=\"412\"><math><ml:eval><ml:id xml:space=\"preserve\"><Span xmlns=\"http://schemas.microsoft.com/winfx/2006/xaml/presentation\" xmlns:pw=\"clr-namespace:Ptc.Wpf;assembly=Ptc.Core\">AC<pw:Subscript>SedTankC</pw:Subscript></Span></ml:id><ml:result /></ml:eval><resultFormat><table /></resultFormat></math></region><region top=\"17095.4414\" width=\"122\" left=\"28.8\" height=\"22\" converted-from=\"Mathcad14\" region-id=\"413\"><math><ml:eval><ml:id xml:space=\"preserve\"><Span xmlns=\"http://schemas.microsoft.com/winfx/2006/xaml/presentation\" xmlns:pw=\"clr-namespace:Ptc.Wpf;assembly=Ptc.Core\">AC<pw:Subscript>ChemTanksA</pw:Subscript></Span></ml:id><ml:result /></ml:eval><resultFormat><table /></resultFormat></math></region><region top=\"17105.041\" width=\"120\" left=\"681.6\" height=\"22\" converted-from=\"Mathcad14\" region-id=\"414\"><math><ml:eval><ml:id xml:space=\"preserve\"><Span xmlns=\"http://schemas.microsoft.com/winfx/2006/xaml/presentation\" xmlns:pw=\"clr-namespace:Ptc.Wpf;assembly=Ptc.Core\">AC<pw:Subscript>ChemTanksB</pw:Subscript></Span></ml:id><ml:result /></ml:eval><resultFormat><table /></resultFormat></math></region><region top=\"17133.84\" width=\"120\" left=\"1209.6\" height=\"22\" converted-from=\"Mathcad14\" region-id=\"415\"><math><ml:eval><ml:id xml:space=\"preserve\"><Span xmlns=\"http://schemas.microsoft.com/winfx/2006/xaml/presentation\" xmlns:pw=\"clr-namespace:Ptc.Wpf;assembly=Ptc.Core\">AC<pw:Subscript>ChemTanksC</pw:Subscript></Span></ml:id><ml:result /></ml:eval></math></region><region top=\"17201.041\" width=\"132\" left=\"28.8\" height=\"22\" converted-from=\"Mathcad14\" region-id=\"416\"><math><ml:eval><ml:id xml:space=\"preserve\"><Span xmlns=\"http://schemas.microsoft.com/winfx/2006/xaml/presentation\" xmlns:pw=\"clr-namespace:Ptc.Wpf;assembly=Ptc.Core\">AC<pw:Subscript>DrainChannelA</pw:Subscript></Span></ml:id><ml:result /></ml:eval><resultFormat><table /></resultFormat></math></region><region top=\"17210.64\" width=\"130\" left=\"672\" height=\"22\" converted-from=\"Mathcad14\" region-id=\"417\"><math><ml:eval><ml:id xml:space=\"preserve\"><Span xmlns=\"http://schemas.microsoft.com/winfx/2006/xaml/presentation\" xmlns:pw=\"clr-namespace:Ptc.Wpf;assembly=Ptc.Core\">AC<pw:Subscript>DrainChannelB</pw:Subscript></Span></ml:id><ml:result /></ml:eval></math></region><region top=\"17210.64\" width=\"130\" left=\"1209.6\" height=\"22\" converted-from=\"Mathcad14\" region-id=\"418\"><math><ml:eval><ml:id xml:space=\"preserve\"><Span xmlns=\"http://schemas.microsoft.com/winfx/2006/xaml/presentation\" xmlns:pw=\"clr-namespace:Ptc.Wpf;assembly=Ptc.Core\">AC<pw:Subscript>DrainChannelC</pw:Subscript></Span></ml:id><ml:result /></ml:eval></math></region><region top=\"17441.041\" width=\"122\" left=\"57.6\" height=\"22\" converted-from=\"Mathcad14\" region-id=\"419\"><math><ml:eval><ml:id xml:space=\"preserve\"><Span xmlns=\"http://schemas.microsoft.com/winfx/2006/xaml/presentation\" xmlns:pw=\"clr-namespace:Ptc.Wpf;assembly=Ptc.Core\">AC<pw:Subscript>ZPlantLayout</pw:Subscript></Span></ml:id><ml:result /></ml:eval><resultFormat><table /></resultFormat></math></region><region top=\"17556.24\" width=\"86\" left=\"67.2\" height=\"22\" converted-from=\"Mathcad14\" region-id=\"420\"><math><ml:eval><ml:id xml:space=\"preserve\"><Span xmlns=\"http://schemas.microsoft.com/winfx/2006/xaml/presentation\" xmlns:pw=\"clr-namespace:Ptc.Wpf;assembly=Ptc.Core\">AC<pw:Subscript>FilterA</pw:Subscript></Span></ml:id><ml:result /></ml:eval><resultFormat><table /></resultFormat></math></region><region top=\"17661.84\" width=\"85\" left=\"566.4\" height=\"22\" converted-from=\"Mathcad14\" region-id=\"421\"><math><ml:eval><ml:id xml:space=\"preserve\"><Span xmlns=\"http://schemas.microsoft.com/winfx/2006/xaml/presentation\" xmlns:pw=\"clr-namespace:Ptc.Wpf;assembly=Ptc.Core\">AC<pw:Subscript>FilterD</pw:Subscript></Span></ml:id><ml:result /></ml:eval><resultFormat><table /></resultFormat></math></region><region top=\"17671.4414\" width=\"84\" left=\"28.8\" height=\"22\" converted-from=\"Mathcad14\" region-id=\"422\"><math><ml:eval><ml:id xml:space=\"preserve\"><Span xmlns=\"http://schemas.microsoft.com/winfx/2006/xaml/presentation\" xmlns:pw=\"clr-namespace:Ptc.Wpf;assembly=Ptc.Core\">AC<pw:Subscript>FilterB</pw:Subscript></Span></ml:id><ml:result /></ml:eval><resultFormat><table /></resultFormat></math></region><region top=\"17738.64\" width=\"84\" left=\"38.4\" height=\"22\" converted-from=\"Mathcad14\" region-id=\"423\"><math><ml:eval><ml:id xml:space=\"preserve\"><Span xmlns=\"http://schemas.microsoft.com/winfx/2006/xaml/presentation\" xmlns:pw=\"clr-namespace:Ptc.Wpf;assembly=Ptc.Core\">AC<pw:Subscript>FilterC</pw:Subscript></Span></ml:id><ml:result /></ml:eval><resultFormat><table /></resultFormat></math></region><region top=\"17834.64\" width=\"313\" left=\"326.4\" height=\"48\" converted-from=\"Mathcad14\" region-id=\"424\"><text><FlowDocument FontFamily=\"Tahoma\" FontStyle=\"Normal\" FontWeight=\"Normal\" FontSize=\"14.6666666666667\" Foreground=\"#FF000000\" Background=\"#00FFFFFF\" PagePadding=\"5,0,5,0\" AllowDrop=\"True\" Typography.Variants=\"Normal\" xmlns=\"http://schemas.microsoft.com/winfx/2006/xaml/presentation\"><Paragraph TextAlignment=\"Left\"><Run FontFamily=\"Arial\" FontStyle=\"Normal\" FontWeight=\"Normal\" FontSize=\"13.3333333333333\" Typography.Variants=\"Normal\"><Run.TextDecorations><TextDecorationCollection /></Run.TextDecorations>this variable is displayed to ensure that LabView can read AC.ZZEnd (error in LabView \"read mathcad file\" code that it misses the last variable)</Run></Paragraph></FlowDocument></text></region><region top=\"17844.24\" width=\"74\" left=\"76.8\" height=\"22\" converted-from=\"Mathcad14\" region-id=\"425\"><math><ml:eval><ml:id xml:space=\"preserve\"><Span xmlns=\"http://schemas.microsoft.com/winfx/2006/xaml/presentation\" xmlns:pw=\"clr-namespace:Ptc.Wpf;assembly=Ptc.Core\">HW<pw:Subscript>Sed</pw:Subscript></Span></ml:id><ml:result /></ml:eval></math></region><region top=\"18141.84\" width=\"80\" left=\"86.4\" height=\"22\" converted-from=\"Mathcad14\" region-id=\"426\"><math><ml:eval><ml:id xml:space=\"preserve\"><Span xmlns=\"http://schemas.microsoft.com/winfx/2006/xaml/presentation\" xmlns:pw=\"clr-namespace:Ptc.Wpf;assembly=Ptc.Core\">AC<pw:Subscript>CdcA</pw:Subscript></Span></ml:id><ml:result /></ml:eval><resultFormat><table /></resultFormat></math></region><region top=\"18141.84\" width=\"78\" left=\"864\" height=\"22\" converted-from=\"Mathcad14\" region-id=\"427\"><math><ml:eval><ml:id xml:space=\"preserve\"><Span xmlns=\"http://schemas.microsoft.com/winfx/2006/xaml/presentation\" xmlns:pw=\"clr-namespace:Ptc.Wpf;assembly=Ptc.Core\">AC<pw:Subscript>CdcC</pw:Subscript></Span></ml:id><ml:result /></ml:eval></math></region><region top=\"18151.4414\" width=\"78\" left=\"518.4\" height=\"22\" converted-from=\"Mathcad14\" region-id=\"428\"><math><ml:eval><ml:id xml:space=\"preserve\"><Span xmlns=\"http://schemas.microsoft.com/winfx/2006/xaml/presentation\" xmlns:pw=\"clr-namespace:Ptc.Wpf;assembly=Ptc.Core\">AC<pw:Subscript>CdcB</pw:Subscript></Span></ml:id><ml:result /></ml:eval><resultFormat><table /></resultFormat></math></region><region top=\"18372.24\" width=\"79\" left=\"662.4\" height=\"20\" converted-from=\"Mathcad14\" region-id=\"429\"><math><ml:id xml:space=\"preserve\"><Span xmlns=\"http://schemas.microsoft.com/winfx/2006/xaml/presentation\" xmlns:pw=\"clr-namespace:Ptc.Wpf;assembly=Ptc.Core\">AC<pw:Subscript>ZZMatApplyB</pw:Subscript></Span></ml:id></math></region><region top=\"18381.84\" width=\"79\" left=\"67.2\" height=\"20\" converted-from=\"Mathcad14\" region-id=\"430\"><math><ml:id xml:space=\"preserve\"><Span xmlns=\"http://schemas.microsoft.com/winfx/2006/xaml/presentation\" xmlns:pw=\"clr-namespace:Ptc.Wpf;assembly=Ptc.Core\">AC<pw:Subscript>ZZMatApplyA</pw:Subscript></Span></ml:id></math></region><region top=\"18391.4414\" width=\"79\" left=\"1171.2\" height=\"20\" converted-from=\"Mathcad14\" region-id=\"431\"><math><ml:id xml:space=\"preserve\"><Span xmlns=\"http://schemas.microsoft.com/winfx/2006/xaml/presentation\" xmlns:pw=\"clr-namespace:Ptc.Wpf;assembly=Ptc.Core\">AC<pw:Subscript>ZZMatApplyC</pw:Subscript></Span></ml:id></math></region><region top=\"18506.64\" width=\"113\" left=\"57.6\" height=\"22\" converted-from=\"Mathcad14\" region-id=\"432\"><math><ml:eval><ml:id xml:space=\"preserve\"><Span xmlns=\"http://schemas.microsoft.com/winfx/2006/xaml/presentation\" xmlns:pw=\"clr-namespace:Ptc.Wpf;assembly=Ptc.Core\">AC<pw:Subscript>ZZLayoutA</pw:Subscript></Span></ml:id><ml:result /></ml:eval><resultFormat><table /></resultFormat></math></region><region top=\"18506.64\" width=\"111\" left=\"854.4\" height=\"22\" converted-from=\"Mathcad14\" region-id=\"433\"><math><ml:eval><ml:id xml:space=\"preserve\"><Span xmlns=\"http://schemas.microsoft.com/winfx/2006/xaml/presentation\" xmlns:pw=\"clr-namespace:Ptc.Wpf;assembly=Ptc.Core\">AC<pw:Subscript>ZZLayoutC</pw:Subscript></Span></ml:id><ml:result /></ml:eval></math></region><region top=\"18516.24\" width=\"111\" left=\"451.2\" height=\"22\" converted-from=\"Mathcad14\" region-id=\"434\"><math><ml:eval><ml:id xml:space=\"preserve\"><Span xmlns=\"http://schemas.microsoft.com/winfx/2006/xaml/presentation\" xmlns:pw=\"clr-namespace:Ptc.Wpf;assembly=Ptc.Core\">AC<pw:Subscript>ZZLayoutB</pw:Subscript></Span></ml:id><ml:result /></ml:eval></math></region><region top=\"18567.84\" width=\"832\" left=\"0\" height=\"19.2\" region-id=\"435\"><text is-text-block=\"true\"><FlowDocument FontFamily=\"Mathcad UniMath\" xmlns=\"http://schemas.microsoft.com/winfx/2006/xaml/presentation\"><Paragraph xml:space=\"preserve\">---↑  ---</Paragraph></FlowDocument></text></region><region top=\"18782.8789\" width=\"82\" left=\"38.4\" height=\"45\" converted-from=\"Mathcad14\" region-id=\"436\"><math><ml:eval><ml:id xml:space=\"preserve\"><Span xmlns=\"http://schemas.microsoft.com/winfx/2006/xaml/presentation\" xmlns:pw=\"clr-namespace:Ptc.Wpf;assembly=Ptc.Core\">Q<pw:Subscript>Plant</pw:Subscript></Span></ml:id><ml:unitOverride><ml:apply><ml:div /><ml:apply><ml:pow /><ml:id label=\"Unit\" xml:space=\"preserve\">m</ml:id><ml:real>3</ml:real></ml:apply><ml:id label=\"Unit\" xml:space=\"preserve\">s</ml:id></ml:apply></ml:unitOverride><ml:result /></ml:eval></math></region></regions></worksheet>") -> (9 "XML content":string[](array[string]), 10 "Tag parameters":string[](array[string]))   [LabVIEW 2015]
panel:
  in  "XML Tag":string="resultData"
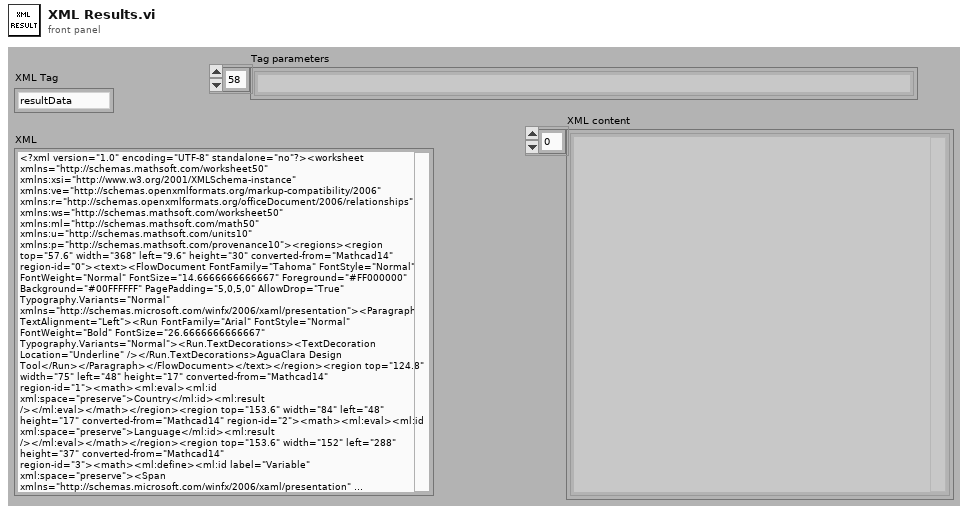
[diagram p1: front panel]
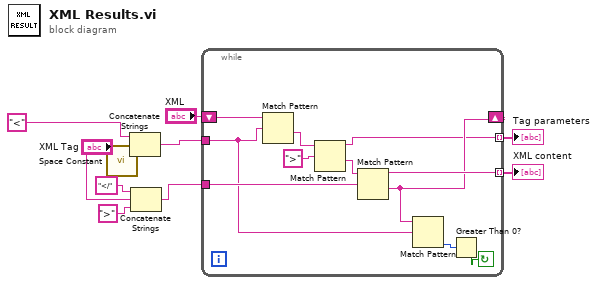
[diagram p0: block diagram]
diagram:
  n1 = call <vilib>:"Space Constant.vi"() -> ("String"=w1:string)
  n2 = Concatenate Strings("<" ("string"), "XML Tag", w1) -> (w9:string)
  n3 = Concatenate Strings("</" ("string"), "XML Tag", ">" ("regular expression")) -> (w5:string)
  n4 = while {
    shift-right: [w16] -> _
    shift-left: "XML" -> [w15]
    tunnel: w9 -> [w12]
    tunnel: w5 -> [w18]
    tunnel: [w17] -> w4 mode=indexing
    tunnel: [w11] -> w2 mode=indexing
    stop <- w13 continue-if-true
    n5 = Match Pattern(string=w15, regular expression=w12) -> (after substring=w21:string)  [unwired: 1 in, 3 out]
    n6 = Match Pattern(string=w21, regular expression=">") -> (before substring=w11:string, after substring=w19:string)  [unwired: 1 in, 2 out]
    n7 = Match Pattern(string=w19, regular expression=w18) -> (before substring=w17:string, after substring=w16:string)  [unwired: 1 in, 2 out]
    n8 = Match Pattern(string=w16, regular expression=w12) -> (offset past match=w14:i32)  [unwired: 1 in, 3 out]
    n9 = Greater Than 0?(x=w14) -> (x > 0?=w13:bool)
  }
  "XML content" <- w4
  "Tag parameters" <- w2
